vi "Gel Tugging Force Mode_Controller v16.20 EPI.vi"() -> ()   [LabVIEW 2015]
doc: "This example demonstrates how to continuously acquire voltage measurements from a DAQmx device using hardware timed, single point reads using a timed loop structure. The timed loop is controlled by the sample clock of the DAQ device. The device will read data on each tick of the sample clock. If an additional sample clock tick occurs before the current data point is read from the device or if the timed loop does not receive any sample clock ticks, a dialog will indicate that this has happened. \n\nHardware Timed Single Point acquisition works best when using a deterministic operating system (such as LabVIEW Real-Time). Because of the less deterministic nature of general purpose operating systems (such as Microsoft Windows), the software loop will not always take the exact same amount of time to execute, and this may lead to the occasional missed sample clock. \n\nFor instructions on how to connect your signals to the DAQ device, refer to your device documentation."
uses:
  <vilib>/Platform/TimedLoop/XDataNode/timing_clust.ctl
  <vilib>/Platform/TimedLoop/XDataNode/nitl_modes.ctl
  <vilib>/Platform/TimedLoop/XDataNode/wakeup.ctl
  <vilib>/dex/Flush And Wait Empty Condition.ctl
  <vilib>/DAQmx/read.llb/DAQmx Read (Analog 1D DBL NChan 1Samp).vi
  <vilib>/DAQmx/write.llb/DAQmx Write (Analog DBL 1Chan 1Samp).vi
  <vilib>/DAQmx/read.llb/DAQmx Read (Analog 2D DBL NChan NSamp).vi
  <vilib>/Analysis/baseanly.llb/Mean (DBL).vi
  <vilib>/DAQmx/create/channels.llb/DAQmx Create Channel (AI-Voltage-Basic).vi
  <vilib>/DAQmx/create/channels.llb/DAQmx Create Channel (AO-Voltage-Basic).vi
  <vilib>/DAQmx/configure/timing.llb/DAQmx Timing (Sample Clock).vi
  <vilib>/DAQmx/create/timing.llb/DAQmx Create Timing Source (Control Loop From Task).vi
  <vilib>/DAQmx/miscellaneous.llb/DAQmx Fill In Error Info.vi
  <vilib>/addons/control/pid/pid.llb/PID (DBL).vi
  <vilib>/addons/control/pid/pid.llb/PID Gain Schedule (DBL).vi
  <vilib>/platform/TimedLoop/XDataNode/XDataNode.xnode
  <vilib>/Analysis/NI_AALBase.lvlib
  <vilib>/addons/control/pid/NI_PID_pid.lvlib
  <vilib>/Platform/TimedLoop/XDataNode/XDNodeRunTimeDep.lvlib
  <vilib>/ptbypt/NI_PtbyPt.lvlib
panel:
  out "Total seconds":dbl format="%.2f"
  out "Loop Index":dbl format="%.3f"
  out "# of Data Points":i64
  out "Loop Index":i32
  out "Final AO (V)":dbl
  in  "1st OFF Length (s)":dbl=1.0
  out "Calibrating Sensor":bool
  out "Waveform Graph 2":dbl[](graph)
  in  "Ramp Total Interval (ms)":u32=490
  in  "# Ramp Steps":u32=7
  in  "7.            Step(s) Force Ramp in              (ms)?":bool=TRUE
  in  "ON":dbl=4.0
  out "DigitalTrigger":bool
  out "Corrective \nNull Flux (Gs)":dbl
  out "PID gains ON Chosen":T1
  in  "Keep Null Flux Running \n       Until Next Step? 2":bool
  in  "Start Null Flux Adjustment 2":bool=TRUE
  out "PID gains OFF Chosen":T1
  in  "Tweaked PID gains ON":T1={"proportional gain (Kc)"=0.7, "integral time (Ti, min)"=3.5e-06, "derivative time (Td, min)"=0.0}
  in  "Tweaked PID gains OFF":T1={"proportional gain (Kc)"=0.078, "integral time (Ti, min)"=3.5e-06, "derivative time (Td, min)"=0.0}
  out "Ready?":bool
  in  "4. Aggressiveness:":i32(listbox)
  out "of":i32
  in  "3. PID Parameters:":i32(listbox)
  out "ON Absolute\nFlux Setpoint (Gs)":dbl
  out "Suggested PID gains OFF":T1
  out "Suggested PID gains ON":T1
  out "Measured Magnetic Sensor 1 Zero, Mean (V)":dbl format="%_7g"
  in  "OFF (s)":dbl=7.0
  out "Round:":i32
  out "Ready?":bool
  out "Ready?":bool
  in  "Proceed with Parameters":bool=TRUE
  out "Final Flux Running at End?":bool
  out "Sensor Sensitivity \n(V/Gs)":dbl
  in  "1. Sensor:":i32(listbox)
  out "Ready?":bool
  in  "2. Needle:":i32(listbox)
  in  "Ready?&\nData Logger Running":bool
  out "Null Flux \nCurrently\nRunning?":bool
  out "Real-Time Flux Control Currently Running?":bool
  out "Ready?":bool
  out "DeGaussing?":bool
  in  "Post-Wave Null Flux Interval (s)":dbl=6.5 format="%#_13g"
  in  "Pre-Wave Null Flux Interval (s)":dbl=1.0 format="%#_13g"
  in  "6. Keep Final Flux Running at End?":bool=TRUE
  out "Flux Control Sequence Running & Uploading Data?":bool
  out "2. Null Magnetic Flux (GS):":dbl=3.5 min=-350.0 max=350.0 step=0.02 format="%#_13g"
  in  "4. Click Rocker to move to\nNext step":bool
  in  "Number of Cycles":i32=1
  in  "Flux ON relative setpoint (Gs)":dbl=-175.0 format="%#.2g"
  # "For Gel Tugging Experiments v16.20 (Controlled-Flux or Force Mode: EPI Part)"
  # "WARNING: This program crashes the first 2 or 3 times it runs after the target has been shut down. \nWARNING: Do NOT run the power supply unattended with the needle attached. Always look at the amount of current periodically."
  # "Step 0-1: Place the needle at Z ~ 7000 micron in the field of view. Inclincation Angle= 25º for HyMu80#1 Needle"
  # "(Note: Check if it is around 2.47±0.02 (V)):"
  # "Step 1: Choose Sensor & \nNeedle/PID Parameters\nfor This Experiment:"
  # "Make sure upper side of Rocker\n is pressed down before Program Starts"
  # "Step 3: Specify Control \n     Sequence Parameters:"
  # "1. Pre-Wave Null Flux Interval (s) (choose 0 if none desired):"
  # "2. Length of 2nd to end OFF"
  # "& ON"
  # "segments (s)."
  # "Length of 1st OFF"
  # "Note 1: Use Negative Flux for waves in opposite direction\nNote 2: Linear Range is (±0-175 Gs) for Null Flux + Flux ON Setpoint\nNote 3: Check ON Absolute Flux Setpoint & PID Gains on first run.\nSometimes they can be glitchy. Abort & Re-run"
  # "3. Number of OFF & ON Square-Wave Cycles:"
  # "4. Flux ON relative setpoint (Gs):"
  # "5. Post-Wave Null Flux Inteval (s) (choose 0 if none desired):"
  # "No"
  # "Yes"
  # "No"
  # "Yes"
  # "Step 4: Do you want to tweak these PID parameters?"
  # "Yes"
  # "No"
  # "vs."
  # "Step 5: Run Data Logger: Gel Tugging Force Mode_Data Logger_Auto-Manual Triggers v15.20.vi\n            Needs to be running to start the control sequence"
  # "Step 6-1: Lower the needle to the desired level for the experiment. Z ~ 3400 microns with TI-SH-U stage.\nStep 6-2: Click TRGR or Run Macro in Nikon Elements"
  # "datapoints uploaded"
  # "out of"
  # "seconds elapsed"
  # "out of"
  # "Close the VI and start over. The VI sometimes freezes upon subsequent runs"
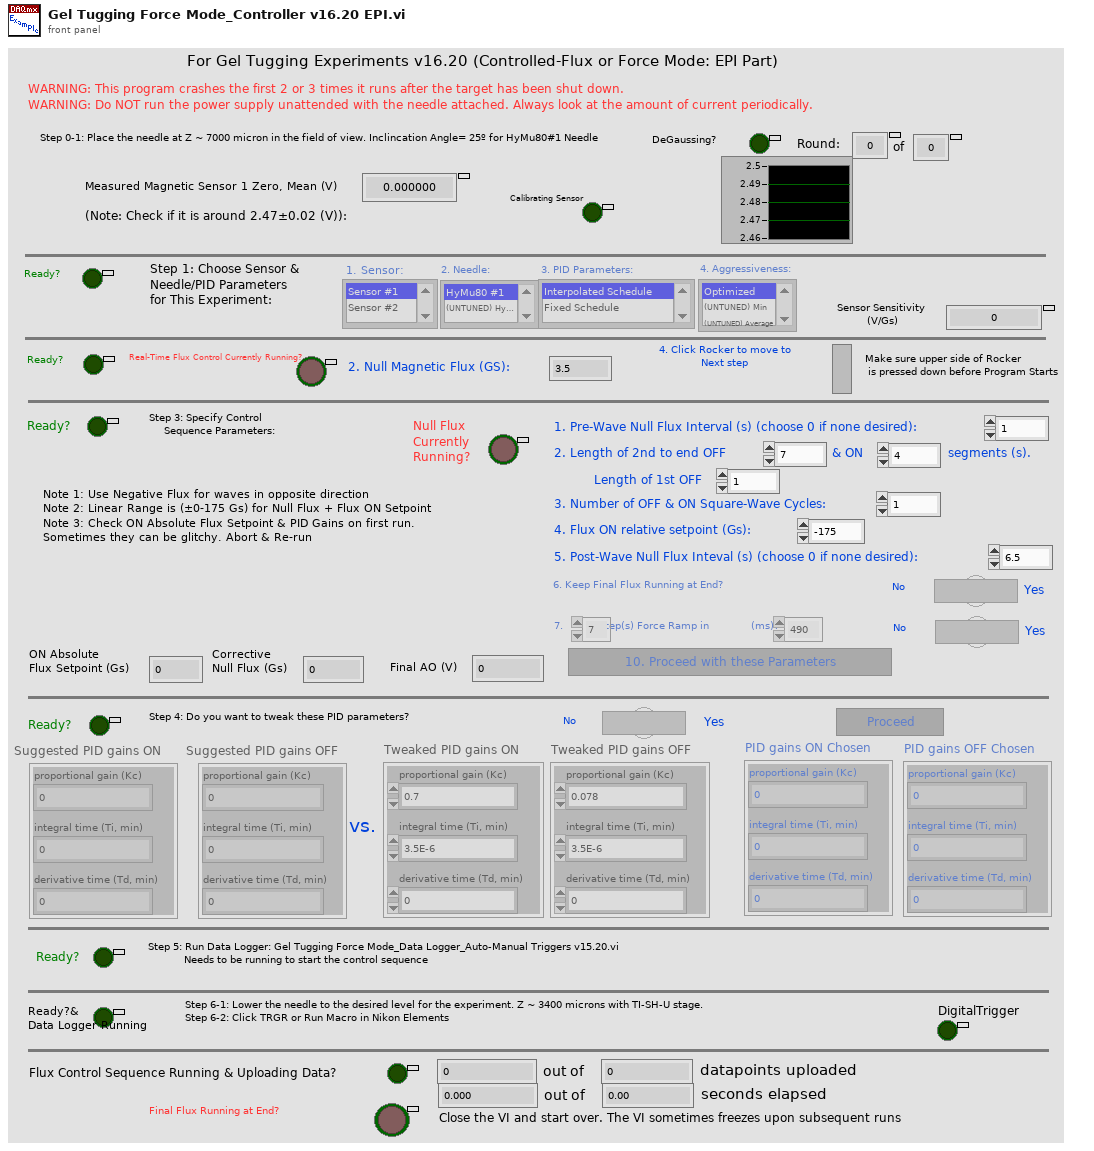
[diagram p1: front panel]
types:
  T1 = cluster{"proportional gain (Kc)":dbl, "integral time (Ti, min)":dbl, "derivative time (Td, min)":dbl}
  T2 = cluster{"PID gains":cluster{"proportional gain (Kc)":dbl, "integral time (Ti, min)":dbl, "derivative time (Td, min)":dbl}, "max value":dbl}[]
  T3 = typedef "XDNodeRunTimeDep.lvlib/timing_clust.ctl" = cluster{"Expected End [f-1]":u64, "Actual End [f-1]":u64, "Finished Late? [f-1]":bool, "Expected End [i-1]":u64, "Actual End [i-1]":u64, "Finished Late? [i-1]":bool, "Expected Start [i]":u64, "Actual Start [i]":u64, "Expected Start [f]":u64, "Actual Start [f]":u64, "Source Name":string, "Structure Name":string, "Period":i64, "Deadline":i64, "Offset":i64, "Start":i64, "Priority":i32, "Timeout":i32, "Mode":T4, "Wakeup Reason":T5, "Error":errorcluster, "Source Type":string, "Secondary Source Type":string, "Global End Time":u64, "Global Start Time":u64, "Frame Duration":u64, "Iteration Duration":u64, "Assigned CPU":i32, "I/O Scan Engine Mode":u32}
  T4 = typedef "XDNodeRunTimeDep.lvlib/nitl_modes.ctl" = enum32{"No Change", "Process missed periods, maintain original phase", "Discard missed periods, maintain original phase", "Process missed periods, ignore original phase", "Discard missed periods, ignore original phase"}
  T5 = typedef "XDNodeRunTimeDep.lvlib/wakeup.ctl" = enum32{"Normal", "Aborted", "Asynchronous wakeup", "Timing source error", "Timed loop error", "Timeout"}
  T6 = cluster{"Max/Min \ncontroller outputs":dbl, "output low":dbl}
  T7 = cluster{"PID gains":cluster{"proportional gain (Kc)":dbl, "integral time (Ti, min)":dbl, "derivative time (Td, min)":dbl}, "max value":dbl}
  T8 = typedef "Flush And Wait Empty Condition.ctl" = u8
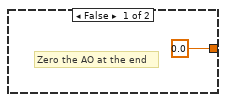
[diagram p2: hidden frame]
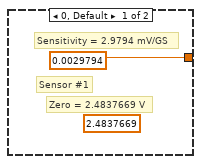
[diagram p4: hidden frame]
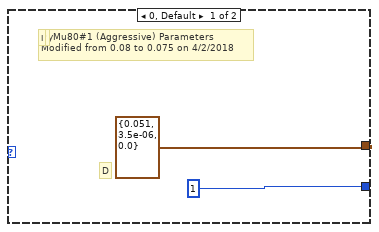
[diagram p5: hidden frame]
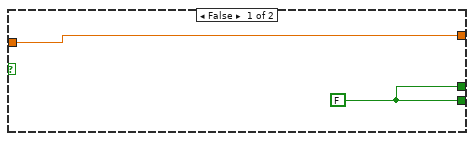
[diagram p6: hidden frame]
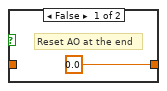
[diagram p7: hidden frame]
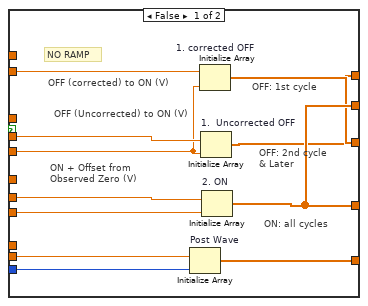
[diagram p9: hidden frame]
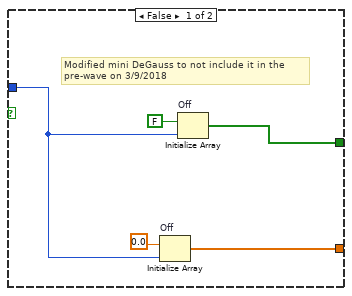
[diagram p10: hidden frame]
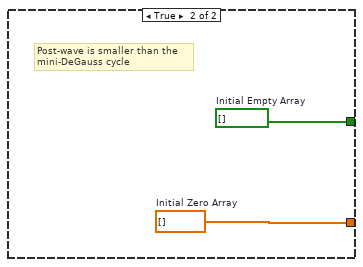
[diagram p11: hidden frame]
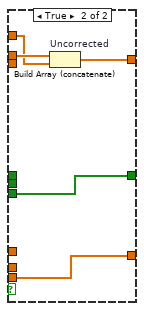
[diagram p13: hidden frame]
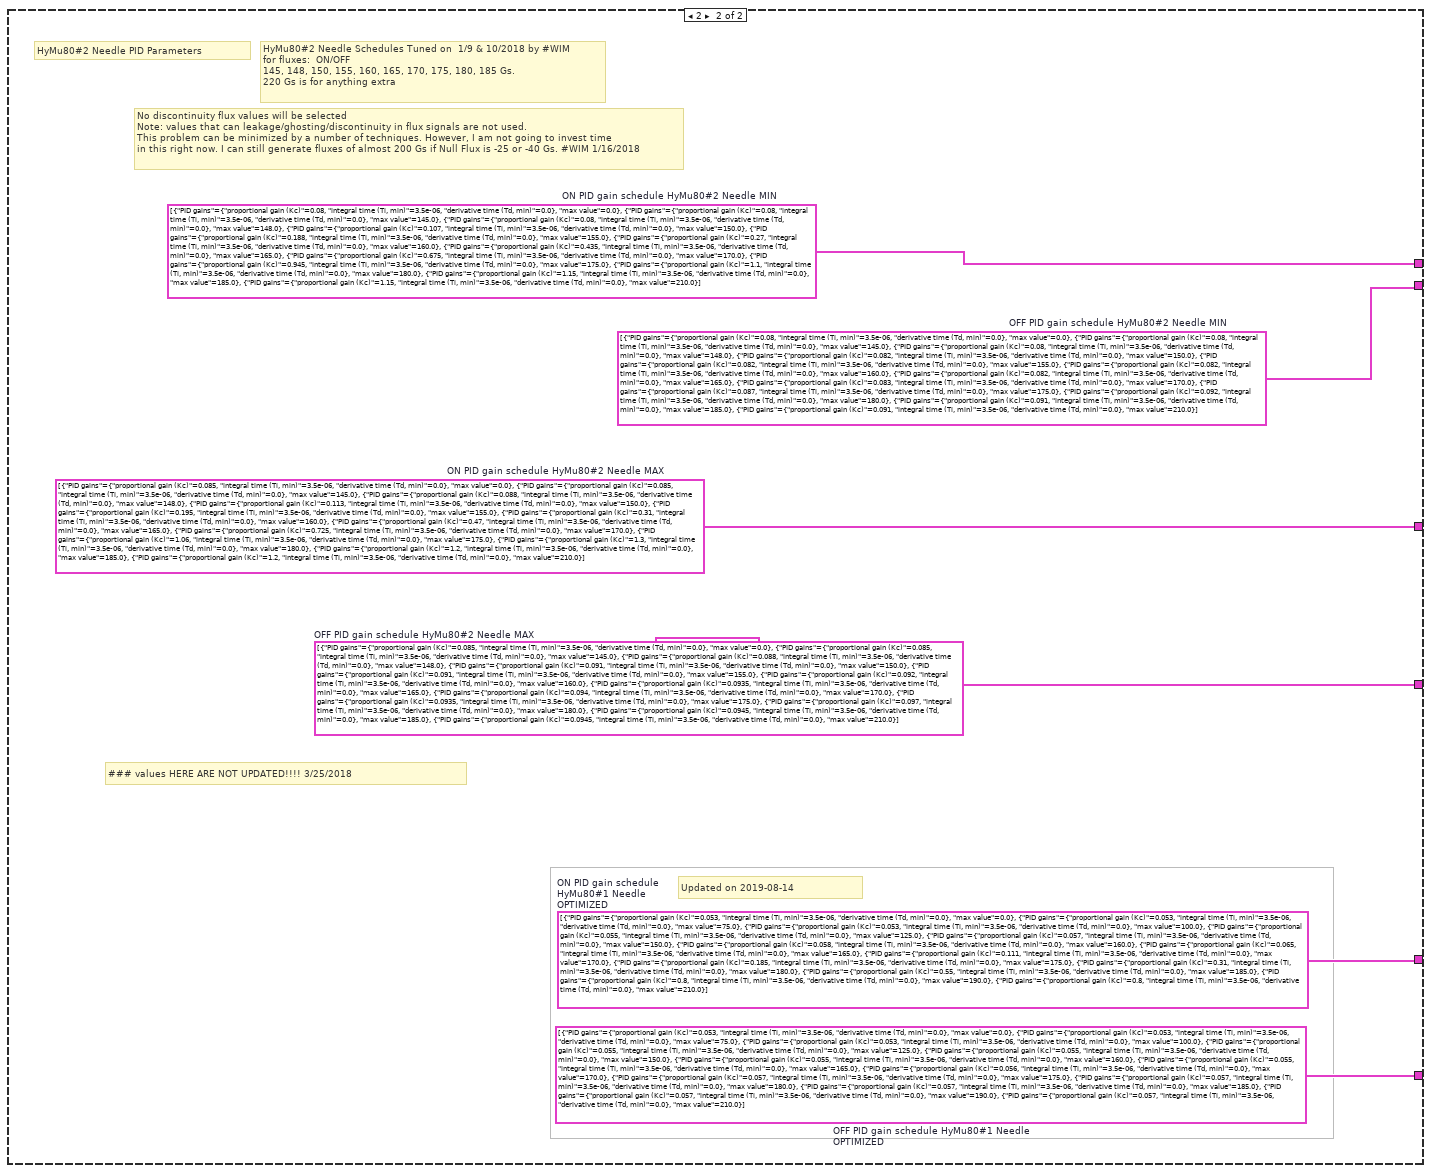
[diagram p17: hidden frame]
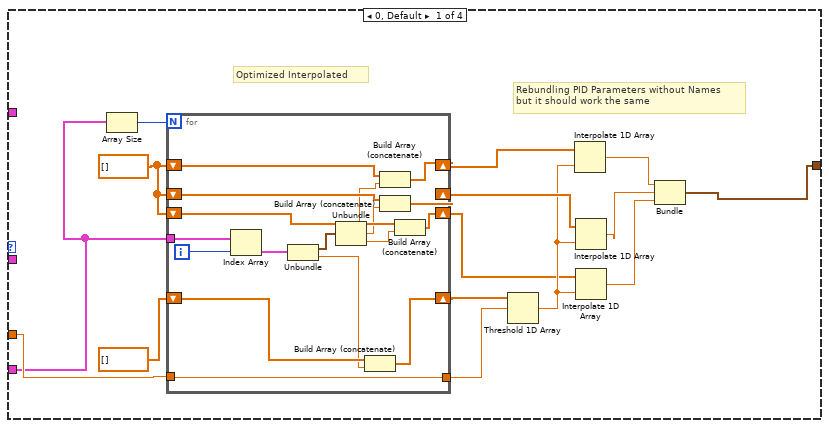
[diagram p18: hidden frame]
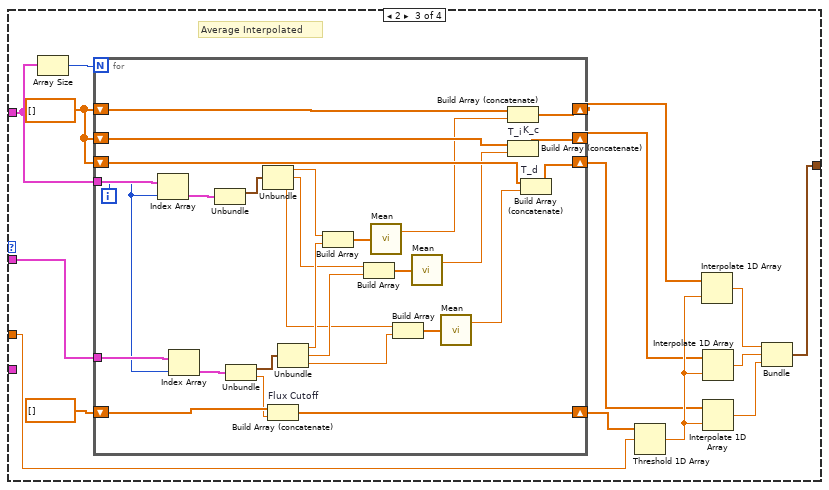
[diagram p19: hidden frame]
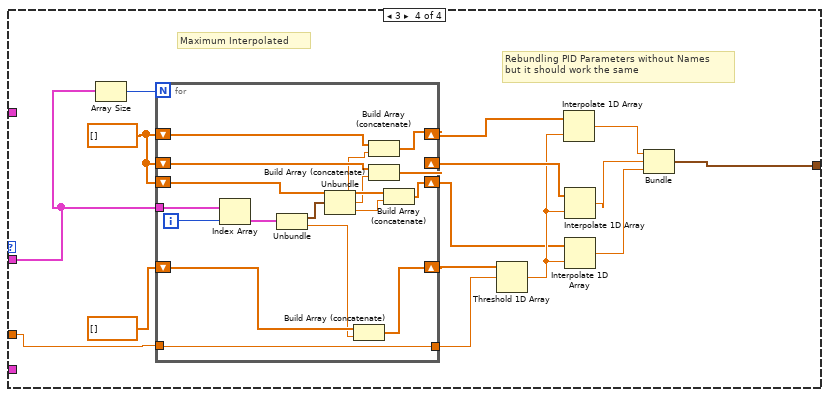
[diagram p20: hidden frame]
diagram:
  (unwired) T2 [{"PID gains"={"proportional gain (Kc)"=0.07, "integral time (Ti, min)"=3.5e-06, "derivative time (Td, min)"=0.0}, "max value"=0.0}, {"PID gains"={"proportional gain (Kc)"=0.07, "integral time (Ti, min)"=3.5e-06, "derivative time (Td, min)"=0.0}, "max value"=143.0}, {"PID gains"={"proportional gain (Kc)"=0.078, "integral time (Ti, min)"=3.5e-06, "derivative time (Td, min)"=0.0}, "max value"=148.0}, {"PID gains"={"proportional gain (Kc)"=0.078, "integral time (Ti, min)"=3.5e-06, "derivative time (Td, min)"=0.0}, "max value"=150.0}, {"PID gains"={"proportional gain (Kc)"=0.078, "integral time (Ti, min)"=3.5e-06, "derivative time (Td, min)"=0.0}, "max value"=155.0}, {"PID gains"={"proportional gain (Kc)"=0.078, "integral time (Ti, min)"=3.5e-06, "derivative time (Td, min)"=0.0}, "max value"=160.0}, {"PID gains"={"proportional gain (Kc)"=0.078, "integral time (Ti, min)"=3.5e-06, "derivative time (Td, min)"=0.0}, "max value"=165.0}, {"PID gains"={"proportional gain (Kc)"=0.078, "integral time (Ti, min)"=3.5e-06, "derivative time (Td, min)"=0.0}, "max value"=170.0}, {"PID gains"={"proportional gain (Kc)"=0.081, "integral time (Ti, min)"=3.5e-06, "derivative time (Td, min)"=0.0}, "max value"=175.0}, {"PID gains"={"proportional gain (Kc)"=0.081, "integral time (Ti, min)"=3.5e-06, "derivative time (Td, min)"=0.0}, "max value"=180.0}, {"PID gains"={"proportional gain (Kc)"=0.085, "integral time (Ti, min)"=3.5e-06, "derivative time (Td, min)"=0.0}, "max value"=185.0}, {"PID gains"={"proportional gain (Kc)"=0.086, "integral time (Ti, min)"=3.5e-06, "derivative time (Td, min)"=0.0}, "max value"=190.0}, {"PID gains"={"proportional gain (Kc)"=0.086, "integral time (Ti, min)"=0.01, "derivative time (Td, min)"=0.0}, "max value"=195.0}, {"PID gains"={"proportional gain (Kc)"=0.086, "integral time (Ti, min)"=0.01, "derivative time (Td, min)"=0.0}, "max value"=220.0}]  # OFF PID gain schedule HyMu80#1 Needle OPTIMIZED
  (unwired) T2 [{"PID gains"={"proportional gain (Kc)"=0.065, "integral time (Ti, min)"=3.5e-06, "derivative time (Td, min)"=0.0}, "max value"=0.0}, {"PID gains"={"proportional gain (Kc)"=0.065, "integral time (Ti, min)"=3.5e-06, "derivative time (Td, min)"=0.0}, "max value"=143.0}, {"PID gains"={"proportional gain (Kc)"=0.083, "integral time (Ti, min)"=3.5e-06, "derivative time (Td, min)"=0.0}, "max value"=148.0}, {"PID gains"={"proportional gain (Kc)"=0.084, "integral time (Ti, min)"=3.5e-06, "derivative time (Td, min)"=0.0}, "max value"=150.0}, {"PID gains"={"proportional gain (Kc)"=0.0875, "integral time (Ti, min)"=3.5e-06, "derivative time (Td, min)"=0.0}, "max value"=155.0}, {"PID gains"={"proportional gain (Kc)"=0.123, "integral time (Ti, min)"=3.5e-06, "derivative time (Td, min)"=0.0}, "max value"=160.0}, {"PID gains"={"proportional gain (Kc)"=0.187, "integral time (Ti, min)"=3.5e-06, "derivative time (Td, min)"=0.0}, "max value"=165.0}, {"PID gains"={"proportional gain (Kc)"=0.315, "integral time (Ti, min)"=3.5e-06, "derivative time (Td, min)"=0.0}, "max value"=170.0}, {"PID gains"={"proportional gain (Kc)"=0.46, "integral time (Ti, min)"=3.5e-06, "derivative time (Td, min)"=0.0}, "max value"=175.0}, {"PID gains"={"proportional gain (Kc)"=0.59, "integral time (Ti, min)"=3.5e-06, "derivative time (Td, min)"=0.0}, "max value"=180.0}, {"PID gains"={"proportional gain (Kc)"=0.8875, "integral time (Ti, min)"=3.5e-06, "derivative time (Td, min)"=0.0}, "max value"=185.0}, {"PID gains"={"proportional gain (Kc)"=1.04, "integral time (Ti, min)"=3.5e-06, "derivative time (Td, min)"=0.0}, "max value"=190.0}, {"PID gains"={"proportional gain (Kc)"=1.04, "integral time (Ti, min)"=0.01, "derivative time (Td, min)"=0.0}, "max value"=195.0}, {"PID gains"={"proportional gain (Kc)"=1.04, "integral time (Ti, min)"=0.01, "derivative time (Td, min)"=0.0}, "max value"=220.0}]  # ON PID gain schedule HyMu80#1 Needle OPTIMIZED
  (unwired) T2 [{"PID gains"={"proportional gain (Kc)"=0.07, "integral time (Ti, min)"=3.5e-06, "derivative time (Td, min)"=0.0}, "max value"=0.0}, {"PID gains"={"proportional gain (Kc)"=0.07, "integral time (Ti, min)"=3.5e-06, "derivative time (Td, min)"=0.0}, "max value"=116.0}, {"PID gains"={"proportional gain (Kc)"=0.078, "integral time (Ti, min)"=3.5e-06, "derivative time (Td, min)"=0.0}, "max value"=117.0}, {"PID gains"={"proportional gain (Kc)"=0.08, "integral time (Ti, min)"=3.5e-06, "derivative time (Td, min)"=0.0}, "max value"=120.0}, {"PID gains"={"proportional gain (Kc)"=0.08, "integral time (Ti, min)"=3.5e-06, "derivative time (Td, min)"=0.0}, "max value"=122.0}, {"PID gains"={"proportional gain (Kc)"=0.08, "integral time (Ti, min)"=3.5e-06, "derivative time (Td, min)"=0.0}, "max value"=125.0}, {"PID gains"={"proportional gain (Kc)"=0.08, "integral time (Ti, min)"=3.5e-06, "derivative time (Td, min)"=0.0}, "max value"=130.0}, {"PID gains"={"proportional gain (Kc)"=0.08, "integral time (Ti, min)"=3.5e-06, "derivative time (Td, min)"=0.0}, "max value"=135.0}, {"PID gains"={"proportional gain (Kc)"=0.08, "integral time (Ti, min)"=3.5e-06, "derivative time (Td, min)"=0.0}, "max value"=140.0}, {"PID gains"={"proportional gain (Kc)"=0.086, "integral time (Ti, min)"=3.5e-06, "derivative time (Td, min)"=0.0}, "max value"=145.0}, {"PID gains"={"proportional gain (Kc)"=0.096, "integral time (Ti, min)"=3.5e-06, "derivative time (Td, min)"=0.0}, "max value"=150.0}, {"PID gains"={"proportional gain (Kc)"=0.096, "integral time (Ti, min)"=3.5e-06, "derivative time (Td, min)"=0.0}, "max value"=200.0}]  # OFF PID gain schedule HyMu80#1 Needle OPTIMIZED
  (unwired) T2 [{"PID gains"={"proportional gain (Kc)"=0.07, "integral time (Ti, min)"=3.5e-06, "derivative time (Td, min)"=0.0}, "max value"=0.0}, {"PID gains"={"proportional gain (Kc)"=0.07, "integral time (Ti, min)"=3.5e-06, "derivative time (Td, min)"=0.0}, "max value"=116.0}, {"PID gains"={"proportional gain (Kc)"=0.08, "integral time (Ti, min)"=3.5e-06, "derivative time (Td, min)"=0.0}, "max value"=117.0}, {"PID gains"={"proportional gain (Kc)"=0.085, "integral time (Ti, min)"=3.5e-06, "derivative time (Td, min)"=0.0}, "max value"=120.0}, {"PID gains"={"proportional gain (Kc)"=0.115, "integral time (Ti, min)"=3.5e-06, "derivative time (Td, min)"=0.0}, "max value"=122.0}, {"PID gains"={"proportional gain (Kc)"=0.18, "integral time (Ti, min)"=3.5e-06, "derivative time (Td, min)"=0.0}, "max value"=125.0}, {"PID gains"={"proportional gain (Kc)"=0.31, "integral time (Ti, min)"=3.5e-06, "derivative time (Td, min)"=0.0}, "max value"=130.0}, {"PID gains"={"proportional gain (Kc)"=0.55, "integral time (Ti, min)"=3.5e-06, "derivative time (Td, min)"=0.0}, "max value"=135.0}, {"PID gains"={"proportional gain (Kc)"=0.95, "integral time (Ti, min)"=3.5e-06, "derivative time (Td, min)"=0.0}, "max value"=140.0}, {"PID gains"={"proportional gain (Kc)"=1.2, "integral time (Ti, min)"=3.5e-06, "derivative time (Td, min)"=0.0}, "max value"=145.0}, {"PID gains"={"proportional gain (Kc)"=1.3, "integral time (Ti, min)"=3.5e-06, "derivative time (Td, min)"=0.0}, "max value"=150.0}, {"PID gains"={"proportional gain (Kc)"=1.3, "integral time (Ti, min)"=3.5e-06, "derivative time (Td, min)"=0.0}, "max value"=200.0}]  # ON PID gain schedule HyMu80#1 Needle OPTIMIZED
  # "Note: Some quirks when running the program are: (as of 2/7/2018):\n1. First time you run it for the day, it will ask if you want to use the newer version instead of the old one already on the Remote Desktop computer\n2. Also, at the end of the first run, it will not stop. You will have to abort it. Some of the data points will be lost near the end. You might have to repeat that run.\n3. Do run the Data Reduction file or any other VIs in the DeGaussing stage. Otherwise, the program will crash."
  # "v15.20 Modified from v15.10 by Waddah Moghram on 2019-08-16 and thereafter:\n*Update based on Calibration_Core Flux Controller v11.00.vi\n\nv15.10 modified from v15.00 by  #Waddah #Moghram on 11/5/2018 and thereafter:\nTo be used with Data Logger v15.00 & Reduction v15.00: \n1. Modified it so that it can select PID gains from inside the loop\n2. Modified some PID gains at 170 Gs and higher.\n3.  Fixed the problem with the Post-wave zero Ramp 11/28/2019. WIM\n\nv 15.00 Modified from v12.00 by #Waddah #Moghram on 10/10/2018 and thereafter. To be used with Data Logger v1500 & Reduction v15.00: \n1. Replaced the Mini-DeGauss Routine with a Force Ramp (Linear vs. Steps?) since a step force function will be difficult to image-track. \n((Please refer to Linear and Step Ramps v1.00.vi for both linear and step ramps).\n*** Amount of step jump is assumed to be from ON-to-OFF and OFF-to-ON. That information is known\n2. Some of the parameters that will be used for the force ramp:\n*** Time interval: Assume that ON-to-OFF and OFF-to-ON ramps will have the same time frames.\n*** If discrete step are chosen. Choose the number of steps that it will take.\n\nv 11.00 Modified from v10.00 by #Waddah #Moghram on 4/26/2018 and thereafter. To be used with Data Logger v11.00 & Reduction v11.00: \n1. Resolve the issue of Digital Trigger automatically being released due to ground loop. Most likely due to construction that is happening around.\n* The Network digital trigger is released from the Master DAQ in the Data Logger, where it will be passed into here as a real-time global variable.\n2. For some reason, the first two runs usually crash, and the program still crashes a lot. I need to find a work around this one. \n\nv 10.00 Modified from v9.60 and v9.40 by #Waddah #Moghram on 4/4/2018 and thereafter: To be used with Data Logger v10.00 & Reduction v10.00\n1. Increased DeGauss Cycle to 2,000 milliseconds from 500 ms.\n2. Corrected the Dialog Boxes\n3. Added a switch for the Corrective Null Flux on the front panel, display it and send it to the Data Logger\n4. Corrected Mini-DeGauss Sampling Glitch where it was wired to the sampling rate directly instead of the one adjusted by the period 4/4/2018\n5. Based on a sigmoidal curve fit 4/18/2018.\nThe Equation is Y = Vmax * X^h /(K_prime + X^h), where Vmax = 10.7369, h = 1.91107, and Kprime = 3499.9. (and K_half = 71.5294))\n\n\nv 9.60 Modified from v9.50 by #Waddah #Moghram on 4/1/2018: \n1. It will correct for the Null Flux shift based on the Sigmoidal Fit that was collected from bead in front of the needle data,\nbased on a sigmoidal curve fit 4/2/2018. Experiments conducted 3/29/2018-4/2/2018. \nThe Equation is Y = Vmax * X^h /(K_prime + X^h), where Vmax = 11.4533, h = 1.69622, and Kprime = 1256.11)\n2. New Global Variable \"FluxObservedZeroGsCorrected\" to be inserted into the Data Logger v9.60\n\nv 9.50 Modified from v9.40 by #Waddah #Moghram on 3/29/2018:\n1. Used AI7 to hook up the 2nd Magnetic Sensor that will be placed in front of the sensor.\n2. Zero of 2nd Sensor is measured in the first step as well. The sensitivity is embedded in the data logger as well. \n3. Accompanies by v9.50 Data Logger.\n4. (GO BACK TO OLDER VERSION and add more details about modifications)\nFixed datapoints lost in the end due to the determinstic loop ending before the other loop. \n\nv 9.40 Modified from v9.20 by #Waddah #Moghram on 3/19/2018\n1. Removed Offset and kept amplitude +/- 10V for MiniDeGauss waveforms from inside the deterrministic loop.\n2. Shuffled the Suggested PID Loop parameters until before the \"Proceed button to allow the user to take a look at them. \n3. 3/22/2018. Reverted back to unshielded magnetic sensor, but with wire propped away from sensor.\nAlso, TI-SH-U is used and the needle is placed at Z~4600 microns for PID tuning with an inclination angle of 20 degrees\n(#OLD: 3. Re-optimized on 3/20/2018 for HyMu80#1 after shielding the sensor. The values were shifted down by 23 Gs   3/20/2018 )\n(#OLD: 4. Relocated PID Gains Selected on the front panel for more clarity 3/21/2018.)\n\nv 9.20 Modified from v9.05 and v9.10 by #Waddah #Moghram on 3/12/2018 and thereafter:\n1. It is back to OFF/ON Sequences, except first OFF segment and pre-waves have no DeGauss. It turns out to be an easy fix. \n2. Modified mini-DeGauss time \n3. Tied variables to make the wave sample properly. See notes for calculations.\n4. Turn OFF \"Null Flux Running Middle\" when control sequence starts. 3/17/2018 WIM \n5. Modified PID Parameters for #Interpolated #Optimized #HyMu80#1. Other parameters will need to be modified later on. \n6. Updated front panel to indicate inclination Angle, and Z-level for both Sensor Zero Measurement and Control Sequence.   3/18/2018\n****It turns out the PID parameters are sensitive to both z-level and inclination angle (which affect the Sensor Zero Measurement).*****\n***NOTE: First run usually does not end by itself. You will have to abort it. It will result in the loss of the last few hundred data points, but that is not too critical. Otherwise, run once, then run again. It should run smoothly every time afterwards. This is one of the quirks of working with LabVIEW. 3/18/2018\n\nv 9.05 Modified from v9.00 by #Waddah #Moghram on 3/12/2018:\n1. Modified Magnitude of Mini-DeGauss cycle from ** Maximum of (AO of Null Flux (AO_nf) or AO of ON (AO_on)) ** to **AO_nf + AO_on**\n2. The mini DeGauss oscillates about AO_nf instead of 0\n\nv 9.00 Modified from v8.40 by #Waddah #Moghram on 3/7/2018 and thereafter:\n1. It will include mini-DeGauss Cycles in the beginning of the OFF segments before PID control kicks back in. This is in an effort to minimize Magnetic Sensor hysteresis at Null Flux Observed\n(Sinusoidally Decaying Waveform Embedded in Control Sequence v1.0.vi is used for initially testing of mini-DeGauss waveforms).\n** So far, the selected waveform is about ~ 15 cycles that exponentially decay under 30 milliseconds. Used a Cosine waveform instead of sine (Sin with 90 degree phase shift).\n** Middle point is AO = 0, Magnitude between max and middle point is AO_last**    (3/12/2018)\n2. Sequence is created externally to minimize Loop calculation time. The AO Mini-DeGauss will only to be multiplied by the amplitude of the last AO out. \n3. Switched #AI6 to #AI3. Some errors with AI6 signal on the DAQ on 3/8/2018\n4. Fixed the glitch where the PID loop overreacted when the PID starts again and the Setpoint point is close to the Process variable. (Kudos to #Dr. #Selby for catching it!). on 3/8/2018\n5. Replaced \"Zero Flux\" with \"Null Flux\" for labels to avoid confusion since it is not really zero\n\nv 8.40 Modified from v8.30 by #Waddah #Moghram on 3/1/2018, and thereafter: \n1. Added a toggle to allow the re-calibration of magnetic sensor Zero or not\n2. Global Variables for DeGauss Cycles Total & Round\n3. Modified Tabbing order on 3/4/2018\n4. Fixed AO 0 initialized before PID loop to keep the value saved from \"keep Null Flux Running\" step on 3/5/2018. It was creating a blip in PID response. However, that does not seem to resolve the problem.\n\nv 8.30 Modified from v8.20 by #Waddah #Moghram on 2/22/2018:\n1. Using the measured magnetic sensor zero to create the control sequence after DeGaussing instead of the one recorded a while back inside a shielded data.\nThis is because it will change a lot over time with thermal drift and so forth. \n2. Reset the value of the sensor zero every time even no deGaussing was done.\n\nv 8.20 Modified from v8.10 by #Waddah #Moghram on 2/2/2018: \n1. This will allow the user to tweak the PID Parameters one more time before the actual experiment. This was found because it turns out that PID parameters can shift with time especially for values in the non-linear range.\n\nv. 8.10 Modified from v8.00 by #Waddah #Moghram on 1/10/2018 and thereafter:\n1. Scrapped fitted PID gains and used interpolated schedules in addition to schedules\n2. Updated PID Values for Gains and so forth.\n\nv 8.00 Modified from v7.40 by #Waddah #Moghram on 1/1/2018 and thereafter:\n1. Used the PID Gains from PID Tuning experiments \n2. Removed Normal vs. Aggressive and now will only use one set of parameters such that only one set of parameters are used\n3. Created a choice of Scheduled vs. Fitted Parameters. 1/8/2018.\n4. Fixed glitch that passed old values of waveform parameters to the global variable 1/8/2018. \n\nv 7.40 Modified from v 7.30 by #Waddah #Moghram on 12/22/2017 to including the following:\n1. Shifting the flux check and current reset only if DeGuassing Cycle required is not equal to zero. Otherwise, skip it, and keep the current running. I did this in case I need more than one run without removing the needle from the sample\n2. corrected total number of data points to allow for more than 2 seconds 1/4/2018 by #WIM\n\nv 7.30 Modified from v 7.20 by #Waddah #Moghram on 12/21/2017 to including the following:\n1. Removed Magnetic Flux Sensor Zero Calibration step, and embedded that value in the sensor section. The idea for doing that is that I want the flux values stated to be absolute. Thermal drift of sensor should not matter since PID should still work regardless of where the zero lies. Moreover, if I am accounting for the Null Flux observed, it should not matter what the absolute flux zero is.\n2. However, I kept the AO reset and used the AI2 to keep it running and also measured sensor values for 2 seconds to make sure that my values are controlled properly.\n3. Steps were re-numbered\n\nv 7.20 Modified from v7.10 by #Waddah #Moghram on 12/18/2017 to include the following:\n1. Custom-Length Waveforms. Data Reduction & Logger will be changed accordingly.\n2. Added Normal (~40 ms response time) vs. Aggressive (~22 ms response time) PID Parameters on 12/20/2017\n\nV 7.10 Modified from v7.00 by #Waddah #Moghram on 12/18/2017 to include the following:\n1. Switch order of DeGaussing & Calibrating Zero of Sensor. First Ensure that there is no residual magnetic. And secondly, reset AO just in case!\n\nv 7.00 Modified from v6.00 by #Waddah #Moghram on 12/18/2017 to include the following:\n1. Calibrated Null Flux at the beginning of the experiment without shielding to account for thermal drifts:\n*** Imported from \"01 Magnetic Sensor Zero Calibration v2.0 - Target.vi\"\n2. Included Second per Cycle\n3. Cleanup interface & Changed Step Numbers.\n\nv 6.00 Modified from v5.22 by #Waddah #Moghram on 12/5/2017 to include the following: \n1. Newer Magnetic Sensor Sensitivities: Sensor 1 is 2.9794 mV/GS and Sensor 2 is 3.0418 mV/GS\n2. Newer Magnetic Sensor Zeroes when unshielded: Sensor 1 is 2.4837669 V and Sensor 2 is 2.4928421 V\nThis program will also be used also to tune the PID in addition Magnetic Needle Choices\nOn 12/13/2017, I overhauled the interface to streamline the proceess and fixed a few glitches that allowed the program to \nchose parameters before clicking on the digital trigger\n\nv 5.22 Modified from v.5.20 by #Waddah #Moghram on 9/25/2017 to include the following:\n1. Remove prompt to calibrate the magnetic sensor and run Null Flux program\n2. Embedded the calibrated Null Flux value into the program, now that the sensor is fixed to the HyMu80 needle #1\n\n\nv5.00 modified from v.3.70 and v.4.10 by #Waddah #Moghram. It should integrate variables from both VIs.\nOther modification include:\n1. User-Defined Pre-experiment Null Flux Period\n2. User-Defined Post-experiment Null Flux Period\nModified on 8/14&15/2017 to streamline the VI even more. Ran into some Ground Loop Issues in the meantime. See Lab Notes for details.\n\nv4.10 Modified on 8/8/2017 to:\n* account for AI5 only for flux sensor values being fed to PID control.\nNotice the PID control scheme process variable is different in that it is not subtracted from the setpoint as in v.3.70 in the first PID Loop\n*modified PID parameters to the optimized ones found (subject to verification)."
  # "Re-optimized on 3/21/2018 for HyMu80#1 after shielding the sensor. The cutoff values were shifted down by ~23-27 Gs\nPreviously Optimized on 3/17/2018 for HyMu80#1 Optimized. The rest will need to be updated later\nAdded 139 Gs to keep fixed values in between 0 and 140 Gs.   Flux at 150 Gs has a response time of ~80 ms. \nAny higher PID gains will result in spike"
  # "Unshielded Previously"
  # "TOTALLY SHIELDED PARAMETERS"
  # "AI"
  # "AO"
  n1 = flat-sequence {
    tunnel: [w326] -> w96
    tunnel: [w325] -> w95
    tunnel: [w324] -> w88
    tunnel: [w323] -> w76
    tunnel: [w338] -> w103
    tunnel: w96 -> [w336]
    tunnel: w95 -> [w335]
    tunnel: w88 -> [w334]
    tunnel: [w334] -> w87
    tunnel: [w333] -> w77
    tunnel: w76 -> [w333]
    tunnel: [w348] -> w104
    tunnel: w103 -> [w348]
    tunnel: w87 -> [w347]
    tunnel: [w347] -> w86
    tunnel: [w346] -> w78
    tunnel: w77 -> [w346]
    tunnel: w104 -> [w352]
    tunnel: [w351] -> w101
    tunnel: [w350] -> w90
    tunnel: w86 -> [w350]
    tunnel: [w349] -> w79
    tunnel: w78 -> [w349]
    tunnel: [w363] -> w113
    tunnel: [w362] -> w112
    tunnel: [w361] -> w111
    tunnel: [w360] -> w102
    tunnel: w101 -> [w360]
    tunnel: w90 -> [w359]
    tunnel: [w359] -> w89
    tunnel: [w357] -> w85
    tunnel: w79 -> [w358]
    tunnel: [w358] -> w75
    tunnel: w113 -> [w406]
    tunnel: w112 -> [w405]
    tunnel: w111 -> [w404]
    tunnel: [w403] -> w107
    tunnel: [w402] -> w106
    tunnel: [w401] -> w105
    tunnel: w102 -> [w392]
    tunnel: [w390] -> w92
    tunnel: w89 -> [w390]
    tunnel: w85 -> [w389]
    tunnel: w75 -> [w388]
    tunnel: [w388] -> w73
    tunnel: [w387] -> w58
    tunnel: w107 -> [w481]
    tunnel: w106 -> [w480]
    tunnel: w105 -> [w479]
    tunnel: w92 -> [w478]
    tunnel: [w478] -> w91
    tunnel: [w477] -> w74
    tunnel: w73 -> [w477]
    tunnel: [w476] -> w59
    tunnel: w58 -> [w476]
    tunnel: [w502] -> w94
    tunnel: w91 -> [w502]
    tunnel: w74 -> [w501]
    tunnel: [w501] -> w71
    tunnel: w59 -> [w500]
    tunnel: [w500] -> w56
    tunnel: [w511] -> w100
    tunnel: [w510] -> w99
    tunnel: [w509] -> w98
    tunnel: [w508] -> w97
    tunnel: w94 -> [w507]
    tunnel: [w507] -> w93
    tunnel: [w506] -> w72
    tunnel: w71 -> [w506]
    tunnel: [w505] -> w57
    tunnel: w56 -> [w505]
    tunnel: [w504] -> w11
    tunnel: [w503] -> w10
    tunnel: [w526] -> w83
    tunnel: [w523] -> w84
    tunnel: [w671] -> w82
    tunnel: [w663] -> w81
    tunnel: w100 -> [w662]
    tunnel: w99 -> [w661]
    tunnel: w98 -> [w660]
    tunnel: w97 -> [w659]
    tunnel: [w658] -> w80
    tunnel: w93 -> [w658]
    tunnel: w72 -> [w657]
    tunnel: [w657] -> w70
    tunnel: w57 -> [w656]
    tunnel: [w656] -> w55
    tunnel: [w642] -> w50
    tunnel: [w628] -> w49
    tunnel: [w607] -> w46
    tunnel: [w601] -> w43
    tunnel: w11 -> [w528]
    tunnel: w10 -> [w597]
    tunnel: [w528] -> w1
    tunnel: w84 -> [w808]
    tunnel: [w800] -> w69
    tunnel: w83 -> [_]
    tunnel: w82 -> [w805]
    tunnel: [w804] -> w67
    tunnel: [w820] -> w65
    tunnel: w81 -> [w812]
    tunnel: [w811] -> w63
    tunnel: [w819] -> w61
    tunnel: w80 -> [w825]
    tunnel: w70 -> [w824]
    tunnel: w55 -> [w806]
    tunnel: [w806] -> w53
    tunnel: [w813] -> w52
    tunnel: w50 -> [w814]
    tunnel: w49 -> [w810]
    tunnel: [w809] -> w48
    tunnel: w46 -> [w822]
    tunnel: [w822] -> w45
    tunnel: w43 -> [w821]
    tunnel: [w821] -> w42
    tunnel: [w818] -> w9
    tunnel: [w817] -> w8
    tunnel: w1 -> [w816]
    tunnel: w69 -> [w1239]
    tunnel: [w1239] -> w68
    tunnel: w67 -> [w1238]
    tunnel: [w1238] -> w66
    tunnel: w65 -> [w1236]
    tunnel: [w1232] -> w64
    tunnel: w63 -> [w1237]
    tunnel: [w1237] -> w62
    tunnel: w61 -> [w1235]
    tunnel: [w1231] -> w60
    tunnel: [w1230] -> w54
    tunnel: w53 -> [w1230]
    tunnel: w52 -> [w1229]
    tunnel: [w1229] -> w51
    tunnel: w48 -> [w1228]
    tunnel: [w1228] -> w47
    tunnel: w45 -> [w1227]
    tunnel: [w1227] -> w44
    tunnel: w42 -> [w1226]
    tunnel: [w1226] -> w41
    tunnel: w9 -> [w1223]
    tunnel: w8 -> [w1222]
    tunnel: [w1223] -> w7
    tunnel: [w1222] -> w6
    tunnel: w68 -> [w1277]
    tunnel: [w1279] -> w40
    tunnel: [w1280] -> w38
    tunnel: [w1272] -> w36
    tunnel: [w1277] -> w34
    tunnel: [w1261] -> w33
    tunnel: [w1276] -> w32
    tunnel: w66 -> [w1269]
    tunnel: [w1269] -> w30
    tunnel: [w1273] -> w28
    tunnel: w64 -> [w1273]
    tunnel: w62 -> [w1275]
    tunnel: [w1275] -> w26
    tunnel: w60 -> [w1274]
    tunnel: [w1274] -> w25
    tunnel: w54 -> [w1270]
    tunnel: [w1270] -> w24
    tunnel: w51 -> [w1268]
    tunnel: [w1268] -> w22
    tunnel: w47 -> [w1267]
    tunnel: [w1267] -> w20
    tunnel: [w1266] -> w18
    tunnel: w44 -> [w1266]
    tunnel: w41 -> [w1265]
    tunnel: [w1265] -> w17
    tunnel: w7 -> [w1263]
    tunnel: w6 -> [w1264]
    tunnel: [w1264] -> w5
    tunnel: [w1263] -> w4
    tunnel: w40 -> [w1305]
    tunnel: [w1304] -> w39
    tunnel: w38 -> [w1307]
    tunnel: [w1306] -> w37
    tunnel: w36 -> [w1309]
    tunnel: [w1308] -> w35
    tunnel: w34 -> [w1311]
    tunnel: w33 -> [w1313]
    tunnel: w32 -> [w1331]
    tunnel: [w1330] -> w31
    tunnel: w30 -> [w1317]
    tunnel: [w1316] -> w29
    tunnel: w28 -> [w1324]
    tunnel: [w1325] -> w27
    tunnel: w26 -> [w1323]
    tunnel: w25 -> [w1327]
    tunnel: w24 -> [w1329]
    tunnel: [w1328] -> w23
    tunnel: w22 -> [w1321]
    tunnel: [w1320] -> w21
    tunnel: w20 -> [w1319]
    tunnel: [w1318] -> w19
    tunnel: w18 -> [_]
    tunnel: w17 -> [w1315]
    tunnel: [w1314] -> w16
    tunnel: [w1326] -> w15
    tunnel: [w1322] -> w14
    tunnel: [w1312] -> w13
    tunnel: [w1310] -> w12
    tunnel: w5 -> [w1303]
    tunnel: w4 -> [w1302]
    tunnel: [w1301] -> w3
    tunnel: [w1300] -> w2
    tunnel: w39 -> [w1416]
    tunnel: w37 -> [w1417]
    tunnel: w35 -> [w1413]
    tunnel: w31 -> [w1380]
    tunnel: [w1399] -> w110
    tunnel: [w1382] -> w109
    tunnel: w29 -> [w1351]
    tunnel: [w1372] -> w108
    tunnel: w27 -> [w1371]
    tunnel: w23 -> [w1363]
    tunnel: w21 -> [w1370]
    tunnel: w19 -> [w1368]
    tunnel: w16 -> [w1360]
    tunnel: w15 -> [w1376]
    tunnel: w14 -> [w1378]
    tunnel: w13 -> [w1369]
    tunnel: w12 -> [w1409]
    tunnel: w3 -> [w1356]
    tunnel: w2 -> [w1354]
    tunnel: w110 -> [w1647]
    tunnel: w109 -> [w1646]
    tunnel: w108 -> [w1648]
    frame #0 {
      (unwired) "BEFORE YOU START: \n* VERIFY these DAQ-2/Slave cables are connected as the following:\n   * AI5 is connected to Magnetic Flux \"Sensor Output - RAW\" on the Magnetic sensor box.   \n   * AI3 is connected to \"Current Sensor (1A/V)\" on the Load Box.\n   * AI7 is connected to Camera \"Exposure Sensor.\"\n   * Digital Trigger from DAQ-3/Master Output \"PF0.0\" is connected to Digital Trigger Input \"PFI0.\"\n* VERIFY these DAQ-3/Master Cables are connected as the following:\n   * Digital Trigger is connected to \"PF0.0\" BOTH \"PFI0\" on the same board and to \"PFI0\" on DAQ2/Slave.\n  \n* TURN ON power supply for half an hour. TURN ON fan control for load box (if needed).\n           WARNING: Check load is connected at the back of the load box to the back of the  power supply.\n           WARNING: Check if magnetic coil is connected to the load box if the toggle is switched to \"COIL+1OHM RESISTOR\" on the Load Box.\n           WARNING: Do NOT Position Needle in solution/cells just yet.\n           WARNING: Do NOT Position Needle in solution/cells just yet.\nIf you have not done these steps. Stop the program, then run it when ready.\n===============================\nClick OK then follow the steps"
      # "Removed the thermocouple  * AI2 is connected to Thermocouple cable."
      # "Switched Ai6 to AI3 on 3/8/2018 \nSome issues with AI6 on DEV2"
      # "1. SPECIFY the number of DeGaussing Cycle. CLICK \"Start DeGaussing.\"\n2. SPECIFY the Sensor & Needle in use for this experiment."
    }
    frame #1 {
      w114 = 0.0 ("DataRT Index")
      w120 = tag "Dev2/ai4, Dev2/ai5, Dev2/ai6, Dev2/ai7"  # AI2:Dummy,AI3: Current, AI4: Dummy,AI5:Flux, AI7: Camera  Changed Ai5 to Ai1 on 2021-04-13
      w124 = FALSE ("DeGuassing Needle")
      # "Added on 4/24/2018"
      # "RESET VARIABLES"
      n2 = shared-variable ".\\Kopco PS Project Target Variables Library.lvlib\\Data Logger Running RT"(w124) -> ()  [unwired: 1 in, 1 out]
      n3 = shared-variable "NI-GenericDesktopPC-3A84958E\\Kopco PS Project Target Variables Library.lvlib\\Needle Selection Finished"(w124) -> ()  [unwired: 1 in, 1 out]
      n4 = shared-variable "NI-GenericDesktopPC-3A84958E\\Kopco PS Project Target Variables Library.lvlib\\Control Parameters Selected"(w124) -> ()  [unwired: 1 in, 1 out]
      n5 = shared-variable "NI-GenericDesktopPC-3A84958E\\Kopco PS Project Target Variables Library.lvlib\\DeGuassing Finished"(w124) -> ()  [unwired: 1 in, 1 out]
      n6 = shared-variable "NI-GenericDesktopPC-3A84958E\\Kopco PS Project Target Variables Library.lvlib\\DeGuassing Needle"(w124) -> ()  [unwired: 1 in, 1 out]
      n7 = shared-variable "NI-GenericDesktopPC-3A84958E\\Kopco PS Project Target Variables Library.lvlib\\Null Flux Selected"(w124) -> ()  [unwired: 1 in, 1 out]
      n8 = shared-variable ".\\Kopco PS Project Target Variables Library.lvlib\\Data Upload"(w124) -> ()  [unwired: 1 in, 1 out]
      n9 = shared-variable "NI-GenericDesktopPC-3A84958E\\Kopco PS Project Target Variables Library.lvlib\\Flux RT Control"(w124) -> ()  [unwired: 1 in, 1 out]
      n10 = shared-variable "NI-GenericDesktopPC-3A84958E\\Kopco PS Project Target Variables Library.lvlib\\Flux Control Sequence Running"(w124) -> ()  [unwired: 1 in, 1 out]
      n11 = shared-variable "NI-GenericDesktopPC-3A84958E\\Kopco PS Project Target Variables Library.lvlib\\Null Flux Running Middle"(w124) -> ()  [unwired: 1 in, 1 out]
      n12 = shared-variable "NI-GenericDesktopPC-3A84958E\\Kopco PS Project Target Variables Library.lvlib\\Null Flux Running End"(w124) -> ()  [unwired: 1 in, 1 out]
      n13 = shared-variable "NI-GenericDesktopPC-3A84958E\\Kopco PS Project Target Variables Library.lvlib\\Zero Flux Calibrated Found"(w124) -> ()  [unwired: 1 in, 1 out]
      n14 = shared-variable "NI-GenericDesktopPC-3A84958E\\Kopco PS Project Target Variables Library.lvlib\\PID Parameters Selected"(w124) -> ()  [unwired: 1 in, 1 out]
      n15 = shared-variable "NI-GenericDesktopPC-3A84958E\\Kopco PS Project Target Variables Library.lvlib\\Digital Trigger"(w124) -> ()  [unwired: 1 in, 1 out]
      n16 = shared-variable ".\\Kopco PS Project Target Variables Library.lvlib\\Data Logger Running"(w124) -> ()  [unwired: 1 in, 1 out]
      n17 = shared-variable ".\\Kopco PS Project Target Variables Library.lvlib\\Data RT Flux"(w114) -> ()  [unwired: 1 in, 1 out]
      n18 = shared-variable ".\\Kopco PS Project Target Variables Library.lvlib\\Data RT Exposure"(w114) -> ()  [unwired: 1 in, 1 out]
      n19 = shared-variable ".\\Kopco PS Project Target Variables Library.lvlib\\Data RT Current"(w114) -> ()  [unwired: 1 in, 1 out]
      n20 = shared-variable ".\\Kopco PS Project Target Variables Library.lvlib\\Data RT Index"(i64 0 ("DataRT Index")) -> ()  [unwired: 1 in, 1 out]
      n21 = shared-variable ".\\Kopco PS Project Target Variables Library.lvlib\\Last Current AO"(0.0 ("Last Current AO")) -> ()  [unwired: 1 in, 1 out]
      n22 = shared-variable "NI-GenericDesktopPC-3A84958E\\Kopco PS Project Target Variables Library.lvlib\\Experiment Settings Entered"(w124) -> ()  [unwired: 1 in, 1 out]
      n23 = shared-variable "NI-GenericDesktopPC-3A84958E\\Kopco PS Project Target Variables Library.lvlib\\Sensor Zero Calibrating"(w124) -> ()  [unwired: 1 in, 1 out]
      n24 = shared-variable "NI-GenericDesktopPC-3A84958E\\Kopco PS Project Target Variables Library.lvlib\\DeGauss Round Num"(i16 0 ("DeGauss Round Num")) -> ()  [unwired: 1 in, 1 out]
      n25 = shared-variable "NI-GenericDesktopPC-3A84958E\\Kopco PS Project Target Variables Library.lvlib\\DeGauss Total"(i16 0 ("DeGauss Total")) -> ()  [unwired: 1 in, 1 out]
      n26 = shared-variable "NI-GenericDesktopPC-3A84958E\\Kopco PS Project Target Variables Library.lvlib\\Channels AI List"(w120) -> ()  [unwired: 1 in, 1 out]
      n27 = shared-variable "NI-GenericDesktopPC-3A84958E\\Kopco PS Project Target Variables Library.lvlib\\Sampling Rate"(30000.0 ("Sampling Rate")) -> ()  [unwired: 1 in, 1 out]
      n28 = shared-variable "NI-GenericDesktopPC-3A84958E\\Kopco PS Project Target Variables Library.lvlib\\Sensor Index Flux Core"(i8 1 ("Sensor Index Flux Core")) -> ()  [unwired: 1 in, 1 out]
      n29 = shared-variable "NI-GenericDesktopPC-3A84958E\\Kopco PS Project Target Variables Library.lvlib\\Sensor Index Camera"(i8 3 ("Sensor Index Flux Core")) -> ()  [unwired: 1 in, 1 out]
      n30 = shared-variable "NI-GenericDesktopPC-3A84958E\\Kopco PS Project Target Variables Library.lvlib\\Sensor Index Current"(i8 0 ("Sensor Index Flux Core")) -> ()  [unwired: 1 in, 1 out]
    }
    frame #2 {
      # "#STEP #0"
      n31 = while {
        tunnel: [w126] -> w125
        stop <- w126 stop-if-true
        w126 = TRUE ("Start DeGaussing")
      }
      n32 = shared-variable "NI-GenericDesktopPC-3A84958E\\Kopco PS Project Target Variables Library.lvlib\\DeGuassing Needle"(w125) -> ()  [unwired: 1 in, 1 out]
    }
    frame #3 {
      w127 = 0 ("1. Number of rounds")
      # "bound to \n\"DeGaussing Needle\"\nshared global variable"
      # "Bound to \n\"DeGauss Round Num\""
      # "Bound to \"DeGauss Total\""
      n33 = shared-variable "NI-GenericDesktopPC-3A84958E\\Kopco PS Project Target Variables Library.lvlib\\DeGauss Total"(w127) -> ()  [unwired: 1 in, 1 out]
      n34 = for {
        N: w127 -> [_]
        i -> [w134]
        # "Wait half a second\nbetween repititions \nto allow the system \nto stabilize\n\nAdded by WIM on \n12/18/2017\n\nUpdated to 2 Seconds\nfrom 500 ms"
        # "First Index is 0"
        n35 = Add(x=1, y=w134) -> (x+y=w128:i32)
        n36 = shared-variable "NI-GenericDesktopPC-3A84958E\\Kopco PS Project Target Variables Library.lvlib\\DeGauss Round Num"(w128) -> ()  [unwired: 1 in, 1 out]
        n37 = Wait (ms)(milliseconds to wait=u32 2000) -> ()  [unwired: 1 out]
        n38 = flat-sequence {
          tunnel: [w146] -> w143
          tunnel: [w144] -> w142
          tunnel: w128 -> [w145]
          tunnel: [w145] -> w131
          tunnel: w143 -> [w168]
          tunnel: [w175] -> w141
          tunnel: [w167] -> w140
          tunnel: [w181] -> w139
          tunnel: w142 -> [w166]
          tunnel: [w166] -> w138
          tunnel: w131 -> [w165]
          tunnel: [w165] -> w130
          tunnel: w141 -> [w198]
          tunnel: w140 -> [w199]
          tunnel: w139 -> [w206]
          tunnel: [w205] -> w137
          tunnel: [w204] -> w136
          tunnel: [w203] -> w135
          tunnel: w138 -> [w196]
          tunnel: w130 -> [w194]
          tunnel: [w194] -> w129
          tunnel: w137 -> [w241]
          tunnel: w136 -> [w240]
          tunnel: w135 -> [w236]
          tunnel: w129 -> [_]
          frame #0 {
            w147 = 5  # Time in Seconds
            w146 = 6000  # Sampling Rate (Samples/Seconds)
            # "Step 0 DeGaussing"
            # "Hardware-Time control loop cannot keep up\nwith 50,000 Hz frequence."
            n39 = Multiply(x=w147, y=w146) -> (x*y=w148:i32)
            n40 = for "A Single DeGuassing Waveform" {
              N: w148 -> [_]
              tunnel: w146 -> [w152]
              tunnel: [w149] -> w144 mode=indexing
              i -> [w151]
              (unwired) 0.3 ("y")
              w155 = 1.0  # A_0
              w158 = 1.0  # Lambda
              w162 = 0.0  # No phase
              w163 = 60.0  # Frequency, 60 Hz
              w164 = 10.0  # 4 amps = 10V
              # "Minimized 10 V to 5 V on 3/19/2018\nadd an offset of 0.3V for now"
              # "Lambda = ln(2)/(halflife time)^2"
              n41 = To Double Precision Float(number=w151) -> (double precision float=w153:dbl)
              n42 = Divide "dT"(x=w153, y=w152) -> (x/y=w150:dbl)
              n43 = Square(x=w150) -> (x^2=w156:dbl)
              n44 = Negate(x=w156) -> (-x=w157:dbl)
              n45 = call <vilib>:"Sine Wave PtByPt.vi"("time"=w150, "phase"=w162, "frequency"=w163, "amplitude"=w164) -> ("sine wave"=w161:dbl)
              n46 = Divide(x=w157, y=w158) -> (x/y=w159:dbl)
              n47 = Exponential(1:w159) -> (0:w160:dbl)
              n48 = Multiply(x=w160, y=w155) -> (x*y=w154:dbl)
              n49 = Multiply(x=w161, y=w154) -> (x*y=w149:dbl)
            }
          }
          frame #1 {
            w176 = -1 items=["default"=-1, "RSE"=10083, "NRSE"=10078, "Differential"=10106, "Pseudodifferential"=12529] ("Terminal Configuration")
            w182 = 12522 items=["Finite Samples"=10178, "Continuous Samples"=10123, "Hardware Timed Single Point"=12522]  # Sample Mode
            w189 = 10106 items=["default"=-1, "RSE"=10083, "NRSE"=10078, "Differential"=10106, "Pseudodifferential"=12529] ("Terminal Configuration")
            w192 = 12522 items=["Finite Samples"=10178, "Continuous Samples"=10123, "Hardware Timed Single Point"=12522]  # Sample Mode
            # "Step 0 DeGaussing"
            # "Power Supply Control"
            # "Magnetic Flux Sensor Signals\nOnly initiated to control \ndeterministic loop"
            n50 = call-poly <vilib>:"DAQmx Create Virtual Channel.vi"("maximum value"=5.0 ("Max Voltage"), "minimum value"=0.0 ("Min Voltage"), "input terminal configuration"=w189, "physical channels"="Dev2/ai5") -> ("task out"=w190:refnum<k21>, "error out"=w191:errorcluster)  [unwired: 10 in]
            n51 = call-poly <vilib>:"DAQmx Create Virtual Channel.vi"("maximum value"=10.0, "minimum value"=-10.0, "output terminal configuration"=w176, "physical channels"="Dev2/ao0") -> ("task out"=w186:refnum<k21>, "error out"=w185:errorcluster)  [unwired: 10 in]
            n52 = call-poly <vilib>:"DAQmx Timing.vi"("task/channels in"=w190, "sample mode"=w192, "rate"=w168, "error in"=w191) -> ("task out"=w179:refnum<k21>, "error out"=w174:errorcluster)  [unwired: 10 in]
            n53 = call "Get Terminal Name with Device Prefix.vi"("error in"=w174, "Local Terminal Name"="ai/SampleClock", "task/channels in"=w179) -> ("error out"=w173:errorcluster, "Terminal Name with Device Prefix"=w172:tag, "task out"=w175:refnum<k21>)  [unwired: 6 in]
            n54 = call-poly <vilib>:"DAQmx Timing.vi"("task/channels in"=w186, "sample mode"=w182, "rate"=w168, "source"=w172, "error in"=w185) -> ("task out"=w169:refnum<k21>, "error out"=w170:errorcluster)  [unwired: 9 in]
            n55 = call <vilib>:"DAQmx Start Task.vi"("task/channels in"=w169, "error in"=w170) -> ("task out"=w181:refnum<k21>, "error out"=w180:errorcluster)  [unwired: 12 in]
            n56 = Merge Errors(w173, w180) -> (w167:errorcluster)
          }
          frame #2 {
            # "Step 0 DeGaussing"
            n57 = call-poly <vilib>:"DAQmx Create Timing Source.vi"("task/channels in"=w198, "sleep time (us)"=1.0, "error in"=w199) -> ("task out"=w195:refnum<k21>, "timing source out"=w197:string, "error out"=w193:errorcluster)  [unwired: 10 in]
            n58 = node-c288(w197, w193) -> (w202:T3)  [unwired: 8 in]
            n59 = timed-loop "DeGuassing Control" {
              tunnel: w195 -> [w225]
              tunnel: [w218] -> w204
              tunnel: w206 -> [w208]
              tunnel: [w223] -> w203
              tunnel: w193 -> [w222]
              tunnel: [w221] -> w205
              timing: w202 -> [_]
              timing-out: [_] -> w201
              tunnel: w196 -> [w210]
              i -> [w214]
              stop <- w207 continue-if-true
              # "PS does not turn off unless two values are written."
              # "Offset by 1 to eliminate\nextra datapoint at end"
              n60 = node-c288() -> ()  [unwired: 1 in, 1 out]
              n61 = Array Size(array=w210) -> (size(s)=w215:i32)
              n62 = Index Array "Index Array"(array=w210, index=w214) -> (element=w211:dbl)
              n63 = call-poly <vilib>:"DAQmx Read.vi"("task/channels in"=w225, "error in"=w222) -> ("task out"=w218:refnum<k21>, "error out"=w224:errorcluster)  [unwired: 11 in, 1 out]
              n64 = Less?(x=w214, y=w215) -> (x < y?=w213:bool)
              n65 = Subtract(x=w215, y=10) -> (x-y=w217:i32)
              n66 = Less?(x=w214, y=w217) -> (x < y?=w212:bool)
              n67 = case shown="True" w212 {
                tunnel: [0.0 ("output") w228] -> w209
                tunnel: w211 -> [_ w228]
                frame False {
                  # "Zero the AO at the end"
                }
                frame True {
                }
              }
              n68 = call-poly <vilib>:"DAQmx Write.vi"("task/channels in"=w208, "data"=w209, "error in"=w224) -> ("task out"=w223:refnum<k21>, "error out"=w221:errorcluster)  [unwired: 10 in, 1 out]
              n69 = Unbundle By Name(w221) -> ("status"=w226:bool)  [unwired: 2 out]
              n70 = Not Or(1:FALSE ("Stop"), 2:w226) -> (0:w219:bool)
              n71 = And(x=w219, y=w213) -> (x .and. y?=w207:bool)
              n72 = shared-variable "NI-GenericDesktopPC-3A84958E\\Kopco PS Project Target Variables Library.lvlib\\DeGuassing Needle"(w207) -> ()  [unwired: 1 in, 1 out]
              n73 = node-c288() -> ()  [unwired: 1 in, 1 out]
            }
            n74 = node-c288(w201) -> ()  [unwired: 1 out]
          }
          frame #3 {
            n75 = call <vilib>:"DAQmx Stop Task.vi"("task/channels in"=w240, "error in"=w241) -> ("task out"=w243:refnum<k21>, "error out"=w242:errorcluster)  [unwired: 12 in]
            n76 = call <vilib>:"DAQmx Clear Task.vi"("task in"=w243, "error in"=w242) -> ("error out"=w237:errorcluster)  [unwired: 13 in]
            n77 = call <vilib>:"DAQmx Stop Task.vi"("task/channels in"=w236, "error in"=w237) -> ("task out"=w239:refnum<k21>, "error out"=w238:errorcluster)  [unwired: 12 in]
            n78 = call <vilib>:"DAQmx Clear Task.vi"("task in"=w239, "error in"=w238) -> ()  [unwired: 13 in, 1 out]
          }
        }
      }
    }
    frame #4 {
      # "Step 0 Reset the Magnetic Sensor"
      n79 = case shown="True" FALSE ("Measure Flux Sensor Zero?") {
        frame False {
        }
        frame True {
          w252 = 12522 items=["Finite Samples"=10178, "Continuous Samples"=10123, "Hardware Timed Single Point"=12522] ("sample mode")
          w266 = 3.0  # Time (s)
          w265 = 10000  # Samples read  per loop
          w285 = -1 items=["default"=-1, "RSE"=10083, "NRSE"=10078, "Differential"=10106, "Pseudodifferential"=12529] ("Terminal Configuration")
          w282 = 12522 items=["Finite Samples"=10178, "Continuous Samples"=10123, "Hardware Timed Single Point"=12522]  # Sample Mode
          w274 = 10106 items=["Default"=-1, "RSE"=10083, "NRSE"=10078, "Differential"=10106, "Pseudodifferential"=12529]  # input terminal configuration
          w277 = 0
          # "Changed on 3/29/2018 to include Sensor 2 placed in front of the needle. Added Global Variable \"Flux Calibrated Zero 2\""
          # "Reset AO to 0. Sometimes it overshoot after DeGaussing\nAdded by #WIM on 12/18/2017"
          # "Power Supply Control"
          n80 = shared-variable "NI-GenericDesktopPC-3A84958E\\Kopco PS Project Target Variables Library.lvlib\\Channels AI List"() -> (w268:string)  [unwired: 1 in, 1 out]
          n81 = shared-variable "NI-GenericDesktopPC-3A84958E\\Kopco PS Project Target Variables Library.lvlib\\Sampling Rate"() -> (w247:dbl)  [unwired: 1 in, 1 out]
          n82 = call-poly <vilib>:"DAQmx Create Virtual Channel.vi"("maximum value"=5.0, "minimum value"=0.0, "input terminal configuration"=w274, "physical channels"=w268) -> ("task out"=w248:refnum<k21>, "error out"=w249:errorcluster)  [unwired: 10 in]
          n83 = call-poly <vilib>:"DAQmx Create Virtual Channel.vi"("maximum value"=10.0, "minimum value"=-10.0, "output terminal configuration"=w285, "physical channels"="Dev2/ao0") -> ("task out"=w279:refnum<k21>, "error out"=w280:errorcluster)  [unwired: 10 in]
          n84 = call-poly <vilib>:"DAQmx Timing.vi"("task/channels in"=w248, "sample mode"=w252, "rate"=w247, "error in"=w249) -> ("task out"=w251:refnum<k21>, "error out"=w250:errorcluster)  [unwired: 10 in]
          n85 = Multiply "Total Samples \nper Channel"(x=w247, y=w266) -> (x*y=w267:dbl)
          n86 = call "Get Terminal Name with Device Prefix.vi"("error in"=w250, "Local Terminal Name"="ai/SampleClock", "task/channels in"=w251) -> ("error out"=w262:errorcluster, "Terminal Name with Device Prefix"=w261:tag, "task out"=w257:refnum<k21>)  [unwired: 6 in]
          n87 = call-poly <vilib>:"DAQmx Timing.vi"("task/channels in"=w279, "sample mode"=w282, "rate"=w247, "source"=w261, "error in"=w280) -> ("task out"=w287:refnum<k21>, "error out"=w286:errorcluster)  [unwired: 9 in]
          n88 = call <vilib>:"DAQmx Start Task.vi"("task/channels in"=w287, "error in"=w286) -> ("task out"=w290:refnum<k21>, "error out"=w289:errorcluster)  [unwired: 12 in]
          n89 = Merge Errors(w262, w289) -> (w255:errorcluster)
          n90 = Subtract "Almost Total"(x=w267, y=w265) -> (x-y=w264:dbl)
          n91 = shared-variable "NI-GenericDesktopPC-3A84958E\\Kopco PS Project Target Variables Library.lvlib\\Sensor Index Flux Core"() -> (w246:i8)  [unwired: 1 in, 1 out]
          n92 = call-poly <vilib>:"DAQmx Create Timing Source.vi"("task/channels in"=w257, "sleep time (us)"=1.0, "error in"=w255) -> ("task out"=w258:refnum<k21>, "timing source out"=w253:string, "error out"=w256:errorcluster)  [unwired: 10 in]
          n93 = Initialize Array(w277, w277) -> (w270:i32[])
          n94 = node-c288(w253) -> (w260:T3)  [unwired: 3 in]
          n95 = timed-loop {
            tunnel: w258 -> [w311]
            tunnel: w256 -> [w306]
            tunnel: [w312] -> w294
            shift-right: [w313] -> _
            shift-left: 0 -> [w314]
            tunnel: [w310] -> w288
            shift-right: [w308] -> w245
            shift-left: w270 -> [w303]
            tunnel: [w303] -> _
            tunnel: w290 -> [w307]
            tunnel: [w302] -> w295
            tunnel: w265 -> [w300]
            tunnel: w264 -> [w299]
            timing: w260 -> [_]
            timing-out: [_] -> w259
            shift-right: [w298] -> _
            shift-left: _ -> [_]
            tunnel: w246 -> [w296]
            i -> [w298]
            stop <- w297 continue-if-true
            w315 = 10.0  # timeout
            # "Magnetic Sensor 2"
            # "Magnetic Sensor 1"
            n96 = node-c288() -> ()  [unwired: 1 in, 1 out]
            n97 = call-poly <vilib>:"DAQmx Write.vi"("task/channels in"=w307, "data"=0.0, "error in"=w306) -> ("task out"=w302:refnum<k21>, "error out"=w305:errorcluster)  [unwired: 10 in, 1 out]
            n98 = call-poly <vilib>:"DAQmx Read.vi"("task/channels in"=w311, "number of samples per channel"=w300, "timeout"=w315, "error in"=w305) -> ("task out"=w310:refnum<k21>, "data"=w301:dbl[][], "error out"=w312:errorcluster)  [unwired: 9 in]
            n99 = Add(x=w314, y=w300) -> (x+y=w313:i32)
            n100 = Unbundle By Name(w312) -> ()  [unwired: 1 out]
            n101 = Less Or Equal?(x=w313, y=w299) -> (x <= y?=w297:bool)
            n102 = Delete From Array(array=w301, index (row)=w296) -> (deleted portion=w309:dbl[])  [unwired: 2 in, 1 out]
            n103 = shared-variable "NI-GenericDesktopPC-3A84958E\\Kopco PS Project Target Variables Library.lvlib\\Sensor Zero Calibrating"(w297) -> ()  [unwired: 1 in, 1 out]
            n104 = Build Array (concatenate)(w303, w309) -> (w308:dbl[])
            n105 = node-c288() -> ()  [unwired: 1 in, 1 out]
          }
          "Waveform Graph 2" <- w245
          n106 = node-c288(w259) -> ()  [unwired: 1 out]
          n107 = call <vilib>:"Std Deviation and Variance.vi"("X"=w245) -> ("mean"=w271:dbl)  [unwired: 1 in, 2 out]
          n108 = call <vilib>:"DAQmx Stop Task.vi"("task/channels in"=w295, "error in"=w294) -> ("task out"=w291:refnum<k21>, "error out"=w292:errorcluster)  [unwired: 12 in]
          n109 = shared-variable "NI-GenericDesktopPC-3A84958E\\Kopco PS Project Target Variables Library.lvlib\\Zero Flux Calibrated Core"(w271) -> ()  [unwired: 1 in, 1 out]
          n110 = call <vilib>:"DAQmx Clear Task.vi"("task in"=w291, "error in"=w292) -> ("error out"=w293:errorcluster)  [unwired: 13 in]
          n111 = call <vilib>:"DAQmx Stop Task.vi"("task/channels in"=w288, "error in"=w293) -> ("task out"=w276:refnum<k21>, "error out"=w275:errorcluster)  [unwired: 12 in]
          n112 = call <vilib>:"DAQmx Clear Task.vi"("task in"=w276, "error in"=w275) -> ("error out"=w269:errorcluster)  [unwired: 13 in]
          n113 = call <vilib>:"General Error Handler.vi"("error in (no error)"=w269) -> ()  [unwired: 10 in, 5 out]
        }
      }
    }
    frame #5 {
      # "Bound to \"Flux Calibrated Zero 2\" \nglobal Variable"
      # "Bound to \"Flux Calibrated Zero\" \nglobal Variable"
      # "Bound to \"DeGaussing Finished\""
      # "Ensure that the correct value is displayed\n(2.49±0.05 (V))"
      n114 = shared-variable "NI-GenericDesktopPC-3A84958E\\Kopco PS Project Target Variables Library.lvlib\\DeGuassing Finished"(TRUE ("DeGuassing Finished")) -> ()  [unwired: 1 in, 1 out]
    }
    frame #6 {
      # "Bound to \"Needle Selection Finished\" \nshared global variable."
      # "Step 1 Selecting Needle & Sensor\n& PID Parameters"
      n115 = while {
        tunnel: [w332] -> w327
        tunnel: ["2. Needle:"] -> w326
        tunnel: ["1. Sensor:"] -> w325
        tunnel: ["3. PID Parameters:"] -> w324
        tunnel: ["4. Aggressiveness:"] -> w323
        stop <- w332 stop-if-true
        w332 = TRUE ("Proceed with Selection")
        # "Added on 1/16/2018"
      }
      n116 = shared-variable "NI-GenericDesktopPC-3A84958E\\Kopco PS Project Target Variables Library.lvlib\\Needle Selection Finished"(w327) -> ()  [unwired: 1 in, 1 out]
    }
    frame #7 {
      # "Step 1 Selecting Needle & Sensor\n& PID Parameters"
      # "1/5/2018\nGot rid of \"normal\" PID Gains, Only kept Aggressive..\n\nFrom now on, that name will be dropped."
      # "Needle Used no needed so far\nbut might be used in future versinos\n12/20/2017"
      # "More precisely measured Magnetic Sensor value for Sensors 1 & 2 on 11/28/2017"
      # "Older Magnetic Sensitivity Measured before 11/2017 for Sensor 2 very crudely\n0.003112 V/GS.\nPreviously sensor 2 zero was 2.4942892 V based on 10-minute experiments on 7/12/2017"
      # "Coupled with Shared Variable Sensor 1"
      n117 = case shown="1" w336 {
        tunnel: [T1 {"proportional gain (Kc)"=0.051, "integral time (Ti, min)"=3.5e-06, "derivative time (Td, min)"=0.0} ("PID gains HyMu80 #1 (Aggressive)") T1 {"proportional gain (Kc)"=0.051, "integral time (Ti, min)"=3.5e-06, "derivative time (Td, min)"=0.0} ("PID gains HyMu80 #2 (Aggressive)")] -> w338
        tunnel: [i8 1 ("Needle Used") i8 2 ("Needle Used")] -> w339
        frame 0, Default {
          # "HyMu80#1 (Aggressive) Parameters\nModified from 0.08 to 0.075 on 4/2/2018"
          # "D"
          # "I"
          # "P"
        }
        frame 1 {
          # "D"
          # "I"
          # "P"
        }
      }
      n118 = case shown="1" w335 {
        tunnel: [0.0029794 0.0030418] -> w337
        frame 0, Default {
          (unwired) 2.4837669
          # "Zero = 2.4837669 V"
          # "Sensor #1"
          # "Sensitivity = 2.9794 mV/GS"
        }
        frame 1 {
          (unwired) 2.4928421
          # "Zero = 2.4928421 V"
          # "Sensor #2"
          # "Sensor 2 = 3.0418 mV/GS"
        }
      }
      n119 = shared-variable "NI-GenericDesktopPC-3A84958E\\Kopco PS Project Target Variables Library.lvlib\\Sensor Sensitivity Core"(w337) -> ()  [unwired: 1 in, 1 out]
      n120 = shared-variable "NI-GenericDesktopPC-3A84958E\\Kopco PS Project Target Variables Library.lvlib\\Needle Used"(w339) -> ()  [unwired: 1 in, 1 out]
    }
    frame #8 {
      (unwired) "1. SET-UP & RUN \"LIVE-FAST\" image acquisition in Nikon Elements. \n2. POSITION the magnetic needle in the glycerol sample within 100 micron of several beads. (Please refer to latest calibration protocol for more details). \n3. Click OK then follow the Steps 3:\n      1. CLICK \"Start Null Flux Adjustment.\"\n      2. Adjust the Magnetic Flux until beads are no longer attacted to the needle.\n      3. Select if you want the flux to stay running until the control sequence is used in Step 4\n      3. CLICK \"FINISH Null Flux Adjustment?\" to Move to Step 4 \n"  # 1. SET-UP & RUN "LIVE-FAST" image acquisition in Nikon Elements.  2. POSITION the magnetic needle in the glycerol sample within 100 micron of several beads. (Please refer to latest calibration protocol for more details).  3. Click OK then follow the Steps 3:       1. CLICK "Start Null Flux Adjustment."       2. Adjust the Magnetic Flux until beads are no longer attacted to the needle.       3. Select if you want the flux to stay running until the control sequence is used in Step 4       3. CLICK "FINISH Null Flux Adjustment?" to Move to Step 4
    }
    frame #9 {
      # "Bound to \"Flux RT Control\" \nglobal shared variable?"
      # "Step 2 Finding Null Flux in Real Time"
      n121 = while {
        tunnel: [w355] -> w353
        tunnel: [w354] -> w351
        tunnel: w352 -> [w354]
        stop <- w355 stop-if-true
        w355 = TRUE ("Start Null Flux Adjustment")
      }
      n122 = shared-variable "NI-GenericDesktopPC-3A84958E\\Kopco PS Project Target Variables Library.lvlib\\Flux RT Control"(w353) -> ()  [unwired: 1 in, 1 out]
    }
    frame #10 {
      w370 = -1 items=["default"=-1, "RSE"=10083, "NRSE"=10078, "Differential"=10106, "Pseudodifferential"=12529] ("Terminal Configuration")
      w375 = 12522 items=["Finite Samples"=10178, "Continuous Samples"=10123, "Hardware Timed Single Point"=12522]  # Sample Mode
      w381 = 10106 items=["default"=-1, "RSE"=10083, "NRSE"=10078, "Differential"=10106, "Pseudodifferential"=12529] ("Terminal Configuration")
      w384 = 12522 items=["Finite Samples"=10178, "Continuous Samples"=10123, "Hardware Timed Single Point"=12522]  # Sample Mode
      # "Step 2 Finding Null Flux in Real Time"
      # "Hardware-Time control loop cannot keep up\nwith 50,000 Hz frequence."
      # "Power Supply Control"
      # "Magnetic Flux Sensor Signals\nRelayed over three channels."
      n123 = shared-variable "NI-GenericDesktopPC-3A84958E\\Kopco PS Project Target Variables Library.lvlib\\Channels AI List"() -> (w356:string)  [unwired: 1 in, 1 out]
      n124 = shared-variable "NI-GenericDesktopPC-3A84958E\\Kopco PS Project Target Variables Library.lvlib\\Sampling Rate"() -> (w357:dbl)  [unwired: 1 in, 1 out]
      n125 = call-poly <vilib>:"DAQmx Create Virtual Channel.vi"("maximum value"=5.0 ("Max Voltage"), "minimum value"=0.0 ("Min Voltage"), "input terminal configuration"=w381, "physical channels"=w356) -> ("task out"=w382:refnum<k21>, "error out"=w383:errorcluster)  [unwired: 10 in]
      n126 = call-poly <vilib>:"DAQmx Create Virtual Channel.vi"("maximum value"=10.0, "minimum value"=-10.0, "output terminal configuration"=w370, "physical channels"="Dev2/ao0") -> ("task out"=w378:refnum<k21>, "error out"=w377:errorcluster)  [unwired: 10 in]
      n127 = call-poly <vilib>:"DAQmx Timing.vi"("task/channels in"=w382, "sample mode"=w384, "rate"=w357, "error in"=w383) -> ("task out"=w373:refnum<k21>, "error out"=w369:errorcluster)  [unwired: 10 in]
      n128 = call "Get Terminal Name with Device Prefix.vi"("error in"=w369, "Local Terminal Name"="ai/SampleClock", "task/channels in"=w373) -> ("error out"=w366:errorcluster, "Terminal Name with Device Prefix"=w368:tag, "task out"=w363:refnum<k21>)  [unwired: 6 in]
      n129 = call-poly <vilib>:"DAQmx Timing.vi"("task/channels in"=w378, "sample mode"=w375, "rate"=w357, "source"=w368, "error in"=w377) -> ("task out"=w365:refnum<k21>, "error out"=w364:errorcluster)  [unwired: 9 in]
      n130 = call <vilib>:"DAQmx Start Task.vi"("task/channels in"=w365, "error in"=w364) -> ("task out"=w361:refnum<k21>, "error out"=w374:errorcluster)  [unwired: 12 in]
      n131 = Merge Errors(w366, w374) -> (w362:errorcluster)
    }
    frame #11 {
      w398 = 30  # # of samples pushed to PID loop
      # "Bound to \"Null Flux Running Middle\" \nshared global variable."
      # "Bound to \"Null Flux Selected\"\nshared global variable"
      # "Step 2 Finding Null Flux in Real Time"
      # "Step 2 Finding Null Flux in Real Time"
      # "12/13/2017. Cannot turn on flux control sequence inside Real-time loop. That is why I have used the trigger in the Datalogger to turn th is on. \nOtherwise, it will remain off"
      # "PID is 30 times slower"
      n132 = shared-variable "NI-GenericDesktopPC-3A84958E\\Kopco PS Project Target Variables Library.lvlib\\Zero Flux Observed Gs Corrected"() -> (w385:dbl)  [unwired: 1 in, 1 out]
      "2. Null Magnetic Flux (GS):" <- w385
      n133 = shared-variable "NI-GenericDesktopPC-3A84958E\\Kopco PS Project Target Variables Library.lvlib\\Zero Flux Calibrated Core"() -> (w393:dbl)  [unwired: 1 in, 1 out]
      n134 = shared-variable "NI-GenericDesktopPC-3A84958E\\Kopco PS Project Target Variables Library.lvlib\\Sensor Sensitivity Core"() -> (w391:dbl)  [unwired: 1 in, 1 out]
      n135 = call-poly <vilib>:"DAQmx Create Timing Source.vi"("task/channels in"=w406, "sleep time (us)"=1.0, "error in"=w405) -> ("task out"=w412:refnum<k21>, "timing source out"=w409:string, "error out"=w410:errorcluster)  [unwired: 10 in]
      n136 = shared-variable "NI-GenericDesktopPC-3A84958E\\Kopco PS Project Target Variables Library.lvlib\\Sensor Index Flux Core"() -> (w386:i8)  [unwired: 1 in, 1 out]
      n137 = Reciprocal(x=w389) -> (1/x=w400:dbl)
      n138 = Multiply(x=w398, y=w400) -> (x*y=w399:dbl)
      n139 = Initialize Array "Initialize Array"(0, 0 ("level 3 duration 0.1ms")) -> (w407:i32[])
      n140 = node-c288(w409, w410) -> (w416:T3)  [unwired: 8 in]
      n141 = timed-loop {
        tunnel: w412 -> [w446]
        tunnel: [w441] -> w403
        tunnel: w404 -> [w445]
        tunnel: [w443] -> w402
        tunnel: w410 -> [w442]
        tunnel: [w432] -> w401
        timing: w416 -> [_]
        timing-out: [_] -> w415
        shift-right: [w428] -> _
        shift-left: 0 -> [w438]
        shift-right: [w435] -> _
        shift-left: w407 -> [w436]
        tunnel: w398 -> [w426]
        tunnel: w399 -> [w425]
        tunnel: w393 -> [w424]
        tunnel: w391 -> [w423]
        tunnel: [w417] -> w397
        tunnel: [w422] -> _
        tunnel: [w422] -> w396
        tunnel: [w421] -> w395
        tunnel: w392 -> [w420]
        tunnel: [w419] -> w387
        tunnel: w386 -> [w418]
        tunnel: w385 -> [w417]
        stop <- w422 continue-if-true
        # "Observed Flux (V)"
        # "Keep this control inside the loop so that changed in \nreal time under live imaging"
        # "Flux Sensor Calibrated Zero value (V)"
        n142 = node-c288() -> ()  [unwired: 1 in, 1 out]
        n143 = call-poly <vilib>:"DAQmx Read.vi"("task/channels in"=w446, "error in"=w442) -> ("task out"=w441:refnum<k21>, "data"=w433:dbl[], "error out"=w444:errorcluster)  [unwired: 11 in]
        n144 = Delete From Array "Choose 1st Channel"(array=w433, index=w418) -> (deleted portion=w437:dbl)  [unwired: 1 in, 1 out]
        n145 = Build Array (concatenate) "AI Array"(w437, w436) -> (w434:dbl[])
        n146 = Array Size(array=w434) -> (size(s)=w440:i32)
        n147 = Equal?(x=w440, y=w426) -> (x = y?=w439:bool)
        n148 = Multiply(x=w417, y=w423) -> (x*y=w427:dbl)
        n149 = Add "Zero Offset"(x=w424, y=w427) -> (x+y=w431:dbl)
        n150 = case shown="True" w439 {
          tunnel: w425 -> [_ w459]
          tunnel: w431 -> [_ w464]
          tunnel: [w457 w462] -> w428
          tunnel: w438 -> [w457 _]
          tunnel: w434 -> [w456 w461]
          tunnel: [w456 w460] -> w435
          tunnel: w420 -> [_ w458]
          frame False {
          }
          frame True {
            # "Max/Min controller outputs"
            n151 = call-poly <vilib>:"Mean.vi"("X"=w461) -> ("mean"=w463:dbl)  [unwired: 1 out]
            n152 = call-poly <vilib>:"PID.vi"("reinitialize? (F)"=FALSE, "output range"=cluster{"output high":dbl, "output low":dbl} {"output high"=10.0, "output low"=-10.0}, "dt (s)"=w459, "PID gains"=w458, "process variable"=w463, "setpoint"=w464) -> ("output"=w462:dbl)  [unwired: 4 in, 1 out]
            n153 = Initialize Array(0, 0) -> (w460:i32[])
          }
        }
        n154 = case shown="True" "4. Click Rocker to move to\nNext step" {
          tunnel: [w448 TRUE ("y")] -> w429
          tunnel: [w449 w451] -> w419
          tunnel: w428 -> [w449 w452]
          tunnel: [w448 w450] -> w421
          frame False {
            w448 = FALSE ("y")
          }
          frame True {
            w450 = TRUE ("3. Keep Null Flux Running \n       Until Next Step?")
            # "A Toggle fixed the problem!"
            n155 = case shown="True" w450 {
              tunnel: [0.0 ("output") w455] -> w451
              tunnel: w452 -> [_ w455]
              frame False {
                # "Reset AO at the end"
              }
              frame True {
                # "Keep Flux the same"
              }
            }
          }
        }
        n156 = call-poly <vilib>:"DAQmx Write.vi"("task/channels in"=w445, "data"=w419, "error in"=w444) -> ("task out"=w443:refnum<k21>, "error out"=w432:errorcluster)  [unwired: 10 in, 1 out]
        n157 = Unbundle By Name(w432) -> ("status"=w447:bool)  [unwired: 2 out]
        n158 = Not Or(1:w429, 2:w447) -> (0:w422:bool)
        n159 = node-c288() -> ()  [unwired: 1 in, 1 out]
      }
      n160 = Not(x=w396) -> (.not. x?=w394:bool)
      n161 = node-c288(w415) -> ()  [unwired: 1 out]
      n162 = shared-variable "NI-GenericDesktopPC-3A84958E\\Kopco PS Project Target Variables Library.lvlib\\Null Flux Running Middle"(w395) -> ()  [unwired: 1 in, 1 out]
      n163 = shared-variable "NI-GenericDesktopPC-3A84958E\\Kopco PS Project Target Variables Library.lvlib\\Zero Flux Observed GS"(w397) -> ()  [unwired: 1 in, 1 out]
      n164 = shared-variable "NI-GenericDesktopPC-3A84958E\\Kopco PS Project Target Variables Library.lvlib\\Null Flux Selected"(w394) -> ()  [unwired: 1 in, 1 out]
      n165 = shared-variable "NI-GenericDesktopPC-3A84958E\\Kopco PS Project Target Variables Library.lvlib\\Flux RT Control"(w396) -> ()  [unwired: 1 in, 1 out]
    }
    frame #12 {
      # "Zeroing the PS Output at the end with a STOP botton.\nReplacing it with a Toggle seemed to do the trick.\n \nSwitch the toggle \"mechanical action\" to \n\"Latch when Released\" so that it will reset to FALSE \nat the end every time."
      n166 = call <vilib>:"DAQmx Stop Task.vi"("task/channels in"=w481, "error in"=w479) -> ("task out"=w486:refnum<k21>, "error out"=w485:errorcluster)  [unwired: 12 in]
      n167 = call <vilib>:"DAQmx Clear Task.vi"("task in"=w486, "error in"=w485) -> ("error out"=w482:errorcluster)  [unwired: 13 in]
      n168 = call <vilib>:"DAQmx Stop Task.vi"("task/channels in"=w480, "error in"=w482) -> ("task out"=w484:refnum<k21>, "error out"=w483:errorcluster)  [unwired: 12 in]
      n169 = call <vilib>:"DAQmx Clear Task.vi"("task in"=w484, "error in"=w483) -> ()  [unwired: 13 in, 1 out]
    }
    frame #13 {
      (unwired) "OK!"
      (unwired) "1. REMOVE the needle from the sample (if needed).\n2. PREPARE for the next experiment.\n3. Click OK in this dialog box!\n4. ENTER the required variables here: (Flux Setpoint & Number of Cycles, & Length of Pre-and Post-Periods of Null Flux). Click \"Proceed with these Parameters.\"\n5. OPEN Data Logger (if you have not done so), ENTER file name, and RUN program. \n6. ADJUST the number of frames in the Fast Timelapse Macro (if a macro is used). Otherwise, skip this step. \n7. RUN the macro (if a macro is used). Otherwise, click \"TRGR\" button in Nikon Elements to initiate Fast Timelapse Image Capture, Data Acquisition, and PID-Controlled Sequence.\n"  # 1. REMOVE the needle from the sample (if needed). 2. PREPARE for the next experiment. 3. Click OK in this dialog box! 4. ENTER the required variables here: (Flux Setpoint & Number of Cycles, & Length of Pre-and Post-Periods of Null Flux). Click "Proceed with these Parameters." 5. OPEN Data Logger (if you have not done so), ENTER file name, and RUN program.  6. ADJUST the number of frames in the Fast Timelapse Macro (if a macro is used). Otherwise, skip this step.  7. RUN the macro (if a macro is used). Otherwise, click "TRGR" button in Nikon Elements to initiate Fast Timelapse Image Capture, Data Acquisition, and PID-Controlled Sequence.
      # "AO values of current"
      n170 = shared-variable "NI-GenericDesktopPC-3A84958E\\Kopco PS Project Target Variables Library.lvlib\\Flux Setpoint ON Gs Absolute"() -> (w489:dbl)  [unwired: 1 in, 1 out]
      "ON Absolute\nFlux Setpoint (Gs)" <- w489
      n171 = shared-variable "NI-GenericDesktopPC-3A84958E\\Kopco PS Project Target Variables Library.lvlib\\Zero Flux Observed Gs Corrected"() -> (w494:dbl)  [unwired: 1 in, 1 out]
      n172 = shared-variable "NI-GenericDesktopPC-3A84958E\\Kopco PS Project Target Variables Library.lvlib\\Null Flux Pre Period"() -> (w499:dbl)  [unwired: 1 in, 1 out]
      n173 = shared-variable "NI-GenericDesktopPC-3A84958E\\Kopco PS Project Target Variables Library.lvlib\\Period OFF 1st Per Cycle"() -> (w497:dbl)  [unwired: 1 in, 1 out]
      n174 = shared-variable "NI-GenericDesktopPC-3A84958E\\Kopco PS Project Target Variables Library.lvlib\\Period OFF 2nd Per Cycle"() -> (w498:dbl)  [unwired: 1 in, 1 out]
      n175 = shared-variable "NI-GenericDesktopPC-3A84958E\\Kopco PS Project Target Variables Library.lvlib\\Null Flux Post Period"() -> (w495:dbl)  [unwired: 1 in, 1 out]
      n176 = shared-variable "NI-GenericDesktopPC-3A84958E\\Kopco PS Project Target Variables Library.lvlib\\Period ON Per Cycle"() -> (w496:dbl)  [unwired: 1 in, 1 out]
      n177 = shared-variable "NI-GenericDesktopPC-3A84958E\\Kopco PS Project Target Variables Library.lvlib\\Cycles"() -> (w487:i16)  [unwired: 1 in, 1 out]
      n178 = Sign(1:w494) -> (0:w491:dbl)
      n179 = Negate(x=w491) -> (-x=w490:dbl)
      n180 = Multiply(x=w489, y=w490) -> (x*y=w493:dbl)
      n181 = property on="Number of Cycles" class="DigNum (strict)"("Value"=w487) -> ()  [unwired: 2 in, 2 out]
      n182 = property on="Pre-Wave Null Flux Interval (s)" class="DigNum (strict)"("Value"=w499) -> ()  [unwired: 2 in, 2 out]
      n183 = Add(x=w493, y=w494) -> (x+y=w492:dbl)
      n184 = property on="Post-Wave Null Flux Interval (s)" class="DigNum (strict)"("Value"=w495) -> ()  [unwired: 2 in, 2 out]
      n185 = property on="1st OFF Length (s)" class="DigNum (strict)"("Value"=w497) -> ()  [unwired: 2 in, 2 out]
      n186 = property on="OFF (s)" class="DigNum (strict)"("Value"=w498) -> ()  [unwired: 2 in, 2 out]
      n187 = property on="ON" class="DigNum (strict)"("Value"=w496) -> ()  [unwired: 2 in, 2 out]
      n188 = Multiply(x=w490, y=w492) -> (x*y=w488:dbl)
      n189 = shared-variable "NI-GenericDesktopPC-3A84958E\\Kopco PS Project Target Variables Library.lvlib\\Flux Setpoint ON Gs Relative"(w488) -> ()  [unwired: 1 in, 1 out]
      n190 = property on="Flux ON relative setpoint (Gs)" class="DigNum (strict)"("Value"=w488) -> ()  [unwired: 2 in, 2 out]
    }
    frame #14 {
      # "AO values of current"
      # "Bound to \"PID Parameters Selected\"\nshared global variable"
      # "Step 3 Specifying Waveform Parameters"
      # "Step 3 Specifying Waveform Parameters"
      n191 = while {
        tunnel: ["Proceed with Parameters"] -> w512
        tunnel: ["Flux ON relative setpoint (Gs)"] -> _
        tunnel: [w514] -> w511
        tunnel: ["Number of Cycles"] -> w510
        tunnel: ["Pre-Wave Null Flux Interval (s)"] -> w509
        tunnel: ["Post-Wave Null Flux Interval (s)"] -> w508
        tunnel: ["OFF (s)"] -> w504
        tunnel: ["ON"] -> w503
        stop <- "Proceed with Parameters" stop-if-true
        # "Updated code on \nto vary ON/OFF cycle"
        # "You can use a #negative #sign to go to the opposite end\nto extend the linear range if neeed."
        # "Changed Cycles type from double\nto integer-16bit on 1/8/2018"
        # "Global variables were moved inside this while loop to resolve\nthe problem of updating them. For whatever reason, LabVIEW\nseems to only pass to the variable the previous values but \nnot the updated ones for variable (but passes the updated version for \nan indicator). Verified on 1/8/2018 by #WIM"
        n192 = shared-variable "NI-GenericDesktopPC-3A84958E\\Kopco PS Project Target Variables Library.lvlib\\Digital Trigger"(FALSE ("Digital Trigger")) -> ()  [unwired: 1 in, 1 out]
        n193 = shared-variable "NI-GenericDesktopPC-3A84958E\\Kopco PS Project Target Variables Library.lvlib\\Cycles"("Number of Cycles") -> ()  [unwired: 1 in, 1 out]
        n194 = Add "Total Period Time (s)"(x="OFF (s)", y="ON") -> (x+y=w514:dbl)
        n195 = shared-variable "NI-GenericDesktopPC-3A84958E\\Kopco PS Project Target Variables Library.lvlib\\Flux Setpoint ON Gs Relative"("Flux ON relative setpoint (Gs)") -> ()  [unwired: 1 in, 1 out]
        n196 = shared-variable "NI-GenericDesktopPC-3A84958E\\Kopco PS Project Target Variables Library.lvlib\\Null Flux Post Period"("Post-Wave Null Flux Interval (s)") -> ()  [unwired: 1 in, 1 out]
        n197 = shared-variable "NI-GenericDesktopPC-3A84958E\\Kopco PS Project Target Variables Library.lvlib\\Null Flux Pre Period"("Pre-Wave Null Flux Interval (s)") -> ()  [unwired: 1 in, 1 out]
        n198 = shared-variable "NI-GenericDesktopPC-3A84958E\\Kopco PS Project Target Variables Library.lvlib\\Period Per Cycle"(w514) -> ()  [unwired: 1 in, 1 out]
      }
      n199 = shared-variable "NI-GenericDesktopPC-3A84958E\\Kopco PS Project Target Variables Library.lvlib\\Control Parameters Selected"(w512) -> ()  [unwired: 1 in, 1 out]
    }
    frame #15 {
      (unwired) 1.0 ("Double")
      w565 = 0 ("index")
      w592 = u32 1000  # ms/sec
      w599 = bool[] []  # Initial Empty Array
      w634 = dbl[] []  # Initial Zero Array
      w616 = 0.031  # Time Length (s)
      w665 = FALSE
      w647 = bool[] []  # Initial Empty Array
      w676 = dbl[] []  # Initial Zero Array
      # "Post Wave might need to be\nfixed with Ramp"
      # "No need for this"
      # "Number of Cycles"
      # "ON per Cycle (s)"
      # "OFF per Cycle (s)"
      # "Corrected Null Flux/OFF Observed (Gs):\n2nd Cycle OFF & Later & Postwave Corrected"
      # "1/4 wave to get the main points of the\n mini DeGauss waveform 3/12/2018"
      # "AO values of current"
      # "Into the Data Logger"
      # "Null Flux Observed:\n2nd Cycle OFF & Later & Postwave Corrected(V)"
      # "Null Flux Observed:\nPrewave & 1st Cycle OFF Uncorrected (V)\nNO CHANGE!"
      # "Initial Null Flux Observed (Gs)"
      # "5. Based on a sigmoidal curve fit 2019-08-08\nThe Equation is Y = Vmax * X^h /(K_prime + X^h), where Vmax = 13.91, h = 1.9431, and Kprime = 747"
      # "# of samples of Mini DeGauss"
      # "Three choices for mini DeGauss\nwaveform? \n0.030 ms @ 500 Hz   (No AI leakage at \nhigher fluxes ~ 200 Gs. Moreoever, flux\nvariation is higher = more atoms are recruited)\n0.030 ms @ 1000 Hz\n0.015 ms @ 1000 Hz"
      # "Added 3/12/2018"
      # "Amplitude will need to be modified later"
      # "OFF = 2 * 1/2 Cycle - samples of ON Mini DeGauss"
      # "30,000 @ 500 Hz\n\n1000 Hz for PID \nsampling rate of 1 ms\ncreate aliasing/roundoff error\n\nSampling at higher rate, and then\nchoose your points of interest"
      # "OFF = - samples of ON Mini DeGauss"
      # "Period per Cycle (s)"
      # "Flux Setpoint/On (V)"
      # "Flux Relative ON Setpoint (Gs)"
      # "Step 3 Building Waveforms for PID control and for mini-DeGauss Cycles"
      # "Step 3 Creating Waveforms"
      # "1/4/2018. It checks the maximum of either the observed zero or the \nsuperimposed ON setpoints for my OFF/ON square wave"
      # "ON/OFF PID Parameters. In order for this to work, the OFF flux needs to be near the linear range."
      # "Note: Max point is included in that given PID Gain schedule. it is the cut-off point"
      # "I was able to build a PID gain schedule by matching the types.\nThis way I will be able to customize the values based on sensor sensitivities\nand so forth 1/2/2017."
      # "Corrected on 1/4/2018"
      # "N cycles of High/Low\nCreate A Control Array in terms \nof flux sensor voltage"
      n200 = shared-variable "NI-GenericDesktopPC-3A84958E\\Kopco PS Project Target Variables Library.lvlib\\Sampling Rate"() -> (w527:dbl)  [unwired: 1 in, 1 out]
      n201 = To Quad Integer(1:w527) -> (0:w526:i64)
      n202 = shared-variable "NI-GenericDesktopPC-3A84958E\\Kopco PS Project Target Variables Library.lvlib\\Zero Flux Observed Gs Corrected"() -> (w598:dbl)  [unwired: 1 in, 1 out]
      "Corrective \nNull Flux (Gs)" <- w598
      n203 = shared-variable "NI-GenericDesktopPC-3A84958E\\Kopco PS Project Target Variables Library.lvlib\\Sensor Sensitivity Core"() -> (w543:dbl)  [unwired: 1 in, 1 out]
      n204 = shared-variable "NI-GenericDesktopPC-3A84958E\\Kopco PS Project Target Variables Library.lvlib\\Flux Setpoint ON Gs Relative"() -> (w522:dbl)  [unwired: 1 in, 1 out]
      n205 = Divide "ms to sec"(x="Ramp Total Interval (ms)", y=w592) -> (x/y=w591:dbl)
      n206 = shared-variable "NI-GenericDesktopPC-3A84958E\\Kopco PS Project Target Variables Library.lvlib\\Zero Flux Observed GS"() -> (w588:dbl)  [unwired: 1 in, 1 out]
      n207 = shared-variable "NI-GenericDesktopPC-3A84958E\\Kopco PS Project Target Variables Library.lvlib\\Ramp Total Interval (ms)"("Ramp Total Interval (ms)") -> ()  [unwired: 1 in, 1 out]
      n208 = shared-variable "NI-GenericDesktopPC-3A84958E\\Kopco PS Project Target Variables Library.lvlib\\Ramp Steps"("# Ramp Steps") -> ()  [unwired: 1 in, 1 out]
      n209 = shared-variable "NI-GenericDesktopPC-3A84958E\\Kopco PS Project Target Variables Library.lvlib\\Flux Setpoint ON Gs Relative"() -> (w575:dbl)  [unwired: 1 in, 1 out]
      n210 = shared-variable "NI-GenericDesktopPC-3A84958E\\Kopco PS Project Target Variables Library.lvlib\\Sensor Sensitivity Core"() -> (w544:dbl)  [unwired: 1 in, 1 out]
      n211 = Multiply "# Total ramp\nSamples"(x=w591, y=w526) -> (x*y=w595:dbl)
      n212 = Multiply "# of Samples"(x=w616, y=w526) -> (x*y=w606:dbl)
      n213 = Divide(x=750.0, y=900.0) -> (x/y=w605:dbl)
      n214 = To Unsigned Long Integer(number=w606) -> (unsigned 32bit integer=w600:u32)
      n215 = To Unsigned Long Integer "# total ramp\nsamples (int)"(number=w595) -> (unsigned 32bit integer=w578:u32)
      n216 = Multiply(x=w606, y=w605) -> (x*y=w602:dbl)
      n217 = Subtract "Uncorrected to Corrected\n OFF Shift (Gs)"(x=w598, y=w588) -> (x-y=w576:dbl)
      n218 = for "One Mini DeGauss Cycle" {
        N: w600 -> [_]
        tunnel: w526 -> [w723]
        tunnel: [w739] -> w626 mode=indexing
        tunnel: w616 -> [w724]
        tunnel: [w723] -> w615
        tunnel: [w722] -> w614
        i -> [w738]
        w727 = 7.5  # amplitude
        w729 = 1.0  # Starting Amplitude
        w743 = 90.0  # Phase, Deg
        w722 = u64 480  # Frequency, Hz
        # "It seems 0.3 * Time will give \na decay around 20 ms."
        # "samples/sec"
        n219 = To Double Precision Float(number=w738) -> (double precision float=w740:dbl)
        n220 = Multiply(x=w724, y=0.3) -> (x*y=w725:dbl)
        n221 = Divide(x=w740, y=w723) -> (x/y=w734:dbl)
        n222 = Square(x=w734) -> (x^2=w736:dbl)
        n223 = Square(x=w725) -> (x^2=w732:dbl)
        n224 = Natural Logarithm(1:2.0 ("x")) -> (0:w730:dbl)
        n225 = Divide(x=w730, y=w732) -> (x/y=w731:dbl)
        n226 = Negate(x=w736) -> (-x=w735:dbl)
        n227 = Multiply(x=w735, y=w731) -> (x*y=w741:dbl)
        n228 = call <vilib>:"Sine Wave PtByPt.vi"("time"=w734, "phase"=w743, "frequency"=w722, "amplitude"=w727) -> ("sine wave"=w728:dbl)
        n229 = Exponential "Exp(-t^2*k)"(1:w741) -> (0:w742:dbl)
        n230 = Multiply(x=w742, y=w729) -> (x*y=w737:dbl)
        n231 = Multiply(x=w728, y=w737) -> (x*y=w739:dbl)
      }
      n232 = Increment "Make one extra to trim"(x="# Ramp Steps") -> (x+1=w587:u32)
      n233 = To Unsigned Long Integer(number=w602) -> (unsigned 32bit integer=w601:u32)
      n234 = Multiply "OFF (Uncorrected) \nGs to V"(x=w598, y=w543) -> (x*y=w589:dbl)
      n235 = Divide "Jump/Step \nON to Uncorrected \nOFF (Gs)"(x=w575, y="# Ramp Steps") -> (x/y=w577:dbl)
      n236 = Multiply "ON\nGs to V"(x=w522, y=w543) -> (x*y=w655:dbl)
      n237 = Quotient & Remainder "Samples # \nper step"(x=w578, y="# Ramp Steps") -> (floor(x/y)=w572:u32)  [unwired: 1 out]
      n238 = Add "ON + Offset from \nObserved Zero (V)"(x=w589, y=w655) -> (x+y=w675:dbl)
      n239 = Subtract "Jump ON to \nCorrected OFF (Gs)"(x=w575, y=w576) -> (x-y=w573:dbl)
      n240 = Divide "Jump/Step\nON to Corrected\nOFF (Gs)"(x=w573, y="# Ramp Steps") -> (x/y=w574:dbl)
      n241 = for "Create Ramp Steps" {
        N: w587 -> [_]
        shift-right: [w712] -> w566
        shift-left: dbl[] [] -> [w714]
        tunnel: w598 -> [w698]
        tunnel: w588 -> [w697]
        tunnel: w544 -> [w704]
        shift-right: [w709] -> w571
        shift-left: dbl[] [] -> [w708]
        tunnel: [w703] -> w564
        tunnel: w572 -> [w703]
        tunnel: w577 -> [w702]
        tunnel: w574 -> [w701]
        i -> [w705]
        n242 = To Double Precision Float(number=w705) -> (double precision float=w707:dbl)
        n243 = Multiply "Going thru\nSteps"(x=w707, y=w701) -> (x*y=w706:dbl)
        n244 = Multiply "Going thru\nSteps"(x=w707, y=w702) -> (x*y=w711:dbl)
        n245 = Add "UnCorrected Null flux Offset"(x=w711, y=w697) -> (x+y=w700:dbl)
        n246 = Add "Corrected Null Flux\nOffset"(x=w706, y=w698) -> (x+y=w699:dbl)
        n247 = Multiply "V to Gs"(x=w700, y=w704) -> (x*y=w696:dbl)
        n248 = Multiply "V to Gs"(x=w704, y=w699) -> (x*y=w695:dbl)
        n249 = Initialize Array "Current \nStep"(w696, w703) -> (w713:dbl[])
        n250 = Initialize Array "Current \nStep"(w695, w703) -> (w710:dbl[])
        n251 = Build Array (concatenate) "Uncorrected OFF\n to ON Ramp (V)"(w714, w713) -> (w712:dbl[])
        n252 = Build Array (concatenate) "Corrected OFF \nto ON Ramp (V)"(w708, w710) -> (w709:dbl[])
      }
      n253 = Multiply "# samples: OFF"(x=w526, y=w528) -> (x*y=w582:dbl)
      n254 = Multiply "# samples ON"(x=w526, y=w597) -> (x*y=w586:dbl)
      n255 = Multiply "Pre-wave Zero Inteval Samples"(x=w660, y=w526) -> (x*y=w673:dbl)
      n256 = Multiply "Post-wave Zero Interval Samples"(x=w659, y=w526) -> (x*y=w534:dbl)
      n257 = Reciprocal "period (s)"(x=w614) -> (1/x=w611:dbl)
      n258 = To Quad Integer(1:w534) -> (0:w532:i64)
      n259 = To Quad Integer(1:w673) -> (0:w533:i64)
      n260 = Multiply "Samples/wave"(x=w615, y=w611) -> (x*y=w612:dbl)
      n261 = Quotient & Remainder "1/4 wave"(x=w612, y=u8 4) -> (floor(x/y)=w608:dbl)  [unwired: 1 out]
      n262 = To Unsigned Long Integer(number=w608) -> (unsigned 32bit integer=w607:u32)
      n263 = Reverse 1D Array "ON to Uncorrected OFF"(array=w566) -> (reversed array=w570:dbl[])
      n264 = Reverse 1D Array "ON to corrected OFF"(array=w571) -> (reversed array=w569:dbl[])
      n265 = Delete From Array "Remove ON"(array=w570, length=w564, index=w565) -> (array with subset deleted=w555:dbl[])  [unwired: 1 out]
      n266 = Delete From Array "Remove ON"(array=w569, length=w564, index=w565) -> (array with subset deleted=w537:dbl[])  [unwired: 1 out]
      n267 = Delete From Array "Remove First \ncorrected OFF step\nto ON"(array=w571, length=w564, index=w565) -> (array with subset deleted=w556:dbl[])  [unwired: 1 out]
      n268 = Delete From Array "Remove First \nUncorrected OFF step\nto ON"(array=w566, length=w564, index=w565) -> (array with subset deleted=w563:dbl[])  [unwired: 1 out]
      n269 = Array Size(array=w563) -> (size(s)=w580:i32)
      n270 = Array Size(array=w537) -> (size(s)=w559:i32)
      n271 = Array Size(array=w556) -> (size(s)=w562:i32)
      n272 = Array Size(array=w555) -> (size(s)=w557:i32)
      n273 = Decrement "last item"(x=w580) -> (x-1=w579:i32)
      n274 = Array Size "Size ON Ramp"(array=w537) -> (size(s)=w558:i32)
      n275 = Array Size "Size OFF Ramp"(array=w556) -> (size(s)=w539:i32)
      n276 = Decrement "last item"(x=w562) -> (x-1=w561:i32)
      n277 = Decrement "last item"(x=w559) -> (x-1=w551:i32)
      n278 = Decrement "last item"(x=w557) -> (x-1=w552:i32)
      n279 = Index Array "ON"(array=w563, index=w579) -> (element=w585:dbl)
      n280 = Index Array "ON"(array=w556, index=w561) -> (element=w584:dbl)
      n281 = Index Array "Corrected OFF"(array=w537, index=w551) -> (element=w535:dbl)
      n282 = Index Array "Uncorrected OFF"(array=w555, index=w552) -> (element=w583:dbl)
      n283 = Subtract "OFF Ramp Samples #"(x=w582, y=w539) -> (x-y=w568:dbl)
      n284 = Subtract "ON Ramp Samples #"(x=w586, y=w558) -> (x-y=w567:dbl)
      n285 = Subtract "Post-Wave OFF Sample #"(x=w532, y=w539) -> (x-y=w536:i64)
      n286 = Initialize Array "Extend PostOFF"(w535, w536) -> (w538:dbl[])
      n287 = Initialize Array "Extend OFF"(w535, w568) -> (w553:dbl[])
      n288 = Initialize Array "Extend ON"(w585, w567) -> (w581:dbl[])
      n289 = Initialize Array "Extend OFF"(w583, w568) -> (w554:dbl[])
      n290 = Initialize Array "Extend ON"(w584, w567) -> (w560:dbl[])
      n291 = Build Array (concatenate) "ON to Corrected OFF (V) First Step Removed\nPost-Wave"(w537, w538) -> (w529:dbl[])
      n292 = Build Array (concatenate) "UnCorrected OFF\n to ON (V)\nFirst Step Removed"(w563, w581) -> (w547:dbl[])
      n293 = Build Array (concatenate) "ON to UnCorrected OFF (V)\nFirst Step Removed"(w555, w554) -> ()  [unwired: 1 out]
      n294 = Build Array (concatenate) "Corrected OFF\n to ON (V)\nFirst Step Removed"(w556, w560) -> (w546:dbl[])
      n295 = Build Array (concatenate) "ON to Corrected OFF (V)\nFirst Step Removed"(w537, w553) -> (w530:dbl[])
      n296 = case "Force Step Ramps" shown="True" "7.            Step(s) Force Ramp in              (ms)?" {
        tunnel: [w681 w691] -> w550
        tunnel: w675 -> [w684 _]
        tunnel: [w682 w690] -> w548
        tunnel: [w680 w694] -> w549
        tunnel: w589 -> [w686 w689]
        tunnel: w589 -> [w687 _]
        tunnel: w586 -> [w683 _]
        tunnel: w582 -> [w685 w693]
        tunnel: w546 -> [_ w690]
        tunnel: w547 -> [_ w692]
        tunnel: w530 -> [_ w691]
        tunnel: [w682 w692] -> w545
        tunnel: w529 -> [_ w688]
        tunnel: w589 -> [w679 _]
        tunnel: w532 -> [w678 _]
        tunnel: [w677 w688] -> w531
        frame False {
          # "OFF: 1st cycle"
          # "ON: all cycles"
          # "OFF: 2nd cycle\n& Later"
          # "NO RAMP"
          # "OFF (corrected) to ON (V)"
          # "OFF (Uncorrected) to ON (V)"
          # "ON + Offset from \nObserved Zero (V)"
          n297 = Initialize Array "Post Wave"(w679, w678) -> (w677:dbl[])
          n298 = Initialize Array "1. corrected OFF"(w687, w685) -> (w681:dbl[])
          n299 = Initialize Array "1.  Uncorrected OFF"(w686, w685) -> (w680:dbl[])
          n300 = Initialize Array "2. ON"(w684, w683) -> (w682:dbl[])
        }
        frame True {
          # "OFF: Post-wave Zero"
          # "OFF: 1st cycle"
          # "OFF: 2nd Cycle & Later"
          # "ON: 2nd Cycle & Later"
          # "ON: 1st cycle"
          # "2. On to corrected OFF (V)"
          # "1. uncorrected OFF to ON (V)"
          # "WITH Steps RAMP"
          # "1. corrected OFF to ON (V)"
          n301 = Initialize Array "1. Uncorrected OFF"(w689, w693) -> (w694:dbl[])
        }
      }
      n302 = Subtract(x=w582, y=w600) -> (x-y=w635:dbl)
      n303 = Initialize Array "1. Off"(FALSE, w582) -> (w670:bool[])
      n304 = Initialize Array "2. On"(TRUE, w586) -> (w669:bool[])
      n305 = Initialize Array "2. Off"(0.0 ("dimension size"), w635) -> (w637:dbl[])
      n306 = Initialize Array "2. Off"(FALSE, w635) -> (w653:bool[])
      n307 = Initialize Array "2. Off"(FALSE, w582) -> (w623:bool[])
      n308 = Initialize Array "1. On"(TRUE, w586) -> (w654:bool[])
      n309 = Initialize Array "2. Off"(0.0 ("dimension size"), w582) -> (w621:dbl[])
      n310 = Build Array (concatenate) "1st Cycle\nOne cycle: OFF/ON"(w549, w545) -> (w525:dbl[])
      n311 = Build Array (concatenate) "2nd Cycle & later\nOne Cycle: OFF/ON"(w550, w548) -> (w524:dbl[])
      n312 = Build Array (concatenate) "Magnetic Flux Control\nWaveform OFF/ON? Array"(w670, w669) -> (w666:bool[])
      n313 = Build Array (concatenate) "Mini DeGauss\nAO Waveform Array"(w626, w637) -> (w625:dbl[])
      n314 = To Quad Integer(1:w533) -> (0:w620:i64)
      n315 = Build Array (concatenate) "Mini DeGauss\nWaveform OFF/ON? Array"(w654, w653) -> (w650:bool[])
      n316 = Less?(x=w532, y=w600) -> (x < y?=w638:bool)
      n317 = Less?(x=w620, y=w600) -> (x < y?=w619:bool)
      n318 = case "Pre-Mini DeGauss?" shown="True" w619 {
        tunnel: [w715 w721] -> w618
        tunnel: w620 -> [w716 _]
        tunnel: [w717 w720] -> w617
        frame False {
          # "Modified mini DeGauss to not include it in the \npre-wave on 3/9/2018"
          n319 = Initialize Array "Off"(0.0 ("dimension size"), w716) -> (w717:dbl[])
          n320 = Initialize Array "Off"(FALSE, w716) -> (w715:bool[])
        }
        frame True {
          w720 = dbl[] []  # Initial Zero Array
          w721 = bool[] []  # Initial Empty Array
          # "Pre-wave is smaller than the \nmini-DeGauss cycle"
        }
      }
      n321 = case "Post-Mini DeGauss" shown="False" w638 {
        tunnel: [w751 w757] -> w646
        tunnel: w532 -> [w750 _]
        tunnel: w600 -> [w749 _]
        tunnel: w626 -> [w746 _]
        tunnel: [w744 w756] -> w627
        frame False {
          n322 = Subtract(x=w750, y=w749) -> (x-y=w745:i64)
          n323 = Initialize Array "2. Off"(0.0 ("dimension size"), w745) -> (w748:dbl[])
          n324 = Initialize Array "1. On"(TRUE, w749) -> (w755:bool[])
          n325 = Initialize Array "2. Off"(FALSE, w745) -> (w754:bool[])
          n326 = Build Array (concatenate) "Mini DeGauss\nWaveform OFF/ON? Array"(w746, w748) -> (w744:dbl[])
          n327 = Build Array (concatenate) "Post-Mini DeGauss\nWave"(w755, w754) -> (w751:bool[])
        }
        frame True {
          w756 = dbl[] []  # Initial Zero Array
          w757 = bool[] []  # Initial Empty Array
          # "Post-wave is smaller than the \nmini-DeGauss cycle"
        }
      }
      n328 = for "Building N Cycles of OFF/ON Wavefform" {
        N: w661 -> [_]
        tunnel: w524 -> [w764]
        shift-right: [w762] -> w542
        shift-left: w676 -> [w765]
        shift-right: [w777] -> w664
        shift-left: w647 -> [w779]
        tunnel: w666 -> [w778]
        shift-right: [w776] -> w639
        shift-left: w599 -> [w775]
        tunnel: w650 -> [w774]
        shift-right: [w773] -> w633
        shift-left: w634 -> [w771]
        tunnel: w625 -> [w772]
        tunnel: w623 -> [w767]
        tunnel: w621 -> [w766]
        tunnel: w525 -> [w763]
        i -> [w770]
        n329 = Equal? "First Cycle?"(x=0, y=w770) -> (x = y?=w768:bool)
        n330 = case "First Cycle?" shown="False" w768 {
          tunnel: [w788 w793] -> w776
          tunnel: w775 -> [w787 _]
          tunnel: w774 -> [w786 _]
          tunnel: [w785 w792] -> w773
          tunnel: w772 -> [w784 _]
          tunnel: w771 -> [w783 _]
          tunnel: w767 -> [_ w793]
          tunnel: w766 -> [_ w792]
          tunnel: w765 -> [w782 w791]
          tunnel: [w781 w789] -> w762
          tunnel: w764 -> [w780 _]
          tunnel: w763 -> [_ w790]
          frame False {
            n331 = Build Array (concatenate) "Build Array"(w787, w786) -> (w788:bool[])
            n332 = Build Array (concatenate) "Corrected"(w782, w780) -> (w781:dbl[])
            n333 = Build Array (concatenate) "Build Array"(w783, w784) -> (w785:dbl[])
          }
          frame True {
            n334 = Build Array (concatenate) "Uncorrected"(w791, w790) -> (w789:dbl[])
          }
        }
        n335 = Build Array (concatenate) "Build Array"(w779, w778) -> (w777:bool[])
      }
      n336 = Initialize Array "Pre-Wave"(w589, w620) -> (w596:dbl[])
      n337 = Initialize Array "Pre-Wave Zero"(w665, w620) -> (w649:bool[])
      n338 = Initialize Array "Post Wave Zero"(w665, w532) -> (w648:bool[])
      n339 = Build Array (concatenate) "Mini-DeGauss  \n Waveform OFF/ON? Array"(w618, w639, w646) -> (w643:bool[])
      n340 = Build Array (concatenate) "Mini-DeGauss  \n Waveform AO Sequence"(w617, w633, w627) -> (w631:dbl[])
      n341 = Build Array (concatenate) "Magnetic Flux \nControl Waveform OFF/ON? Array"(w649, w664, w648) -> (w663:bool[])
      n342 = Array Size(array=w631) -> (size(s)=w632:i32)
      n343 = Multiply "Samples/cycle"(x=w526, y=w662) -> (x*y=w674:dbl)
      n344 = Array Size(array=w643) -> (size(s)=w644:i32)
      n345 = Add "Pre & Post Samples"(x=w620, y=w532) -> (x+y=w672:i64)
      n346 = Build Array (concatenate) "Magnetic Flux \nControl Array"(w596, w542, w531) -> (w523:dbl[])
      n347 = Initialize Array "1. Off"(0.0, w632) -> (w629:dbl[])
      n348 = Initialize Array "1. Off"(FALSE, w644) -> (w641:bool[])
      n349 = Multiply "Total Number of OFF/ON Samples"(x=w674, y=w661) -> (x*y=w610:dbl)
      n350 = To Unsigned Long Integer(number=w610) -> (unsigned 32bit integer=w609:u32)
      n351 = case "Mini DeGauss? YES/NO?" shown="False" FALSE ("6. Mini DeGauss cycles in OFF segments?") {
        tunnel: w643 -> [_ w761]
        tunnel: [w759 w761] -> w642
        tunnel: w641 -> [w759 _]
        tunnel: w631 -> [_ w760]
        tunnel: w629 -> [w758 _]
        tunnel: [w758 w760] -> w628
        frame False {
          # "NO mini\nDeGauss \ncycles"
        }
        frame True {
          # "Mini DeGauss\ncycles"
        }
      }
      n352 = Add "Total # of Samples"(x=w609, y=w672) -> (x+y=w671:i64)
    }
    frame #16 {
      # "1/4 wave to get the main points of the\n mini DeGauss waveform 3/12/2018"
      # "# of samples of Mini DeGauss"
      # "Flux ON/OFF Logical"
      # "Sampling Rate"
      # "Flux Control Sequence"
      # "Mini DeGauss AO Sequence, Normalized"
      # "Mini DeGauss Logical"
      # "AO values of current"
      # "1 for #1\n2 for #2"
      # "#WIM 1/16/2018\nPID Aggressiveness\n0 = Optimized\n1 = Minimum\n2 = Average\n3 = Maximum"
      # "Step 4 Specifying PID Parameters"
      # "Total Number of Samples"
      # "#WIM 1/10/2018\nPID Parameters List Selection:\n0 = Fixed Schedule\n1 = Interpolated Schedule"
      n353 = shared-variable "NI-GenericDesktopPC-3A84958E\\Kopco PS Project Target Variables Library.lvlib\\Needle Used"() -> (w823:i8)  [unwired: 1 in, 1 out]
      n354 = case "Needle Chosen: #1 or #2" shown="1, Default" w823 {
        tunnel: [w859 w865] -> w829
        tunnel: [w858 w864] -> w828
        tunnel: [w857 w860] -> w827
        tunnel: [w856 w863] -> w826
        tunnel: [w855 w861] -> w818
        tunnel: [w854 w862] -> w817
        frame 1, Default {
          w854 = T2 [{"PID gains"={"proportional gain (Kc)"=0.053, "integral time (Ti, min)"=3.5e-06, "derivative time (Td, min)"=0.0}, "max value"=0.0}, {"PID gains"={"proportional gain (Kc)"=0.053, "integral time (Ti, min)"=3.5e-06, "derivative time (Td, min)"=0.0}, "max value"=75.0}, {"PID gains"={"proportional gain (Kc)"=0.053, "integral time (Ti, min)"=3.5e-06, "derivative time (Td, min)"=0.0}, "max value"=100.0}, {"PID gains"={"proportional gain (Kc)"=0.055, "integral time (Ti, min)"=3.5e-06, "derivative time (Td, min)"=0.0}, "max value"=125.0}, {"PID gains"={"proportional gain (Kc)"=0.055, "integral time (Ti, min)"=3.5e-06, "derivative time (Td, min)"=0.0}, "max value"=150.0}, {"PID gains"={"proportional gain (Kc)"=0.055, "integral time (Ti, min)"=3.5e-06, "derivative time (Td, min)"=0.0}, "max value"=160.0}, {"PID gains"={"proportional gain (Kc)"=0.056, "integral time (Ti, min)"=3.5e-06, "derivative time (Td, min)"=0.0}, "max value"=165.0}, {"PID gains"={"proportional gain (Kc)"=0.056, "integral time (Ti, min)"=3.5e-06, "derivative time (Td, min)"=0.0}, "max value"=170.0}, {"PID gains"={"proportional gain (Kc)"=0.058, "integral time (Ti, min)"=3.5e-06, "derivative time (Td, min)"=0.0}, "max value"=175.0}, {"PID gains"={"proportional gain (Kc)"=0.058, "integral time (Ti, min)"=3.5e-06, "derivative time (Td, min)"=0.0}, "max value"=180.0}, {"PID gains"={"proportional gain (Kc)"=0.058, "integral time (Ti, min)"=3.5e-06, "derivative time (Td, min)"=0.0}, "max value"=185.0}, {"PID gains"={"proportional gain (Kc)"=0.058, "integral time (Ti, min)"=3.5e-06, "derivative time (Td, min)"=0.0}, "max value"=190.0}, {"PID gains"={"proportional gain (Kc)"=0.058, "integral time (Ti, min)"=3.5e-06, "derivative time (Td, min)"=0.0}, "max value"=210.0}]  # OFF PID gain schedule HyMu80#1 Needle OPTIMIZED
          w855 = T2 [{"PID gains"={"proportional gain (Kc)"=0.053, "integral time (Ti, min)"=3.5e-06, "derivative time (Td, min)"=0.0}, "max value"=0.0}, {"PID gains"={"proportional gain (Kc)"=0.053, "integral time (Ti, min)"=3.5e-06, "derivative time (Td, min)"=0.0}, "max value"=75.0}, {"PID gains"={"proportional gain (Kc)"=0.053, "integral time (Ti, min)"=3.5e-06, "derivative time (Td, min)"=0.0}, "max value"=100.0}, {"PID gains"={"proportional gain (Kc)"=0.055, "integral time (Ti, min)"=3.5e-06, "derivative time (Td, min)"=0.0}, "max value"=125.0}, {"PID gains"={"proportional gain (Kc)"=0.057, "integral time (Ti, min)"=3.5e-06, "derivative time (Td, min)"=0.0}, "max value"=150.0}, {"PID gains"={"proportional gain (Kc)"=0.058, "integral time (Ti, min)"=3.5e-06, "derivative time (Td, min)"=0.0}, "max value"=160.0}, {"PID gains"={"proportional gain (Kc)"=0.065, "integral time (Ti, min)"=3.5e-06, "derivative time (Td, min)"=0.0}, "max value"=165.0}, {"PID gains"={"proportional gain (Kc)"=0.111, "integral time (Ti, min)"=3.5e-06, "derivative time (Td, min)"=0.0}, "max value"=170.0}, {"PID gains"={"proportional gain (Kc)"=0.27, "integral time (Ti, min)"=3.5e-06, "derivative time (Td, min)"=0.0}, "max value"=175.0}, {"PID gains"={"proportional gain (Kc)"=0.32, "integral time (Ti, min)"=3.5e-06, "derivative time (Td, min)"=0.0}, "max value"=180.0}, {"PID gains"={"proportional gain (Kc)"=0.72, "integral time (Ti, min)"=3.5e-06, "derivative time (Td, min)"=0.0}, "max value"=185.0}, {"PID gains"={"proportional gain (Kc)"=0.8, "integral time (Ti, min)"=3.5e-06, "derivative time (Td, min)"=0.0}, "max value"=190.0}, {"PID gains"={"proportional gain (Kc)"=0.8, "integral time (Ti, min)"=3.5e-06, "derivative time (Td, min)"=0.0}, "max value"=210.0}]  # ON PID gain schedule HyMu80#1 Needle OPTIMIZED
          w856 = T2 [{"PID gains"={"proportional gain (Kc)"=0.08, "integral time (Ti, min)"=3.5e-06, "derivative time (Td, min)"=0.0}, "max value"=0.0}, {"PID gains"={"proportional gain (Kc)"=0.08, "integral time (Ti, min)"=3.5e-06, "derivative time (Td, min)"=0.0}, "max value"=145.0}, {"PID gains"={"proportional gain (Kc)"=0.075, "integral time (Ti, min)"=3.5e-06, "derivative time (Td, min)"=0.0}, "max value"=148.0}, {"PID gains"={"proportional gain (Kc)"=0.075, "integral time (Ti, min)"=3.5e-06, "derivative time (Td, min)"=0.0}, "max value"=150.0}, {"PID gains"={"proportional gain (Kc)"=0.075, "integral time (Ti, min)"=3.5e-06, "derivative time (Td, min)"=0.0}, "max value"=155.0}, {"PID gains"={"proportional gain (Kc)"=0.075, "integral time (Ti, min)"=3.5e-06, "derivative time (Td, min)"=0.0}, "max value"=160.0}, {"PID gains"={"proportional gain (Kc)"=0.078, "integral time (Ti, min)"=3.5e-06, "derivative time (Td, min)"=0.0}, "max value"=165.0}, {"PID gains"={"proportional gain (Kc)"=0.078, "integral time (Ti, min)"=3.5e-06, "derivative time (Td, min)"=0.0}, "max value"=170.0}, {"PID gains"={"proportional gain (Kc)"=0.081, "integral time (Ti, min)"=3.5e-06, "derivative time (Td, min)"=0.0}, "max value"=175.0}, {"PID gains"={"proportional gain (Kc)"=0.08, "integral time (Ti, min)"=3.5e-06, "derivative time (Td, min)"=0.0}, "max value"=180.0}, {"PID gains"={"proportional gain (Kc)"=0.085, "integral time (Ti, min)"=3.5e-06, "derivative time (Td, min)"=0.0}, "max value"=185.0}, {"PID gains"={"proportional gain (Kc)"=0.086, "integral time (Ti, min)"=3.5e-06, "derivative time (Td, min)"=0.0}, "max value"=190.0}, {"PID gains"={"proportional gain (Kc)"=0.086, "integral time (Ti, min)"=3.5e-06, "derivative time (Td, min)"=0.0}, "max value"=195.0}, {"PID gains"={"proportional gain (Kc)"=0.086, "integral time (Ti, min)"=3.5e-06, "derivative time (Td, min)"=0.0}, "max value"=220.0}]  # OFF PID gain schedule HyMu80#1 Needle MAX
          w857 = T2 [{"PID gains"={"proportional gain (Kc)"=0.08, "integral time (Ti, min)"=3.5e-06, "derivative time (Td, min)"=0.0}, "max value"=0.0}, {"PID gains"={"proportional gain (Kc)"=0.08, "integral time (Ti, min)"=3.5e-06, "derivative time (Td, min)"=0.0}, "max value"=145.0}, {"PID gains"={"proportional gain (Kc)"=0.075, "integral time (Ti, min)"=3.5e-06, "derivative time (Td, min)"=0.0}, "max value"=148.0}, {"PID gains"={"proportional gain (Kc)"=0.075, "integral time (Ti, min)"=3.5e-06, "derivative time (Td, min)"=0.0}, "max value"=150.0}, {"PID gains"={"proportional gain (Kc)"=0.075, "integral time (Ti, min)"=3.5e-06, "derivative time (Td, min)"=0.0}, "max value"=155.0}, {"PID gains"={"proportional gain (Kc)"=0.075, "integral time (Ti, min)"=3.5e-06, "derivative time (Td, min)"=0.0}, "max value"=160.0}, {"PID gains"={"proportional gain (Kc)"=0.078, "integral time (Ti, min)"=3.5e-06, "derivative time (Td, min)"=0.0}, "max value"=165.0}, {"PID gains"={"proportional gain (Kc)"=0.078, "integral time (Ti, min)"=3.5e-06, "derivative time (Td, min)"=0.0}, "max value"=170.0}, {"PID gains"={"proportional gain (Kc)"=0.081, "integral time (Ti, min)"=3.5e-06, "derivative time (Td, min)"=0.0}, "max value"=175.0}, {"PID gains"={"proportional gain (Kc)"=0.08, "integral time (Ti, min)"=3.5e-06, "derivative time (Td, min)"=0.0}, "max value"=180.0}, {"PID gains"={"proportional gain (Kc)"=0.085, "integral time (Ti, min)"=3.5e-06, "derivative time (Td, min)"=0.0}, "max value"=185.0}, {"PID gains"={"proportional gain (Kc)"=0.086, "integral time (Ti, min)"=3.5e-06, "derivative time (Td, min)"=0.0}, "max value"=190.0}, {"PID gains"={"proportional gain (Kc)"=0.086, "integral time (Ti, min)"=3.5e-06, "derivative time (Td, min)"=0.0}, "max value"=195.0}, {"PID gains"={"proportional gain (Kc)"=0.086, "integral time (Ti, min)"=3.5e-06, "derivative time (Td, min)"=0.0}, "max value"=220.0}]  # OFF PID gain schedule HyMu80#1 Needle MIN
          w858 = T2 [{"PID gains"={"proportional gain (Kc)"=0.08, "integral time (Ti, min)"=3.5e-06, "derivative time (Td, min)"=0.0}, "max value"=0.0}, {"PID gains"={"proportional gain (Kc)"=0.08, "integral time (Ti, min)"=3.5e-06, "derivative time (Td, min)"=0.0}, "max value"=145.0}, {"PID gains"={"proportional gain (Kc)"=0.083, "integral time (Ti, min)"=3.5e-06, "derivative time (Td, min)"=0.0}, "max value"=148.0}, {"PID gains"={"proportional gain (Kc)"=0.085, "integral time (Ti, min)"=3.5e-06, "derivative time (Td, min)"=0.0}, "max value"=150.0}, {"PID gains"={"proportional gain (Kc)"=0.0875, "integral time (Ti, min)"=3.5e-06, "derivative time (Td, min)"=0.0}, "max value"=155.0}, {"PID gains"={"proportional gain (Kc)"=0.123, "integral time (Ti, min)"=3.5e-06, "derivative time (Td, min)"=0.0}, "max value"=160.0}, {"PID gains"={"proportional gain (Kc)"=0.207, "integral time (Ti, min)"=3.5e-06, "derivative time (Td, min)"=0.0}, "max value"=165.0}, {"PID gains"={"proportional gain (Kc)"=0.315, "integral time (Ti, min)"=3.5e-06, "derivative time (Td, min)"=0.0}, "max value"=170.0}, {"PID gains"={"proportional gain (Kc)"=0.46, "integral time (Ti, min)"=3.5e-06, "derivative time (Td, min)"=0.0}, "max value"=175.0}, {"PID gains"={"proportional gain (Kc)"=0.65, "integral time (Ti, min)"=3.5e-06, "derivative time (Td, min)"=0.0}, "max value"=180.0}, {"PID gains"={"proportional gain (Kc)"=0.925, "integral time (Ti, min)"=3.5e-06, "derivative time (Td, min)"=0.0}, "max value"=185.0}, {"PID gains"={"proportional gain (Kc)"=1.04, "integral time (Ti, min)"=3.5e-06, "derivative time (Td, min)"=0.0}, "max value"=190.0}, {"PID gains"={"proportional gain (Kc)"=1.04, "integral time (Ti, min)"=3.5e-06, "derivative time (Td, min)"=0.0}, "max value"=195.0}, {"PID gains"={"proportional gain (Kc)"=1.04, "integral time (Ti, min)"=3.5e-06, "derivative time (Td, min)"=0.0}, "max value"=220.0}]  # ON PID gain schedule HyMu80#1 Needle MAX
          w859 = T2 [{"PID gains"={"proportional gain (Kc)"=0.075, "integral time (Ti, min)"=3.5e-06, "derivative time (Td, min)"=0.0}, "max value"=0.0}, {"PID gains"={"proportional gain (Kc)"=0.075, "integral time (Ti, min)"=3.5e-06, "derivative time (Td, min)"=0.0}, "max value"=145.0}, {"PID gains"={"proportional gain (Kc)"=0.075, "integral time (Ti, min)"=3.5e-06, "derivative time (Td, min)"=0.0}, "max value"=148.0}, {"PID gains"={"proportional gain (Kc)"=0.075, "integral time (Ti, min)"=3.5e-06, "derivative time (Td, min)"=0.0}, "max value"=150.0}, {"PID gains"={"proportional gain (Kc)"=0.0775, "integral time (Ti, min)"=3.5e-06, "derivative time (Td, min)"=0.0}, "max value"=155.0}, {"PID gains"={"proportional gain (Kc)"=0.117, "integral time (Ti, min)"=3.5e-06, "derivative time (Td, min)"=0.0}, "max value"=160.0}, {"PID gains"={"proportional gain (Kc)"=0.187, "integral time (Ti, min)"=3.5e-06, "derivative time (Td, min)"=0.0}, "max value"=165.0}, {"PID gains"={"proportional gain (Kc)"=0.28, "integral time (Ti, min)"=3.5e-06, "derivative time (Td, min)"=0.0}, "max value"=170.0}, {"PID gains"={"proportional gain (Kc)"=0.425, "integral time (Ti, min)"=3.5e-06, "derivative time (Td, min)"=0.0}, "max value"=175.0}, {"PID gains"={"proportional gain (Kc)"=0.615, "integral time (Ti, min)"=3.5e-06, "derivative time (Td, min)"=0.0}, "max value"=180.0}, {"PID gains"={"proportional gain (Kc)"=0.85, "integral time (Ti, min)"=3.5e-06, "derivative time (Td, min)"=0.0}, "max value"=185.0}, {"PID gains"={"proportional gain (Kc)"=1.0, "integral time (Ti, min)"=3.5e-06, "derivative time (Td, min)"=0.0}, "max value"=190.0}, {"PID gains"={"proportional gain (Kc)"=1.0, "integral time (Ti, min)"=3.5e-06, "derivative time (Td, min)"=0.0}, "max value"=195.0}, {"PID gains"={"proportional gain (Kc)"=1.0, "integral time (Ti, min)"=3.5e-06, "derivative time (Td, min)"=0.0}, "max value"=220.0}]  # ON PID gain schedule HyMu80#1 Needle MIN
          # "Updated on 2019-08-27"
          # "11/5/2018. Modified the PID gains for values 170 Gs and higher to make it more aggressive near the end."
          # "### values ABOVE ARE NOT UPDATED!!!! 3/25/2018"
          # "No discontinuity flux values will be selected\nNote: values that can leakage/ghosting/discontinuity in flux signals are not used.\nThis problem can be minimized by a number of techniques. However, I am not going to invest time \nin this right now. I can still generate fluxes of almost 200 Gs if Null Flux is -25 or -40 Gs. #WIM 1/16/2018"
          # "HyMu80#1 Needle Schedules Tuned on  1/11 & 12/2018 by #WIM\nfor fluxes:  ON/OFF\n145, 148, 150, 155, 160, 165, 170, 175, 180, 185, 190, 195 Gs\n220 Gs is for anything extra"
          # "HyMu80#1 Needle PID Parameters"
        }
        frame 2 {
          w862 = T2 [{"PID gains"={"proportional gain (Kc)"=0.053, "integral time (Ti, min)"=3.5e-06, "derivative time (Td, min)"=0.0}, "max value"=0.0}, {"PID gains"={"proportional gain (Kc)"=0.053, "integral time (Ti, min)"=3.5e-06, "derivative time (Td, min)"=0.0}, "max value"=75.0}, {"PID gains"={"proportional gain (Kc)"=0.053, "integral time (Ti, min)"=3.5e-06, "derivative time (Td, min)"=0.0}, "max value"=100.0}, {"PID gains"={"proportional gain (Kc)"=0.055, "integral time (Ti, min)"=3.5e-06, "derivative time (Td, min)"=0.0}, "max value"=125.0}, {"PID gains"={"proportional gain (Kc)"=0.055, "integral time (Ti, min)"=3.5e-06, "derivative time (Td, min)"=0.0}, "max value"=150.0}, {"PID gains"={"proportional gain (Kc)"=0.055, "integral time (Ti, min)"=3.5e-06, "derivative time (Td, min)"=0.0}, "max value"=160.0}, {"PID gains"={"proportional gain (Kc)"=0.055, "integral time (Ti, min)"=3.5e-06, "derivative time (Td, min)"=0.0}, "max value"=165.0}, {"PID gains"={"proportional gain (Kc)"=0.056, "integral time (Ti, min)"=3.5e-06, "derivative time (Td, min)"=0.0}, "max value"=170.0}, {"PID gains"={"proportional gain (Kc)"=0.057, "integral time (Ti, min)"=3.5e-06, "derivative time (Td, min)"=0.0}, "max value"=175.0}, {"PID gains"={"proportional gain (Kc)"=0.057, "integral time (Ti, min)"=3.5e-06, "derivative time (Td, min)"=0.0}, "max value"=180.0}, {"PID gains"={"proportional gain (Kc)"=0.057, "integral time (Ti, min)"=3.5e-06, "derivative time (Td, min)"=0.0}, "max value"=185.0}, {"PID gains"={"proportional gain (Kc)"=0.057, "integral time (Ti, min)"=3.5e-06, "derivative time (Td, min)"=0.0}, "max value"=190.0}, {"PID gains"={"proportional gain (Kc)"=0.057, "integral time (Ti, min)"=3.5e-06, "derivative time (Td, min)"=0.0}, "max value"=210.0}]  # OFF PID gain schedule HyMu80#1 Needle OPTIMIZED
          w861 = T2 [{"PID gains"={"proportional gain (Kc)"=0.053, "integral time (Ti, min)"=3.5e-06, "derivative time (Td, min)"=0.0}, "max value"=0.0}, {"PID gains"={"proportional gain (Kc)"=0.053, "integral time (Ti, min)"=3.5e-06, "derivative time (Td, min)"=0.0}, "max value"=75.0}, {"PID gains"={"proportional gain (Kc)"=0.053, "integral time (Ti, min)"=3.5e-06, "derivative time (Td, min)"=0.0}, "max value"=100.0}, {"PID gains"={"proportional gain (Kc)"=0.055, "integral time (Ti, min)"=3.5e-06, "derivative time (Td, min)"=0.0}, "max value"=125.0}, {"PID gains"={"proportional gain (Kc)"=0.057, "integral time (Ti, min)"=3.5e-06, "derivative time (Td, min)"=0.0}, "max value"=150.0}, {"PID gains"={"proportional gain (Kc)"=0.058, "integral time (Ti, min)"=3.5e-06, "derivative time (Td, min)"=0.0}, "max value"=160.0}, {"PID gains"={"proportional gain (Kc)"=0.065, "integral time (Ti, min)"=3.5e-06, "derivative time (Td, min)"=0.0}, "max value"=165.0}, {"PID gains"={"proportional gain (Kc)"=0.111, "integral time (Ti, min)"=3.5e-06, "derivative time (Td, min)"=0.0}, "max value"=170.0}, {"PID gains"={"proportional gain (Kc)"=0.185, "integral time (Ti, min)"=3.5e-06, "derivative time (Td, min)"=0.0}, "max value"=175.0}, {"PID gains"={"proportional gain (Kc)"=0.31, "integral time (Ti, min)"=3.5e-06, "derivative time (Td, min)"=0.0}, "max value"=180.0}, {"PID gains"={"proportional gain (Kc)"=0.55, "integral time (Ti, min)"=3.5e-06, "derivative time (Td, min)"=0.0}, "max value"=185.0}, {"PID gains"={"proportional gain (Kc)"=0.8, "integral time (Ti, min)"=3.5e-06, "derivative time (Td, min)"=0.0}, "max value"=190.0}, {"PID gains"={"proportional gain (Kc)"=0.8, "integral time (Ti, min)"=3.5e-06, "derivative time (Td, min)"=0.0}, "max value"=210.0}]  # ON PID gain schedule HyMu80#1 Needle OPTIMIZED
          w863 = T2 [{"PID gains"={"proportional gain (Kc)"=0.085, "integral time (Ti, min)"=3.5e-06, "derivative time (Td, min)"=0.0}, "max value"=0.0}, {"PID gains"={"proportional gain (Kc)"=0.085, "integral time (Ti, min)"=3.5e-06, "derivative time (Td, min)"=0.0}, "max value"=145.0}, {"PID gains"={"proportional gain (Kc)"=0.088, "integral time (Ti, min)"=3.5e-06, "derivative time (Td, min)"=0.0}, "max value"=148.0}, {"PID gains"={"proportional gain (Kc)"=0.091, "integral time (Ti, min)"=3.5e-06, "derivative time (Td, min)"=0.0}, "max value"=150.0}, {"PID gains"={"proportional gain (Kc)"=0.091, "integral time (Ti, min)"=3.5e-06, "derivative time (Td, min)"=0.0}, "max value"=155.0}, {"PID gains"={"proportional gain (Kc)"=0.092, "integral time (Ti, min)"=3.5e-06, "derivative time (Td, min)"=0.0}, "max value"=160.0}, {"PID gains"={"proportional gain (Kc)"=0.0935, "integral time (Ti, min)"=3.5e-06, "derivative time (Td, min)"=0.0}, "max value"=165.0}, {"PID gains"={"proportional gain (Kc)"=0.094, "integral time (Ti, min)"=3.5e-06, "derivative time (Td, min)"=0.0}, "max value"=170.0}, {"PID gains"={"proportional gain (Kc)"=0.0935, "integral time (Ti, min)"=3.5e-06, "derivative time (Td, min)"=0.0}, "max value"=175.0}, {"PID gains"={"proportional gain (Kc)"=0.097, "integral time (Ti, min)"=3.5e-06, "derivative time (Td, min)"=0.0}, "max value"=180.0}, {"PID gains"={"proportional gain (Kc)"=0.0945, "integral time (Ti, min)"=3.5e-06, "derivative time (Td, min)"=0.0}, "max value"=185.0}, {"PID gains"={"proportional gain (Kc)"=0.0945, "integral time (Ti, min)"=3.5e-06, "derivative time (Td, min)"=0.0}, "max value"=210.0}]  # OFF PID gain schedule HyMu80#2 Needle MAX
          w860 = T2 [{"PID gains"={"proportional gain (Kc)"=0.08, "integral time (Ti, min)"=3.5e-06, "derivative time (Td, min)"=0.0}, "max value"=0.0}, {"PID gains"={"proportional gain (Kc)"=0.08, "integral time (Ti, min)"=3.5e-06, "derivative time (Td, min)"=0.0}, "max value"=145.0}, {"PID gains"={"proportional gain (Kc)"=0.08, "integral time (Ti, min)"=3.5e-06, "derivative time (Td, min)"=0.0}, "max value"=148.0}, {"PID gains"={"proportional gain (Kc)"=0.082, "integral time (Ti, min)"=3.5e-06, "derivative time (Td, min)"=0.0}, "max value"=150.0}, {"PID gains"={"proportional gain (Kc)"=0.082, "integral time (Ti, min)"=3.5e-06, "derivative time (Td, min)"=0.0}, "max value"=155.0}, {"PID gains"={"proportional gain (Kc)"=0.082, "integral time (Ti, min)"=3.5e-06, "derivative time (Td, min)"=0.0}, "max value"=160.0}, {"PID gains"={"proportional gain (Kc)"=0.082, "integral time (Ti, min)"=3.5e-06, "derivative time (Td, min)"=0.0}, "max value"=165.0}, {"PID gains"={"proportional gain (Kc)"=0.083, "integral time (Ti, min)"=3.5e-06, "derivative time (Td, min)"=0.0}, "max value"=170.0}, {"PID gains"={"proportional gain (Kc)"=0.087, "integral time (Ti, min)"=3.5e-06, "derivative time (Td, min)"=0.0}, "max value"=175.0}, {"PID gains"={"proportional gain (Kc)"=0.092, "integral time (Ti, min)"=3.5e-06, "derivative time (Td, min)"=0.0}, "max value"=180.0}, {"PID gains"={"proportional gain (Kc)"=0.091, "integral time (Ti, min)"=3.5e-06, "derivative time (Td, min)"=0.0}, "max value"=185.0}, {"PID gains"={"proportional gain (Kc)"=0.091, "integral time (Ti, min)"=3.5e-06, "derivative time (Td, min)"=0.0}, "max value"=210.0}]  # OFF PID gain schedule HyMu80#2 Needle MIN
          w864 = T2 [{"PID gains"={"proportional gain (Kc)"=0.085, "integral time (Ti, min)"=3.5e-06, "derivative time (Td, min)"=0.0}, "max value"=0.0}, {"PID gains"={"proportional gain (Kc)"=0.085, "integral time (Ti, min)"=3.5e-06, "derivative time (Td, min)"=0.0}, "max value"=145.0}, {"PID gains"={"proportional gain (Kc)"=0.088, "integral time (Ti, min)"=3.5e-06, "derivative time (Td, min)"=0.0}, "max value"=148.0}, {"PID gains"={"proportional gain (Kc)"=0.113, "integral time (Ti, min)"=3.5e-06, "derivative time (Td, min)"=0.0}, "max value"=150.0}, {"PID gains"={"proportional gain (Kc)"=0.195, "integral time (Ti, min)"=3.5e-06, "derivative time (Td, min)"=0.0}, "max value"=155.0}, {"PID gains"={"proportional gain (Kc)"=0.31, "integral time (Ti, min)"=3.5e-06, "derivative time (Td, min)"=0.0}, "max value"=160.0}, {"PID gains"={"proportional gain (Kc)"=0.47, "integral time (Ti, min)"=3.5e-06, "derivative time (Td, min)"=0.0}, "max value"=165.0}, {"PID gains"={"proportional gain (Kc)"=0.725, "integral time (Ti, min)"=3.5e-06, "derivative time (Td, min)"=0.0}, "max value"=170.0}, {"PID gains"={"proportional gain (Kc)"=1.06, "integral time (Ti, min)"=3.5e-06, "derivative time (Td, min)"=0.0}, "max value"=175.0}, {"PID gains"={"proportional gain (Kc)"=1.3, "integral time (Ti, min)"=3.5e-06, "derivative time (Td, min)"=0.0}, "max value"=180.0}, {"PID gains"={"proportional gain (Kc)"=1.2, "integral time (Ti, min)"=3.5e-06, "derivative time (Td, min)"=0.0}, "max value"=185.0}, {"PID gains"={"proportional gain (Kc)"=1.2, "integral time (Ti, min)"=3.5e-06, "derivative time (Td, min)"=0.0}, "max value"=210.0}]  # ON PID gain schedule HyMu80#2 Needle MAX
          w865 = T2 [{"PID gains"={"proportional gain (Kc)"=0.08, "integral time (Ti, min)"=3.5e-06, "derivative time (Td, min)"=0.0}, "max value"=0.0}, {"PID gains"={"proportional gain (Kc)"=0.08, "integral time (Ti, min)"=3.5e-06, "derivative time (Td, min)"=0.0}, "max value"=145.0}, {"PID gains"={"proportional gain (Kc)"=0.08, "integral time (Ti, min)"=3.5e-06, "derivative time (Td, min)"=0.0}, "max value"=148.0}, {"PID gains"={"proportional gain (Kc)"=0.107, "integral time (Ti, min)"=3.5e-06, "derivative time (Td, min)"=0.0}, "max value"=150.0}, {"PID gains"={"proportional gain (Kc)"=0.188, "integral time (Ti, min)"=3.5e-06, "derivative time (Td, min)"=0.0}, "max value"=155.0}, {"PID gains"={"proportional gain (Kc)"=0.27, "integral time (Ti, min)"=3.5e-06, "derivative time (Td, min)"=0.0}, "max value"=160.0}, {"PID gains"={"proportional gain (Kc)"=0.435, "integral time (Ti, min)"=3.5e-06, "derivative time (Td, min)"=0.0}, "max value"=165.0}, {"PID gains"={"proportional gain (Kc)"=0.675, "integral time (Ti, min)"=3.5e-06, "derivative time (Td, min)"=0.0}, "max value"=170.0}, {"PID gains"={"proportional gain (Kc)"=0.945, "integral time (Ti, min)"=3.5e-06, "derivative time (Td, min)"=0.0}, "max value"=175.0}, {"PID gains"={"proportional gain (Kc)"=1.1, "integral time (Ti, min)"=3.5e-06, "derivative time (Td, min)"=0.0}, "max value"=180.0}, {"PID gains"={"proportional gain (Kc)"=1.15, "integral time (Ti, min)"=3.5e-06, "derivative time (Td, min)"=0.0}, "max value"=185.0}, {"PID gains"={"proportional gain (Kc)"=1.15, "integral time (Ti, min)"=3.5e-06, "derivative time (Td, min)"=0.0}, "max value"=210.0}]  # ON PID gain schedule HyMu80#2 Needle MIN
          # "Updated on 2019-08-14"
          # "### values HERE ARE NOT UPDATED!!!! 3/25/2018"
          # "No discontinuity flux values will be selected\nNote: values that can leakage/ghosting/discontinuity in flux signals are not used.\nThis problem can be minimized by a number of techniques. However, I am not going to invest time \nin this right now. I can still generate fluxes of almost 200 Gs if Null Flux is -25 or -40 Gs. #WIM 1/16/2018"
          # "HyMu80#2 Needle Schedules Tuned on  1/9 & 10/2018 by #WIM\nfor fluxes:  ON/OFF\n145, 148, 150, 155, 160, 165, 170, 175, 180, 185 Gs. \n220 Gs is for anything extra"
          # "HyMu80#2 Needle PID Parameters"
        }
      }
      n355 = shared-variable "NI-GenericDesktopPC-3A84958E\\Kopco PS Project Target Variables Library.lvlib\\Period OFF 1st Per Cycle"("1st OFF Length (s)") -> ()  [unwired: 1 in, 1 out]
      n356 = shared-variable "NI-GenericDesktopPC-3A84958E\\Kopco PS Project Target Variables Library.lvlib\\Sampling Rate"() -> (w815:dbl)  [unwired: 1 in, 1 out]
      n357 = Greater?(x=w816, y="1st OFF Length (s)") -> (0:w807:bool)
      n358 = case shown="True" w807 {
        tunnel: "1st OFF Length (s)" -> [_ w853]
        tunnel: w816 -> [_ w852]
        tunnel: w815 -> [_ w850]
        tunnel: w814 -> [w836 w846]
        tunnel: [w836 w847] -> w813
        tunnel: [w835 w848] -> w811
        tunnel: w812 -> [w835 w849]
        tunnel: w810 -> [w834 w844]
        tunnel: [w834 w845] -> w809
        tunnel: w808 -> [w833 w842]
        tunnel: [w833 w843] -> w800
        tunnel: w805 -> [w832 w840]
        tunnel: [w832 w839] -> w804
        frame False {
        }
        frame True {
          w841 = 0 ("index")
          n359 = Subtract(x=w852, y=w853) -> (x-y=w851:dbl)
          n360 = Multiply(x=w850, y=w851) -> (x*y=w838:dbl)
          n361 = To Quad Integer(1:w838) -> (0:w837:i64)
          n362 = Subtract(x=w840, y=w837) -> (x-y=w839:i64)
          n363 = Delete From Array(array=w846, length=w837, index=w841) -> (array with subset deleted=w847:bool[])  [unwired: 1 out]
          n364 = Delete From Array(array=w844, length=w837, index=w841) -> (array with subset deleted=w845:dbl[])  [unwired: 1 out]
          n365 = Delete From Array(array=w842, length=w837, index=w841) -> (array with subset deleted=w843:dbl[])  [unwired: 1 out]
          n366 = Delete From Array(array=w849, length=w837, index=w841) -> (array with subset deleted=w848:bool[])  [unwired: 1 out]
        }
      }
      n367 = shared-variable "NI-GenericDesktopPC-3A84958E\\Kopco PS Project Target Variables Library.lvlib\\Flux Setpoint ON Gs Relative"() -> (w794:dbl)  [unwired: 1 in, 1 out]
      n368 = shared-variable "NI-GenericDesktopPC-3A84958E\\Kopco PS Project Target Variables Library.lvlib\\Samples Total"(w804) -> ()  [unwired: 1 in, 1 out]
      n369 = Array Size(array=w800) -> (size(s)=w798:i32)
      n370 = Decrement(x=w798) -> (x-1=w797:i32)
      n371 = case "OFF Flux PID Gain Parameters: Interpolated vs. Fixed" shown="0, Default" w825 {
        tunnel: w794 -> [w869 w1014]
        tunnel: [w871 w1016] -> w819
        tunnel: w827 -> [w870 w1013]
        tunnel: w826 -> [w868 w1015]
        tunnel: w824 -> [w867 w1012]
        tunnel: w817 -> [w866 w1011]
        frame 0, Default {
          # "Interpolated Schedule"
          n372 = case "PID Paramter Aggressiveness" shown="1" w867 {
            tunnel: [w874 w906 w940 w981] -> w871
            tunnel: w870 -> [_ w904 w937 _]
            tunnel: w869 -> [w873 w905 w936 w980]
            tunnel: w868 -> [_ _ w938 w979]
            tunnel: w866 -> [w872 _ _ _]
            frame 0, Default {
              w884 = dbl[] []
              # "Rebundling PID Parameters without Names\nbut it should work the same"
              # "Optimized Interpolated"
              n373 = Array Size(array=w872) -> (size(s)=w886:i32)
              n374 = for {
                N: w886 -> [_]
                tunnel: w873 -> [w902]
                shift-right: [w900] -> w883
                shift-left: dbl[] [] -> [w901]
                tunnel: [w902] -> w876
                shift-right: [w898] -> w880
                shift-left: w884 -> [w899]
                shift-right: [w896] -> w882
                shift-left: w884 -> [w895]
                shift-right: [w897] -> w875
                shift-left: w884 -> [w894]
                tunnel: w872 -> [w893]
                i -> [w903]
                n375 = Index Array(array=w893, index=w903) -> (element=w892:T7)
                n376 = Unbundle(w892) -> ("PID gains"=w890:T1, "max value"=w891:dbl)
                n377 = Unbundle(w890) -> ("proportional gain (Kc)"=w887:dbl, "integral time (Ti, min)"=w889:dbl, "derivative time (Td, min)"=w888:dbl)
                n378 = Build Array (concatenate)(w901, w891) -> (w900:dbl[])
                n379 = Build Array (concatenate)(w899, w887) -> (w898:dbl[])
                n380 = Build Array (concatenate)(w895, w889) -> (w896:dbl[])
                n381 = Build Array (concatenate)(w894, w888) -> (w897:dbl[])
              }
              n382 = Threshold 1D Array(2:w876, 3:w883) -> (0:w881:dbl)  [unwired: 1 in]
              n383 = Interpolate 1D Array(1:w881, 2:w880) -> (0:w879:dbl)
              n384 = Interpolate 1D Array(1:w881, 2:w882) -> (0:w878:dbl)
              n385 = Interpolate 1D Array(1:w881, 2:w875) -> (0:w877:dbl)
              n386 = Bundle(w879, w878, w877) -> (w874:cluster{dbl, dbl, dbl})  [unwired: 1 in]
            }
            frame 1 {
              w916 = dbl[] []
              # "Rebundling PID Parameters without Names\nbut it should work the same"
              # "Minimum Interpolated"
              n387 = Array Size(array=w904) -> (size(s)=w918:i32)
              n388 = for {
                N: w918 -> [_]
                tunnel: w905 -> [w934]
                shift-right: [w932] -> w915
                shift-left: dbl[] [] -> [w933]
                tunnel: [w934] -> w908
                shift-right: [w930] -> w912
                shift-left: w916 -> [w931]
                shift-right: [w928] -> w914
                shift-left: w916 -> [w927]
                shift-right: [w929] -> w907
                shift-left: w916 -> [w926]
                tunnel: w904 -> [w925]
                i -> [w935]
                n389 = Index Array(array=w925, index=w935) -> (element=w924:T7)
                n390 = Unbundle(w924) -> ("PID gains"=w922:T1, "max value"=w923:dbl)
                n391 = Unbundle(w922) -> ("proportional gain (Kc)"=w919:dbl, "integral time (Ti, min)"=w921:dbl, "derivative time (Td, min)"=w920:dbl)
                n392 = Build Array (concatenate)(w933, w923) -> (w932:dbl[])
                n393 = Build Array (concatenate)(w931, w919) -> (w930:dbl[])
                n394 = Build Array (concatenate)(w927, w921) -> (w928:dbl[])
                n395 = Build Array (concatenate)(w926, w920) -> (w929:dbl[])
              }
              n396 = Threshold 1D Array(2:w908, 3:w915) -> (0:w913:dbl)  [unwired: 1 in]
              n397 = Interpolate 1D Array(1:w913, 2:w912) -> (0:w911:dbl)
              n398 = Interpolate 1D Array(1:w913, 2:w914) -> (0:w910:dbl)
              n399 = Interpolate 1D Array(1:w913, 2:w907) -> (0:w909:dbl)
              n400 = Bundle(w911, w910, w909) -> (w906:cluster{dbl, dbl, dbl})  [unwired: 1 in]
            }
            frame 2 {
              w948 = dbl[] []
              # "Average Interpolated"
              n401 = Array Size(array=w937) -> (size(s)=w950:i32)
              n402 = for {
                N: w950 -> [_]
                tunnel: w937 -> [w978]
                shift-right: [w974] -> w946
                shift-left: dbl[] [] -> [w975]
                shift-right: [w972] -> w943
                shift-left: w948 -> [w973]
                shift-right: [w970] -> w944
                shift-left: w948 -> [w969]
                shift-right: [w971] -> w945
                shift-left: w948 -> [w968]
                tunnel: w938 -> [w965]
                i -> [w964]
                n403 = Index Array(array=w978, index=w964) -> (element=w977:T7)
                n404 = Index Array(array=w965, index=w964) -> (element=w967:T7)
                n405 = Unbundle(w977) -> ("PID gains"=w976:T1)  [unwired: 1 out]
                n406 = Unbundle(w967) -> ("PID gains"=w963:T1, "max value"=w966:dbl)
                n407 = Unbundle(w976) -> ("proportional gain (Kc)"=w961:dbl, "integral time (Ti, min)"=w957:dbl, "derivative time (Td, min)"=w955:dbl)
                n408 = Build Array (concatenate) "Flux Cutoff"(w975, w966) -> (w974:dbl[])
                n409 = Unbundle(w963) -> ("proportional gain (Kc)"=w962:dbl, "integral time (Ti, min)"=w956:dbl, "derivative time (Td, min)"=w952:dbl)
                n410 = Build Array(w961, w962) -> (w960:dbl[])
                n411 = Build Array(w957, w956) -> (w959:dbl[])
                n412 = call-poly <vilib>:"Mean.vi"("X"=w960) -> ("mean"=w951:dbl)  [unwired: 1 out]
                n413 = Build Array(w955, w952) -> (w958:dbl[])
                n414 = call-poly <vilib>:"Mean.vi"("X"=w959) -> ("mean"=w954:dbl)  [unwired: 1 out]
                n415 = call-poly <vilib>:"Mean.vi"("X"=w958) -> ("mean"=w953:dbl)  [unwired: 1 out]
                n416 = Build Array (concatenate) "K_c"(w973, w951) -> (w972:dbl[])
                n417 = Build Array (concatenate) "T_i"(w969, w954) -> (w970:dbl[])
                n418 = Build Array (concatenate) "T_d"(w968, w953) -> (w971:dbl[])
              }
              n419 = Threshold 1D Array(2:w936, 3:w946) -> (0:w947:dbl)  [unwired: 1 in]
              n420 = Interpolate 1D Array(1:w947, 2:w943) -> (0:w942:dbl)
              n421 = Interpolate 1D Array(1:w947, 2:w944) -> (0:w941:dbl)
              n422 = Interpolate 1D Array(1:w947, 2:w945) -> (0:w939:dbl)
              n423 = Bundle(w942, w941, w939) -> (w940:cluster{dbl, dbl, dbl})  [unwired: 1 in]
            }
            frame 3 {
              w991 = dbl[] []
              # "Maximum Interpolated"
              # "Rebundling PID Parameters without Names\nbut it should work the same"
              n424 = Array Size(array=w979) -> (size(s)=w993:i32)
              n425 = for {
                N: w993 -> [_]
                tunnel: w980 -> [w1009]
                shift-right: [w1007] -> w990
                shift-left: dbl[] [] -> [w1008]
                tunnel: [w1009] -> w983
                shift-right: [w1005] -> w987
                shift-left: w991 -> [w1006]
                shift-right: [w1003] -> w989
                shift-left: w991 -> [w1002]
                shift-right: [w1004] -> w982
                shift-left: w991 -> [w1001]
                tunnel: w979 -> [w1000]
                i -> [w1010]
                n426 = Index Array(array=w1000, index=w1010) -> (element=w999:T7)
                n427 = Unbundle(w999) -> ("PID gains"=w997:T1, "max value"=w998:dbl)
                n428 = Unbundle(w997) -> ("proportional gain (Kc)"=w994:dbl, "integral time (Ti, min)"=w996:dbl, "derivative time (Td, min)"=w995:dbl)
                n429 = Build Array (concatenate)(w1008, w998) -> (w1007:dbl[])
                n430 = Build Array (concatenate)(w1006, w994) -> (w1005:dbl[])
                n431 = Build Array (concatenate)(w1002, w996) -> (w1003:dbl[])
                n432 = Build Array (concatenate)(w1001, w995) -> (w1004:dbl[])
              }
              n433 = Threshold 1D Array(2:w983, 3:w990) -> (0:w988:dbl)  [unwired: 1 in]
              n434 = Interpolate 1D Array(1:w988, 2:w987) -> (0:w986:dbl)
              n435 = Interpolate 1D Array(1:w988, 2:w989) -> (0:w985:dbl)
              n436 = Interpolate 1D Array(1:w988, 2:w982) -> (0:w984:dbl)
              n437 = Bundle(w986, w985, w984) -> (w981:cluster{dbl, dbl, dbl})  [unwired: 1 in]
            }
          }
        }
        frame 1 {
          # "Fixed Schedule"
          n438 = case "PID Paramter Aggressiveness" shown="2" w1012 {
            tunnel: [w1019 w1022 w1026 w1043] -> w1016
            tunnel: w1015 -> [_ _ w1024 w1042]
            tunnel: w1014 -> [w1018 w1021 w1023 w1041]
            tunnel: w1013 -> [_ w1020 w1025 _]
            tunnel: w1011 -> [w1017 _ _ _]
            frame 0, Default {
              # "Optimized Fixed"
              n439 = call-poly <vilib>:"PID Gain Schedule.vi"("PID gain schedule"=w1017, "gain scheduling value"=w1018) -> ("PID gains out"=w1019:T1)  [unwired: 2 in, 1 out]
            }
            frame 1 {
              # "Minimum Fixed"
              n440 = call-poly <vilib>:"PID Gain Schedule.vi"("PID gain schedule"=w1020, "gain scheduling value"=w1021) -> ("PID gains out"=w1022:T1)  [unwired: 2 in, 1 out]
            }
            frame 2 {
              # "Averaged Fixed"
              n441 = call-poly <vilib>:"PID Gain Schedule.vi"("PID gain schedule"=w1025, "gain scheduling value"=w1023) -> ("PID gains out"=w1031:T1)  [unwired: 2 in, 1 out]
              n442 = call-poly <vilib>:"PID Gain Schedule.vi"("PID gain schedule"=w1024, "gain scheduling value"=w1023) -> ("PID gains out"=w1030:T1)  [unwired: 2 in, 1 out]
              n443 = Unbundle(w1031) -> ("proportional gain (Kc)"=w1039:dbl, "integral time (Ti, min)"=w1035:dbl, "derivative time (Td, min)"=w1033:dbl)
              n444 = Unbundle(w1030) -> ("proportional gain (Kc)"=w1040:dbl, "integral time (Ti, min)"=w1034:dbl, "derivative time (Td, min)"=w1032:dbl)
              n445 = Build Array(w1039, w1040) -> (w1038:dbl[])
              n446 = Build Array(w1035, w1034) -> (w1037:dbl[])
              n447 = call-poly <vilib>:"Mean.vi"("X"=w1038) -> ("mean"=w1027:dbl)  [unwired: 1 out]
              n448 = Build Array(w1033, w1032) -> (w1036:dbl[])
              n449 = call-poly <vilib>:"Mean.vi"("X"=w1037) -> ("mean"=w1029:dbl)  [unwired: 1 out]
              n450 = call-poly <vilib>:"Mean.vi"("X"=w1036) -> ("mean"=w1028:dbl)  [unwired: 1 out]
              n451 = Bundle("mean"=w1027, "mean"=w1029, "mean"=w1028) -> (w1026:cluster{"mean":dbl, "mean":dbl, "mean":dbl})  [unwired: 1 in]
            }
            frame 3 {
              # "Maximum Fixed"
              n452 = call-poly <vilib>:"PID Gain Schedule.vi"("PID gain schedule"=w1042, "gain scheduling value"=w1041) -> ("PID gains out"=w1043:T1)  [unwired: 2 in, 1 out]
            }
          }
        }
      }
      "Suggested PID gains OFF" <- w819
      n453 = case "ON Flux PID Gain Parameters: Interpolated vs. Fixed" shown="1" w825 {
        tunnel: w794 -> [w1046 w1191]
        tunnel: [w1048 w1193] -> w820
        tunnel: w824 -> [w1049 w1194]
        tunnel: w829 -> [w1047 w1190]
        tunnel: w828 -> [w1045 w1192]
        tunnel: w818 -> [w1044 w1189]
        frame 0, Default {
          # "Interpolated Schedule"
          n454 = case "PID Paramter Aggressiveness" shown="0, Default" w1049 {
            tunnel: [w1052 w1084 w1118 w1159] -> w1048
            tunnel: w1047 -> [_ w1082 w1115 _]
            tunnel: w1046 -> [w1051 w1083 w1114 w1158]
            tunnel: w1045 -> [_ _ w1116 w1157]
            tunnel: w1044 -> [w1050 _ _ _]
            frame 0, Default {
              w1062 = dbl[] []
              # "Rebundling PID Parameters without Names\nbut it should work the same"
              # "Optimized Interpolated"
              n455 = Array Size(array=w1050) -> (size(s)=w1064:i32)
              n456 = for {
                N: w1064 -> [_]
                tunnel: w1051 -> [w1080]
                shift-right: [w1078] -> w1061
                shift-left: dbl[] [] -> [w1079]
                tunnel: [w1080] -> w1054
                shift-right: [w1076] -> w1058
                shift-left: w1062 -> [w1077]
                shift-right: [w1074] -> w1060
                shift-left: w1062 -> [w1073]
                shift-right: [w1075] -> w1053
                shift-left: w1062 -> [w1072]
                tunnel: w1050 -> [w1071]
                i -> [w1081]
                n457 = Index Array(array=w1071, index=w1081) -> (element=w1070:T7)
                n458 = Unbundle(w1070) -> ("PID gains"=w1068:T1, "max value"=w1069:dbl)
                n459 = Unbundle(w1068) -> ("proportional gain (Kc)"=w1065:dbl, "integral time (Ti, min)"=w1067:dbl, "derivative time (Td, min)"=w1066:dbl)
                n460 = Build Array (concatenate)(w1079, w1069) -> (w1078:dbl[])
                n461 = Build Array (concatenate)(w1077, w1065) -> (w1076:dbl[])
                n462 = Build Array (concatenate)(w1073, w1067) -> (w1074:dbl[])
                n463 = Build Array (concatenate)(w1072, w1066) -> (w1075:dbl[])
              }
              n464 = Threshold 1D Array(2:w1054, 3:w1061) -> (0:w1059:dbl)  [unwired: 1 in]
              n465 = Interpolate 1D Array(1:w1059, 2:w1058) -> (0:w1057:dbl)
              n466 = Interpolate 1D Array(1:w1059, 2:w1060) -> (0:w1056:dbl)
              n467 = Interpolate 1D Array(1:w1059, 2:w1053) -> (0:w1055:dbl)
              n468 = Bundle(w1057, w1056, w1055) -> (w1052:cluster{dbl, dbl, dbl})  [unwired: 1 in]
            }
            frame 1 {
              w1094 = dbl[] []
              # "Rebundling PID Parameters without Names\nbut it should work the same"
              # "Minimum Interpolated"
              n469 = Array Size(array=w1082) -> (size(s)=w1096:i32)
              n470 = for {
                N: w1096 -> [_]
                tunnel: w1083 -> [w1112]
                shift-right: [w1110] -> w1093
                shift-left: dbl[] [] -> [w1111]
                tunnel: [w1112] -> w1086
                shift-right: [w1108] -> w1090
                shift-left: w1094 -> [w1109]
                shift-right: [w1106] -> w1092
                shift-left: w1094 -> [w1105]
                shift-right: [w1107] -> w1085
                shift-left: w1094 -> [w1104]
                tunnel: w1082 -> [w1103]
                i -> [w1113]
                n471 = Index Array(array=w1103, index=w1113) -> (element=w1102:T7)
                n472 = Unbundle(w1102) -> ("PID gains"=w1100:T1, "max value"=w1101:dbl)
                n473 = Unbundle(w1100) -> ("proportional gain (Kc)"=w1097:dbl, "integral time (Ti, min)"=w1099:dbl, "derivative time (Td, min)"=w1098:dbl)
                n474 = Build Array (concatenate)(w1111, w1101) -> (w1110:dbl[])
                n475 = Build Array (concatenate)(w1109, w1097) -> (w1108:dbl[])
                n476 = Build Array (concatenate)(w1105, w1099) -> (w1106:dbl[])
                n477 = Build Array (concatenate)(w1104, w1098) -> (w1107:dbl[])
              }
              n478 = Threshold 1D Array(2:w1086, 3:w1093) -> (0:w1091:dbl)  [unwired: 1 in]
              n479 = Interpolate 1D Array(1:w1091, 2:w1090) -> (0:w1089:dbl)
              n480 = Interpolate 1D Array(1:w1091, 2:w1092) -> (0:w1088:dbl)
              n481 = Interpolate 1D Array(1:w1091, 2:w1085) -> (0:w1087:dbl)
              n482 = Bundle(w1089, w1088, w1087) -> (w1084:cluster{dbl, dbl, dbl})  [unwired: 1 in]
            }
            frame 2 {
              w1126 = dbl[] []
              # "Average Interpolated"
              n483 = Array Size(array=w1115) -> (size(s)=w1128:i32)
              n484 = for {
                N: w1128 -> [_]
                tunnel: w1115 -> [w1156]
                shift-right: [w1152] -> w1124
                shift-left: dbl[] [] -> [w1153]
                shift-right: [w1150] -> w1121
                shift-left: w1126 -> [w1151]
                shift-right: [w1148] -> w1122
                shift-left: w1126 -> [w1147]
                shift-right: [w1149] -> w1123
                shift-left: w1126 -> [w1146]
                tunnel: w1116 -> [w1143]
                i -> [w1142]
                n485 = Index Array(array=w1156, index=w1142) -> (element=w1155:T7)
                n486 = Index Array(array=w1143, index=w1142) -> (element=w1145:T7)
                n487 = Unbundle(w1155) -> ("PID gains"=w1154:T1)  [unwired: 1 out]
                n488 = Unbundle(w1145) -> ("PID gains"=w1141:T1, "max value"=w1144:dbl)
                n489 = Unbundle(w1154) -> ("proportional gain (Kc)"=w1139:dbl, "integral time (Ti, min)"=w1135:dbl, "derivative time (Td, min)"=w1133:dbl)
                n490 = Build Array (concatenate) "Flux Cutoff"(w1153, w1144) -> (w1152:dbl[])
                n491 = Unbundle(w1141) -> ("proportional gain (Kc)"=w1140:dbl, "integral time (Ti, min)"=w1134:dbl, "derivative time (Td, min)"=w1130:dbl)
                n492 = Build Array(w1139, w1140) -> (w1138:dbl[])
                n493 = Build Array(w1135, w1134) -> (w1137:dbl[])
                n494 = call-poly <vilib>:"Mean.vi"("X"=w1138) -> ("mean"=w1129:dbl)  [unwired: 1 out]
                n495 = Build Array(w1133, w1130) -> (w1136:dbl[])
                n496 = call-poly <vilib>:"Mean.vi"("X"=w1137) -> ("mean"=w1132:dbl)  [unwired: 1 out]
                n497 = call-poly <vilib>:"Mean.vi"("X"=w1136) -> ("mean"=w1131:dbl)  [unwired: 1 out]
                n498 = Build Array (concatenate) "K_c"(w1151, w1129) -> (w1150:dbl[])
                n499 = Build Array (concatenate) "T_i"(w1147, w1132) -> (w1148:dbl[])
                n500 = Build Array (concatenate) "T_d"(w1146, w1131) -> (w1149:dbl[])
              }
              n501 = Threshold 1D Array(2:w1114, 3:w1124) -> (0:w1125:dbl)  [unwired: 1 in]
              n502 = Interpolate 1D Array(1:w1125, 2:w1121) -> (0:w1120:dbl)
              n503 = Interpolate 1D Array(1:w1125, 2:w1122) -> (0:w1119:dbl)
              n504 = Interpolate 1D Array(1:w1125, 2:w1123) -> (0:w1117:dbl)
              n505 = Bundle(w1120, w1119, w1117) -> (w1118:cluster{dbl, dbl, dbl})  [unwired: 1 in]
            }
            frame 3 {
              w1169 = dbl[] []
              # "Maximum Interpolated"
              # "Rebundling PID Parameters without Names\nbut it should work the same"
              n506 = Array Size(array=w1157) -> (size(s)=w1171:i32)
              n507 = for {
                N: w1171 -> [_]
                tunnel: w1158 -> [w1187]
                shift-right: [w1185] -> w1168
                shift-left: dbl[] [] -> [w1186]
                tunnel: [w1187] -> w1161
                shift-right: [w1183] -> w1165
                shift-left: w1169 -> [w1184]
                shift-right: [w1181] -> w1167
                shift-left: w1169 -> [w1180]
                shift-right: [w1182] -> w1160
                shift-left: w1169 -> [w1179]
                tunnel: w1157 -> [w1178]
                i -> [w1188]
                n508 = Index Array(array=w1178, index=w1188) -> (element=w1177:T7)
                n509 = Unbundle(w1177) -> ("PID gains"=w1175:T1, "max value"=w1176:dbl)
                n510 = Unbundle(w1175) -> ("proportional gain (Kc)"=w1172:dbl, "integral time (Ti, min)"=w1174:dbl, "derivative time (Td, min)"=w1173:dbl)
                n511 = Build Array (concatenate)(w1186, w1176) -> (w1185:dbl[])
                n512 = Build Array (concatenate)(w1184, w1172) -> (w1183:dbl[])
                n513 = Build Array (concatenate)(w1180, w1174) -> (w1181:dbl[])
                n514 = Build Array (concatenate)(w1179, w1173) -> (w1182:dbl[])
              }
              n515 = Threshold 1D Array(2:w1161, 3:w1168) -> (0:w1166:dbl)  [unwired: 1 in]
              n516 = Interpolate 1D Array(1:w1166, 2:w1165) -> (0:w1164:dbl)
              n517 = Interpolate 1D Array(1:w1166, 2:w1167) -> (0:w1163:dbl)
              n518 = Interpolate 1D Array(1:w1166, 2:w1160) -> (0:w1162:dbl)
              n519 = Bundle(w1164, w1163, w1162) -> (w1159:cluster{dbl, dbl, dbl})  [unwired: 1 in]
            }
          }
        }
        frame 1 {
          # "Fixed Schedule"
          n520 = case "PID Paramter Aggressiveness" shown="2" w1194 {
            tunnel: [w1195 w1200 w1204 w1221] -> w1193
            tunnel: w1192 -> [_ _ w1201 w1220]
            tunnel: w1191 -> [w1196 w1199 w1202 w1219]
            tunnel: w1190 -> [_ w1198 w1203 _]
            tunnel: w1189 -> [w1197 _ _ _]
            frame 0 {
              # "Optimized Fixed"
              n521 = call-poly <vilib>:"PID Gain Schedule.vi"("PID gain schedule"=w1197, "gain scheduling value"=w1196) -> ("PID gains out"=w1195:T1)  [unwired: 2 in, 1 out]
            }
            frame 1, Default {
              # "Minimum Fixed"
              n522 = call-poly <vilib>:"PID Gain Schedule.vi"("PID gain schedule"=w1198, "gain scheduling value"=w1199) -> ("PID gains out"=w1200:T1)  [unwired: 2 in, 1 out]
            }
            frame 2 {
              # "Averaged Fixed"
              n523 = call-poly <vilib>:"PID Gain Schedule.vi"("PID gain schedule"=w1203, "gain scheduling value"=w1202) -> ("PID gains out"=w1209:T1)  [unwired: 2 in, 1 out]
              n524 = call-poly <vilib>:"PID Gain Schedule.vi"("PID gain schedule"=w1201, "gain scheduling value"=w1202) -> ("PID gains out"=w1208:T1)  [unwired: 2 in, 1 out]
              n525 = Unbundle(w1209) -> ("proportional gain (Kc)"=w1217:dbl, "integral time (Ti, min)"=w1213:dbl, "derivative time (Td, min)"=w1211:dbl)
              n526 = Unbundle(w1208) -> ("proportional gain (Kc)"=w1218:dbl, "integral time (Ti, min)"=w1212:dbl, "derivative time (Td, min)"=w1210:dbl)
              n527 = Build Array(w1217, w1218) -> (w1216:dbl[])
              n528 = Build Array(w1213, w1212) -> (w1215:dbl[])
              n529 = call-poly <vilib>:"Mean.vi"("X"=w1216) -> ("mean"=w1205:dbl)  [unwired: 1 out]
              n530 = Build Array(w1211, w1210) -> (w1214:dbl[])
              n531 = call-poly <vilib>:"Mean.vi"("X"=w1215) -> ("mean"=w1207:dbl)  [unwired: 1 out]
              n532 = call-poly <vilib>:"Mean.vi"("X"=w1214) -> ("mean"=w1206:dbl)  [unwired: 1 out]
              n533 = Bundle("mean"=w1205, "mean"=w1207, "mean"=w1206) -> (w1204:cluster{"mean":dbl, "mean":dbl, "mean":dbl})  [unwired: 1 in]
            }
            frame 3 {
              # "Maximum Fixed"
              n534 = call-poly <vilib>:"PID Gain Schedule.vi"("PID gain schedule"=w1220, "gain scheduling value"=w1219) -> ("PID gains out"=w1221:T1)  [unwired: 2 in, 1 out]
            }
          }
        }
      }
      "Suggested PID gains ON" <- w820
      n535 = Array Subset(array=w800, index=w797, length=1) -> (w796:dbl[])
      n536 = Delete From Array "Last Point\n AO (V)"(array=w796) -> (deleted portion=w795:dbl)  [unwired: 2 in, 1 out]
      "Final AO (V)" <- w795
      n537 = shared-variable "NI-GenericDesktopPC-3A84958E\\Kopco PS Project Target Variables Library.lvlib\\FinalAOV"(w795) -> ()  [unwired: 1 in, 1 out]
      n538 = shared-variable "NI-GenericDesktopPC-3A84958E\\Kopco PS Project Target Variables Library.lvlib\\Digital Trigger"() -> (w803:bool)  [unwired: 1 in, 1 out]
      n539 = shared-variable "NI-GenericDesktopPC-3A84958E\\Kopco PS Project Target Variables Library.lvlib\\Data Upload"() -> (w802:bool)  [unwired: 1 in, 1 out]
      n540 = case shown="True" w803 {
        frame False {
        }
        frame True {
          n541 = shared-variable "NI-GenericDesktopPC-3A84958E\\Kopco PS Project Target Variables Library.lvlib\\Digital Trigger"(FALSE ("Digital Trigger")) -> ()  [unwired: 1 in, 1 out]
        }
      }
      n542 = case shown="True" w802 {
        frame False {
        }
        frame True {
          n543 = shared-variable "NI-GenericDesktopPC-3A84958E\\Kopco PS Project Target Variables Library.lvlib\\Data Upload"(FALSE ("Digital Trigger")) -> ()  [unwired: 1 in, 1 out]
        }
      }
    }
    frame #17 {
      # "Bound to \"PID Parameters Selected\"\nshared global variable"
      # "Bound to \"Data Logger Running\"\nshared global variable."
      # "Flux ON/OFF Logical"
      # "AO values of current"
      # "Sampling Rate"
      # "Flux Control Sequence"
      # "Mini DeGauss AO Sequence, Normalized"
      # "Mini DeGauss Logical"
      # "Ask if you want to tweak the current parameters. This is useful in \ninterpolation cases, and when values change over time"
      # "Step 4 Specifying PID Parameters"
      n544 = flat-sequence {
        tunnel: w1235 -> [w1240]
        tunnel: w1236 -> [w1243]
        tunnel: [w1244] -> w1233
        tunnel: [w1242] -> w1225
        tunnel: [w1241] -> w1224
        tunnel: [w1254] -> w1234
        tunnel: [w1252] -> w1232
        tunnel: [w1251] -> w1231
        tunnel: w1233 -> [w1250]
        tunnel: w1225 -> [w1253]
        tunnel: w1224 -> [w1249]
        frame #0 {
          n545 = while {
            tunnel: ["Start Null Flux Adjustment 2"] -> _
            tunnel: ["Keep Null Flux Running \n       Until Next Step? 2"] -> w1244
            tunnel: w1243 -> [w1246]
            tunnel: [w1246] -> w1242
            tunnel: [w1245] -> w1241
            tunnel: w1240 -> [w1245]
            stop <- "Start Null Flux Adjustment 2" stop-if-true
          }
        }
        frame #1 {
          n546 = case shown="False" w1250 {
            tunnel: [TRUE TRUE] -> w1254
            tunnel: w1253 -> [w1255 _]
            tunnel: [w1255 "Tweaked PID gains ON"] -> w1252
            tunnel: [w1256 "Tweaked PID gains OFF"] -> w1251
            tunnel: w1249 -> [w1256 _]
            frame False {
              # "No Change in PID Parameters"
            }
            frame True {
            }
          }
        }
      }
      n547 = shared-variable "NI-GenericDesktopPC-3A84958E\\Kopco PS Project Target Variables Library.lvlib\\PID Parameters Selected"(w1234) -> ()  [unwired: 1 in, 1 out]
      "PID gains ON Chosen" <- w1232
      "PID gains OFF Chosen" <- w1231
    }
    frame #18 {
      w1286 = -1 items=["default"=-1, "RSE"=10083, "NRSE"=10078, "Differential"=10106, "Pseudodifferential"=12529] ("Terminal Configuration")
      w1291 = "Dev2/ao0"  # Power Supply Control
      w1290 = 12522 items=["Finite Samples"=10178, "Continuous Samples"=10123, "Hardware Timed Single Point"=12522]  # Sample Mode
      w1296 = 10106 items=["default"=-1, "RSE"=10083, "NRSE"=10078, "Differential"=10106, "Pseudodifferential"=12529] ("Terminal Configuration")
      w1299 = 12522 items=["Finite Samples"=10178, "Continuous Samples"=10123, "Hardware Timed Single Point"=12522]  # Sample Mode
      # "1/4 wave to get the main points of the\n mini DeGauss waveform 3/12/2018"
      # "Reversed order of AI7 & AI3 on 4/11/2018 to \nminimize leakage to Channel 7"
      # "# of samples of Mini DeGauss"
      # "Fixed by WIM on 3/5/2018 to keep the old AO value"
      # "Step 5 Preparing DAQ for Waveform"
      # "Total Number of Samples"
      n548 = shared-variable "NI-GenericDesktopPC-3A84958E\\Kopco PS Project Target Variables Library.lvlib\\Channels AI List"() -> (w1262:string)  [unwired: 1 in, 1 out]
      n549 = shared-variable "NI-GenericDesktopPC-3A84958E\\Kopco PS Project Target Variables Library.lvlib\\Sampling Rate"() -> (w1261:dbl)  [unwired: 1 in, 1 out]
      n550 = call-poly <vilib>:"DAQmx Create Virtual Channel.vi"("maximum value"=5.0 ("Max Voltage"), "minimum value"=0.0 ("Min Voltage"), "input terminal configuration"=w1296, "physical channels"=w1262) -> ("task out"=w1297:refnum<k21>, "error out"=w1298:errorcluster)  [unwired: 10 in]
      n551 = call-poly <vilib>:"DAQmx Create Virtual Channel.vi"("maximum value"=10.0, "minimum value"=-10.0, "output terminal configuration"=w1286, "physical channels"=w1291) -> ("task out"=w1293:refnum<k21>, "error out"=w1292:errorcluster)  [unwired: 10 in]
      n552 = shared-variable "NI-GenericDesktopPC-3A84958E\\Kopco PS Project Target Variables Library.lvlib\\Zero Flux Calibrated Core"() -> (w1276:dbl)  [unwired: 1 in, 1 out]
      n553 = call-poly <vilib>:"DAQmx Timing.vi"("task/channels in"=w1297, "sample mode"=w1299, "rate"=w1261, "error in"=w1298) -> ("task out"=w1289:refnum<k21>, "error out"=w1285:errorcluster)  [unwired: 10 in]
      n554 = call "Get Terminal Name with Device Prefix.vi"("error in"=w1285, "Local Terminal Name"="ai/SampleClock", "task/channels in"=w1289) -> ("error out"=w1278:errorcluster, "Terminal Name with Device Prefix"=w1284:tag, "task out"=w1279:refnum<k21>)  [unwired: 6 in]
      n555 = call-poly <vilib>:"DAQmx Timing.vi"("task/channels in"=w1293, "sample mode"=w1290, "rate"=w1261, "source"=w1284, "error in"=w1292) -> ("task out"=w1281:refnum<k21>, "error out"=w1282:errorcluster)  [unwired: 9 in]
      n556 = call <vilib>:"DAQmx Start Task.vi"("task/channels in"=w1281, "error in"=w1282) -> ("task out"=w1272:refnum<k21>, "error out"=w1271:errorcluster)  [unwired: 12 in]
      n557 = Merge Errors(w1278, w1271) -> (w1280:errorcluster)
    }
    frame #19 {
      # "1/4 wave to get the main points of the mini DeGauss waveform 3/12/2018"
      n558 = while "Digital Trigger from Master Data Logger" {
        tunnel: [w1348] -> w1330
        tunnel: w1331 -> [w1348]
        tunnel: w1329 -> [w1347]
        tunnel: [w1347] -> w1328
        tunnel: w1327 -> [w1346]
        tunnel: [w1346] -> w1326
        tunnel: [w1345] -> w1325
        tunnel: w1324 -> [w1345]
        tunnel: w1323 -> [w1344]
        tunnel: [w1344] -> w1322
        tunnel: w1321 -> [w1343]
        tunnel: [w1343] -> w1320
        tunnel: w1319 -> [w1342]
        tunnel: [w1342] -> w1318
        tunnel: w1317 -> [w1341]
        tunnel: [w1341] -> w1316
        tunnel: w1315 -> [w1340]
        tunnel: [w1340] -> w1314
        tunnel: w1313 -> [w1339]
        tunnel: [w1339] -> w1312
        tunnel: w1311 -> [w1338]
        tunnel: [w1338] -> w1310
        tunnel: w1309 -> [w1337]
        tunnel: [w1337] -> w1308
        tunnel: w1307 -> [w1336]
        tunnel: [w1336] -> w1306
        tunnel: w1305 -> [w1335]
        tunnel: [w1335] -> w1304
        tunnel: w1303 -> [w1332]
        tunnel: w1302 -> [w1333]
        tunnel: [w1333] -> w1301
        tunnel: [w1332] -> w1300
        stop <- w1349 stop-if-true
        # "Bound to Digital Trigger Real-Time Shared Variable"
        n559 = shared-variable "NI-GenericDesktopPC-3A84958E\\Kopco PS Project Target Variables Library.lvlib\\Digital Trigger"() -> (w1349:bool)  [unwired: 1 in, 1 out]
        "DigitalTrigger" <- w1349
        n560 = Wait (ms)(milliseconds to wait=u32 1) -> ()  [unwired: 1 out]
      }
    }
    frame #20 {
      w1362 = 0  # Last Current AO Index
      w1367 = 0  # 0-14 Mini DeGauss Sample Counter Initialized
      w1388 = T8 1 items=["All Elements Read From Stream", "All Elements Available for Reading"] ("wait condition")
      w1366 = 30  # # of samples pushed  to PID loop
      w1412 = 0  # 0-29 PID Sample Counter Initialized
      # "Reset Digital trigger in case program gets stuck"
      # "Moved Outside 3/31/2018"
      # "# of samples of Mini DeGauss"
      # "Bound to \"DataUpload\" shared variable"
      # "Abs(AO_nf) + Abs(AO_on,last)"
      # "AO_Last"
      # "Set PID \nReinitialize as true\ninitialially"
      # "Mini DeGauss AO Sequence, Normalized"
      # "Mini DeGauss PID CTRL ON/OFF Logical"
      # "AO,last"
      # "Step 5 Pushing Data to Datalogger"
      # "Step 5 Carrying out Waveform"
      # "ON PID Gain"
      # "OFF PID Gains"
      # "Flux ON/OFF CTRL Setpoint Sequence Logical"
      # "Increased buffer size to 100Mil on 1/1/2018"
      # "For 2 minutes"
      # "Calibrated Zero"
      # "PID Sampling interval, dt"
      # "Total Number of Samples"
      # "Note 1: Even though the parameters can be\nbrought into the loop \nand changed in real time. We want to avoid this\nNote 2: These parameters are for control in the linear range 0-175 GS absolute.\nFor non-linear range, you will need PID Gain Scheduling VI"
      # "Sample Rate (Hz or s^-1)\nor Step Duration (Each step is one second)"
      # "Offset by 1 removed \non 8/3/2017.\nIt solved problem. All\nData is there!"
      # "PS does not turn off unless two values are written."
      # "Maybe use it to replace the last value?"
      # "Removed Digital Trigger DAQmx and replaced\nwith real-time global variable before that"
      # "Flux Control Setpoint Sequence"
      n561 = Unbundle(w1376) -> ("proportional gain (Kc)"=w1375:dbl, "integral time (Ti, min)"=w1374:dbl, "derivative time (Td, min)"=w1373:dbl)
      n562 = Build Array "PID Parameters OFF"(w1375, w1374, w1373) -> (w1377:dbl[])
      n563 = Unbundle(w1371) -> ("proportional gain (Kc)"=w1407:dbl, "integral time (Ti, min)"=w1406:dbl, "derivative time (Td, min)"=w1405:dbl)
      n564 = Build Array "PID Parameters ON"(w1407, w1406, w1405, w1366, w1369) -> (w1404:dbl[])
      n565 = Reciprocal "Sample interval"(x=w1369) -> (1/x=w1408:dbl)
      n566 = shared-variable "NI-GenericDesktopPC-3A84958E\\Kopco PS Project Target Variables Library.lvlib\\PID Parameters OFF"(w1377) -> ()  [unwired: 1 in, 1 out]
      n567 = shared-variable "NI-GenericDesktopPC-3A84958E\\Kopco PS Project Target Variables Library.lvlib\\PID Parameters ON"(w1404) -> ()  [unwired: 1 in, 1 out]
      n568 = call-poly <vilib>:"DAQmx Create Timing Source.vi"("task/channels in"=w1416, "sleep time (us)"=1.0, "error in"=w1417) -> ("task out"=w1381:refnum<k21>, "timing source out"=w1355:string, "error out"=w1400:errorcluster)  [unwired: 10 in]
      n569 = Multiply "PID Sampling Interval, dt"(x=w1366, y=w1408) -> (x*y=w1403:dbl)
      n570 = Create Network Stream Writer Endpoint(7:100000000 ("writer buffer size"), 9:0.0 ("Double"), 11:"FluxWriter" ("writer name")) -> (0:w1392:errorcluster, 3:w1391:refnum<k21>)  [unwired: 4 in]
      n571 = Initialize Array "Initialize Array\nof samples to PID"(0.0 ("sleep time (us)"), w1366) -> (w1401:dbl[])
      n572 = shared-variable "NI-GenericDesktopPC-3A84958E\\Kopco PS Project Target Variables Library.lvlib\\Sensor Sensitivity Core"() -> (w1353:dbl)  [unwired: 1 in, 1 out]
      n573 = shared-variable "NI-GenericDesktopPC-3A84958E\\Kopco PS Project Target Variables Library.lvlib\\Sampling Rate"() -> (w1350:dbl)  [unwired: 1 in, 1 out]
      n574 = Array Size(array=w1409) -> (size(s)=w1410:i32)
      n575 = Divide(x=w1351, y=w1350) -> (x/y=→"Total seconds":dbl)
      n576 = Subtract(x=w1410, y=0) -> (x-y=w1402:i32)
      n577 = node-c288(w1355) -> (w1397:T3)  [unwired: 3 in]
      n578 = Quotient & Remainder(x=w1366, y=2) -> (floor(x/y)=w1361:i32)  [unwired: 1 out]
      n579 = timed-loop "Lower priority deterministic Code for Data Collection to Data Logger" {
        timing: w1397 -> [_]
        timing-out: [_] -> w1396
        tunnel: w1351 -> [w1428]
        tunnel: w1392 -> [w1440]
        tunnel: [w1429] -> w1386
        tunnel: [w1438] -> w1387
        tunnel: w1391 -> [w1439]
        shift-right: [w1427] -> _
        shift-left: -1 ("y") -> [w1430]
        tunnel: [w1419] -> _
        tunnel: w1350 -> [w1420]
        i -> [w1419]
        stop <- w1434 stop-if-true
        # "Switch OFF Null Flux currently running indicator. Placed in non-deterministic loop so as not to"
        # "Using variable bound\nto the toggle generate the error message\nthat remote endpoint is destroyed."
        n580 = node-c288() -> (w1426:errorcluster)  [unwired: 1 in]
        n581 = shared-variable ".\\Kopco PS Project Target Variables Library.lvlib\\Last Current AO"() -> (w1427:dbl)  [unwired: 1 in, 1 out]
        n582 = shared-variable ".\\Kopco PS Project Target Variables Library.lvlib\\Data RT Current"() -> (w1436:dbl)  [unwired: 1 in, 1 out]
        n583 = shared-variable ".\\Kopco PS Project Target Variables Library.lvlib\\Data RT Exposure"() -> (w1435:dbl)  [unwired: 1 in, 1 out]
        n584 = shared-variable ".\\Kopco PS Project Target Variables Library.lvlib\\Data RT Flux"() -> (w1437:dbl)  [unwired: 1 in, 1 out]
        n585 = Greater?(x=w1419, y=w1430) -> ()  [unwired: 1 out]
        n586 = shared-variable "NI-GenericDesktopPC-3A84958E\\Kopco PS Project Target Variables Library.lvlib\\Null Flux Running Middle"(FALSE ("Null Flux Running Middle")) -> ()  [unwired: 1 in, 1 out]
        n587 = Greater Or Equal?(x=w1419, y=w1428) -> (x >= y?=w1434:bool)
        n588 = Build Array(w1427, w1437, w1436, w1435) -> (w1433:dbl[])
        n589 = shared-variable-write(w1439, w1440, w1433) -> (w1438:refnum<k21>, w1429:errorcluster)  [unwired: 1 in, 1 out]
        n590 = Quotient & Remainder(x=w1419, y=10000) -> (x-y*floor(x/y)=w1424:i32)  [unwired: 1 out]
        n591 = Not(x=w1434) -> (.not. x?=w1432:bool)
        n592 = Equal To 0?(x=w1424) -> (x = 0?=w1423:bool)
        n593 = Equal?(x=w1419, y=w1419) -> (x = y?=w1421:bool)
        n594 = Or(x=w1421, y=w1423) -> (x .or. y?=w1422:bool)
        n595 = case shown="True" w1422 {
          tunnel: w1420 -> [_ w1443]
          tunnel: w1419 -> [_ w1442]
          frame False {
          }
          frame True {
            n596 = Divide(x=w1442, y=w1443) -> (x/y=→"Loop Index":dbl)
            "Loop Index" <- w1442
          }
        }
        n597 = shared-variable ".\\Kopco PS Project Target Variables Library.lvlib\\Data Upload"(w1432) -> ()  [unwired: 1 in, 1 out]
        n598 = node-c288(w1426) -> ()  [unwired: 1 out]
      }
      n599 = node-c288(w1355) -> (w1415:T3)  [unwired: 9 in]
      n600 = timed-loop "PID Control Loop" {
        tunnel: [w1507] -> _
        tunnel: w1413 -> [w1510]
        tunnel: [w1492] -> w1399
        tunnel: w1409 -> [w1508]
        timing: w1415 -> [_]
        timing-out: [_] -> w1414
        shift-right: [w1454] -> _
        shift-left: w1363 -> [w1485]
        shift-right: [w1504] -> _
        shift-left: w1401 -> [w1502]
        tunnel: w1401 -> [w1501]
        shift-right: [w1500] -> _
        shift-left: w1412 -> [w1499]
        tunnel: w1410 -> [w1503]
        tunnel: w1402 -> [_]
        tunnel: w1366 -> [w1483]
        tunnel: w1371 -> [w1489]
        tunnel: w1403 -> [w1495]
        tunnel: w1400 -> [w1494]
        tunnel: [w1493] -> w1384
        tunnel: [w1492] -> w1372
        tunnel: w1381 -> [w1491]
        tunnel: w1380 -> [w1490]
        tunnel: w1378 -> [w1488]
        tunnel: w1376 -> [w1487]
        tunnel: w1370 -> [w1486]
        tunnel: w1368 -> [w1484]
        shift-right: [w1481] -> _
        shift-left: w1367 -> [w1479]
        tunnel: w1361 -> [w1480]
        shift-right: [w1477] -> _
        shift-left: TRUE -> [w1476]
        tunnel: w1363 -> [w1475]
        shift-right: [w1473] -> _
        shift-left: w1363 -> [w1474]
        shift-right: [w1471] -> _
        shift-left: w1362 -> [w1472]
        tunnel: w1360 -> [w1470]
        tunnel: [w1467] -> w1358
        tunnel: "6. Keep Final Flux Running at End?" -> [w1466]
        tunnel: w1356 -> [w1459]
        tunnel: w1354 -> [w1458]
        tunnel: w1353 -> [w1457]
        i -> [w1455]
        stop <- w1468 continue-if-true
        # "Reversed order of AI7 & AI3 on 4/11/2018 to \nminimize leakage to Channel 7"
        # "No PID Control/DeGauss\nwhen control sequence is exceeded 3/31/2018"
        # "Stop this loop once data is uploaded"
        # "Calibrated Zero"
        # "AO_Null Flux"
        # "Rewrite to AO for now to see what it actually outputs.,  3/8/2018."
        # "AO last"
        # "AO"
        # "PID Sampling interval, dt"
        # "Number of samples pushed to PID\nper time"
        # "Current Flux\nSetpoint Value"
        # "Flux AI Reading"
        # "Array size"
        n601 = node-c288() -> ()  [unwired: 1 in, 1 out]
        n602 = Index Array "Current\nFlux Setpoint"(array=w1508, index=w1455) -> (element=w1506:dbl)
        n603 = Less Or Equal? "Less than 30 Samples"(x=w1499, y=w1483) -> (x <= y?=w1461:bool)
        n604 = call-poly <vilib>:"DAQmx Read.vi"("task/channels in"=w1491, "error in"=w1494) -> ("task out"=w1507:refnum<k21>, "data"=w1497:dbl[], "error out"=w1509:errorcluster)  [unwired: 11 in]
        n605 = Less Or Equal? "Less than 15 Samples"(x=w1479, y=w1480) -> (x <= y?=w1482:bool)
        n606 = Greater Or Equal? "Exceeded Datapoints?"(x=w1455, y=w1503) -> (x >= y?=w1460:bool)
        n607 = Delete From Array "AI5 Flux \nChannel"(array=w1497, index=1) -> (deleted portion=w1496:dbl)  [unwired: 1 in, 1 out]
        n608 = Delete From Array "AI7 Exposure\n Channel"(array=w1497, index=3) -> (deleted portion=w1456:dbl)  [unwired: 1 in, 1 out]
        n609 = Index Array "Mini-DeGauss \nON/OFF Status?"(array=w1486, index=w1455) -> (element=w1465:bool)
        n610 = case "DeGauss Sequence ON/OFF?" shown="False" w1465 {
          tunnel: w1506 -> [w1545 _]
          tunnel: w1485 -> [w1544 _]
          tunnel: [w1543 w1604] -> w1504
          tunnel: w1461 -> [w1520 _]
          tunnel: w1502 -> [w1542 w1603]
          tunnel: w1501 -> [w1541 w1602]
          tunnel: [w1523 w1606] -> w1500
          tunnel: w1499 -> [w1540 _]
          tunnel: w1496 -> [w1539 _]
          tunnel: w1495 -> [w1538 _]
          tunnel: [w1524 w1600] -> w1478
          tunnel: w1490 -> [w1537 _]
          tunnel: w1455 -> [w1527 w1594]
          tunnel: w1489 -> [w1536 _]
          tunnel: w1488 -> [w1535 _]
          tunnel: w1487 -> [w1534 _]
          tunnel: w1484 -> [_ w1601]
          tunnel: w1482 -> [_ w1599]
          tunnel: [w1533 w1598] -> w1481
          tunnel: w1479 -> [_ w1597]
          tunnel: [w1531 TRUE] -> w1477
          tunnel: w1476 -> [w1532 _]
          tunnel: w1475 -> [w1530 w1595]
          tunnel: [w1527 w1591] -> w1471
          tunnel: w1474 -> [w1522 w1593]
          tunnel: [w1528 w1590] -> w1473
          tunnel: w1472 -> [_ w1592]
          tunnel: w1470 -> [_ w1589]
          tunnel: w1460 -> [_ w1588]
          tunnel: w1460 -> [w1521 _]
          tunnel: w1459 -> [w1518 _]
          tunnel: w1458 -> [w1517 _]
          tunnel: w1457 -> [w1515 _]
          frame False {
            w1533 = 0  # Reset Mini DeGausss Sample Counter
            # "Update Last Current AO Index with \nCurrent Sample Index"
            # "Change the Magnitude\nof miniDeGauss:\nAbs(AO_nf) + Abs(AO_on,last) \nUse Max between that and the \ndifference. Difference will be\nminimal in OFF segments, but\nmaximal in ON segments."
            # "Loop Index"
            n611 = Index Array "Flux ON/OFF \nStatus?"(array=w1535, index=w1527) -> (element=w1526:bool)
            n612 = case "Control Sequence Exceeded?" shown="False" w1521 {
              tunnel: [w1546 TRUE] -> w1519
              tunnel: w1520 -> [w1546 _]
              frame False {
              }
              frame True {
                # "No PID Control"
              }
            }
            n613 = case "PID Gain Selector" shown="False" w1526 {
              tunnel: [w1556 w1558] -> w1514
              tunnel: w1536 -> [_ w1558]
              tunnel: w1534 -> [w1556 _]
              tunnel: w1518 -> [_ w1557]
              tunnel: w1517 -> [w1555 _]
              tunnel: [w1555 w1557] -> w1516
              frame False {
                # "Off Sequence"
              }
              frame True {
                # "ON Sequence"
              }
            }
            n614 = case "PID Control ON/OFF?" shown="True" w1519 {
              tunnel: w1538 -> [w1573 _]
              tunnel: w1545 -> [w1572 _]
              tunnel: [w1571 w1587] -> w1525
              tunnel: w1544 -> [_ w1587]
              tunnel: [w1578 w1585] -> w1543
              tunnel: w1542 -> [w1575 w1584]
              tunnel: w1541 -> [w1577 _]
              tunnel: [w1576 w1586] -> w1523
              tunnel: w1540 -> [_ w1583]
              tunnel: w1539 -> [_ w1582]
              tunnel: w1537 -> [w1564 _]
              tunnel: w1532 -> [w1569 w1581]
              tunnel: [FALSE w1581] -> w1531
              tunnel: w1530 -> [w1567 w1580]
              tunnel: [w1567 w1580] -> w1529
              tunnel: w1516 -> [w1566 _]
              tunnel: w1515 -> [w1563 _]
              tunnel: w1514 -> [_ _]
              frame False {
                w1576 = 0  # PID Sample Counter
                # "Offset was added to AO output\nby PID to eliminate the problem of\noutputing 0V for AO when there is \nlittle to no change in PV, which caused\na dip in response until PID recovers."
                # "Tried adding AO 0 to PID AO output. It works find with Null Flux, but \nnot with the anything where AO is not zero. It becomes like a run-away reaction. \nIt turns out that was because I added the indexed Flux value instead of the Null Flux AO.\nProblem Solved"
                # "flux setpoint"
                # "dt"
                # "Reset Array"
                n615 = call-poly <vilib>:"Mean.vi"("X"=w1575) -> ("mean"=w1565:dbl)  [unwired: 1 out]
                n616 = Subtract "PV-SP"(x=w1565, y=w1564) -> (x-y=w1561:dbl)
                n617 = Absolute Value(x=w1561) -> (abs(x)=w1559:dbl)
                n618 = Divide(x=w1559, y=w1563) -> (x/y=w1562:dbl)
                n619 = call-poly <vilib>:"PID Gain Schedule.vi"("PID gain schedule"=w1566, "gain scheduling value"=w1562) -> ("PID gains out"=w1560:T1)  [unwired: 2 in, 1 out]
                n620 = call-poly <vilib>:"PID.vi"("reinitialize? (F)"=w1569, "output range"=T6 {"Max/Min \ncontroller outputs"=10.0, "output low"=-10.0}, "dt (s)"=w1573, "PID gains"=w1560, "process variable"=w1561, "setpoint"=w1572) -> ("output"=w1570:dbl)  [unwired: 4 in, 1 out]
                n621 = Replace Array Subset "Reset Flux Array \nfed to PID"(array=w1575, new element=w1577, index=0) -> (w1578:dbl[])
                n622 = Add "Offset"(x=w1567, y=w1570) -> (x+y=w1571:dbl)
              }
              frame True {
                # "PID Sample Counter Index"
                # "AO last"
                # "Flux AI Reading"
                n623 = Increment "Increment\nto next\nindex"(x=w1583) -> (x+1=w1586:i32)
                n624 = Replace Array Subset "Replace ith item \nin Array fed to PID"(array=w1584, new element=w1582, index=w1583) -> (w1585:dbl[])
              }
            }
            n625 = case "Mini DeGauss Magnitude\nSelector" shown="False" w1526 {
              tunnel: w1529 -> [_ w1554]
              tunnel: [w1549 w1551] -> w1528
              tunnel: [w1548 w1550] -> w1524
              tunnel: w1525 -> [w1548 w1550]
              tunnel: w1522 -> [w1549 _]
              frame False {
              }
              frame True {
                n626 = Absolute Value "Abs[AO_on,last]"(x=w1550) -> (abs(x)=w1553:dbl)
                n627 = Absolute Value "Abs[AO_nf]"(x=w1554) -> (abs(x)=w1552:dbl)
                n628 = Add(x=w1553, y=w1552) -> (x+y=w1551:dbl)
              }
            }
          }
          frame True {
            w1606 = 0  # PID Sample Counter
            # "Leave Index unchanged\nDuring Mini DeGauss\nsequence"
            # "current sample index"
            # "Abs(AO_nf) + Abs(AO_on,last)"
            # "Null Flux AO"
            # "NO PID sequence. DeGaussing Sequence"
            n629 = case "Mini DeGauss Updated AO?" shown="True" w1599 {
              tunnel: w1601 -> [_ w1625]
              tunnel: [w1609 w1623] -> w1600
              tunnel: [w1611 w1624] -> w1598
              tunnel: w1597 -> [w1610 _]
              tunnel: w1594 -> [_ w1622]
              tunnel: w1595 -> [w1609 w1616]
              tunnel: w1593 -> [w1607 w1618]
              tunnel: w1592 -> [w1608 w1620]
              tunnel: [w1608 w1620] -> w1591
              tunnel: [w1607 w1619] -> w1590
              tunnel: w1589 -> [_ w1617]
              tunnel: w1588 -> [_ w1614]
              frame False {
                n630 = Increment "Increment\nto next\nindex"(x=w1610) -> (x+1=w1611:i32)
              }
              frame True {
                w1624 = 0  # Reset Mini DeGausss Sample Counter
                # "No PID Control/DeGauss\nwhen control sequence is exceeded 3/31/2018"
                # "Removed the offset\nand kept amplitude the same"
                # "Take the value once every 15 samples\nInitial curve is sampled at a lot more to \nminimize aliasing of the proper waveform"
                n631 = Index Array "Mini-DeGauss \nON/OFF Status?"(array=w1625, index=w1622) -> (element=w1615:dbl)
                n632 = Subtract "Reset"(x=w1622, y=w1620) -> (x-y=w1621:i32)
                n633 = Greater Or Equal? "Index of Cut off"(x=w1621, y=w1617) -> (x >= y?=w1612:bool)
                n634 = case "Control Sequence Exceeded?" shown="True" w1614 {
                  tunnel: [w1626 TRUE] -> w1613
                  tunnel: w1612 -> [w1626 _]
                  frame False {
                  }
                  frame True {
                    # "No PID Control"
                  }
                }
                n635 = case shown="True" w1613 {
                  tunnel: [w1629 w1631] -> w1623
                  tunnel: w1616 -> [_ w1631]
                  tunnel: w1615 -> [w1629 _]
                  tunnel: [w1628 w1630] -> w1619
                  tunnel: w1618 -> [w1628 w1630]
                  frame False {
                  }
                  frame True {
                  }
                }
              }
            }
            n636 = Replace Array Subset "Reset Flux Array \nfed to PID"(array=w1603, new element=w1602, index=0) -> (w1604:dbl[])
          }
        }
        n637 = shared-variable ".\\Kopco PS Project Target Variables Library.lvlib\\Data RT Exposure"(w1456) -> ()  [unwired: 1 in, 1 out]
        n638 = shared-variable ".\\Kopco PS Project Target Variables Library.lvlib\\Data RT Flux"(w1496) -> ()  [unwired: 1 in, 1 out]
        n639 = case shown="True" w1460 {
          tunnel: [w1633 w1635] -> w1454
          tunnel: w1478 -> [w1633 w1636]
          tunnel: [w1632 w1634] -> w1467
          tunnel: w1466 -> [w1632 w1634]
          frame False {
          }
          frame True {
            (unwired) FALSE ("y")
            # "A Toggle fixed the problem!"
            n640 = case shown="False" w1634 {
              tunnel: [0.0 ("output") w1638] -> w1635
              tunnel: w1636 -> [_ w1638]
              frame False {
                # "Reset AO at the end"
              }
              frame True {
                # "Keep Flux the same"
              }
            }
          }
        }
        n641 = shared-variable ".\\Kopco PS Project Target Variables Library.lvlib\\Last Current AO"(w1454) -> ()  [unwired: 1 in, 1 out]
        n642 = call-poly <vilib>:"DAQmx Write.vi"("task/channels in"=w1510, "data"=w1454, "error in"=w1509) -> ("task out"=w1492:refnum<k21>, "error out"=w1493:errorcluster)  [unwired: 10 in, 1 out]
        n643 = shared-variable ".\\Kopco PS Project Target Variables Library.lvlib\\Data RT Current"(w1454) -> ()  [unwired: 1 in, 1 out]
        n644 = case shown="False" w1460 {
          tunnel: [FALSE w1513] -> w1462
          frame False {
          }
          frame True {
            n645 = shared-variable ".\\Kopco PS Project Target Variables Library.lvlib\\Data Upload"() -> (w1512:bool)  [unwired: 1 in, 1 out]
            n646 = Not "No longer uploading"(x=w1512) -> (.not. x?=w1513:bool)
          }
        }
        n647 = Unbundle By Name(w1493) -> ("status"=w1469:bool)  [unwired: 2 out]
        n648 = Not(x=w1462) -> (.not. x?=w1463:bool)
        n649 = Not(x=w1469) -> (.not. x?=w1464:bool)
        n650 = And(x=w1464, y=w1463) -> (x .and. y?=w1468:bool)
        n651 = node-c288() -> ()  [unwired: 1 in, 1 out]
      }
      n652 = node-c288(w1396) -> (w1379:errorcluster)
      n653 = Flush Stream(8:w1386, 10:w1388, 11:w1387) -> (0:w1389:errorcluster, 3:w1390:refnum<k21>)  [unwired: 1 in, 1 out]
      n654 = Destroy Stream Endpoint(8:w1389, 11:w1390) -> (0:w1383:errorcluster)
      n655 = node-c288(w1414) -> (w1385:errorcluster)
      n656 = shared-variable "NI-GenericDesktopPC-3A84958E\\Kopco PS Project Target Variables Library.lvlib\\Null Flux Running End"(w1358) -> ()  [unwired: 1 in, 1 out]
      n657 = Merge Errors(w1385, w1384, w1379, w1383) -> (w1382:errorcluster)
      "# of Data Points" <- w1351
    }
    frame #21 {
      # "Bound to \"Null Flux Running End\""
      n658 = call <vilib>:"DAQmx Stop Task.vi"("task/channels in"=w1647, "error in"=w1646) -> ("task out"=w1653:refnum<k21>, "error out"=w1652:errorcluster)  [unwired: 12 in]
      n659 = call <vilib>:"DAQmx Clear Task.vi"("task in"=w1653, "error in"=w1652) -> ("error out"=w1649:errorcluster)  [unwired: 13 in]
      n660 = call <vilib>:"DAQmx Stop Task.vi"("task/channels in"=w1648, "error in"=w1649) -> ("task out"=w1651:refnum<k21>, "error out"=w1650:errorcluster)  [unwired: 12 in]
      n661 = call <vilib>:"DAQmx Clear Task.vi"("task in"=w1651, "error in"=w1650) -> ()  [unwired: 13 in, 1 out]
    }
  }
